vi "Results_file_Plotter.vi"() -> ()   [LabVIEW 2012]
uses:
  Anemometry/Anemometry Sub Vis/Data_plotting_vis/Plot_Slice.ctl
  Anemometry/Anemometry Sub Vis/Data_plotting_vis/Plotter_Mode.ctl
  Anemometry/Anemometry Sub Vis/Data_plotting_vis/Data_File_Type.ctl
  Anemometry/Anemometry Sub Vis/File/Setup_Filetype.ctl
  Anemometry/Anemometry Sub Vis/Controls/Global_mode.ctl
  Anemometry/Anemometry Sub Vis/Data_plotting_vis/Results_plotter_Global.vi
  Anemometry/Anemometry Sub Vis/Globals/Trav_pos_global.vi
  Instance           1 28Saved   Results_file_Plotter .vi
  Anemometry/Anemometry Sub Vis/Globals/Constants_global.vi
panel:
  out "Edit Raw DF?":bool
  in  "Tab Control":T1(tab)=enum."Save "
  in  "Template":path
  in  "Empty":bool
  in  "Result files to read":path[](array[path])
  in  "Add results file":bool
  in  "File Types to Read":T2
  in  "Vector Plot?":bool
  in  "Ordinate Name":string
  out "2nd Add label":string
  out "First Add label":string
  in  "Additional X Values":dbl[](array[numeric]) format="%.2f"
  in  "Additional Y Values":dbl[](array[numeric]) format="%.2f"
  in  "Show Results Space Analysis":bool
  in  "Show Plot Space Analysis":bool
  in  "Multi Ordinate":i32[](listbox)
  in  "Multi Ordinate?":bool
  in  "Ordinate":u16(ring) items=["Case", "File", "Source_Position X (mm)", "Receptor X (mm)", "Receptor Y (mm)", "Receptor Z (mm)", "C (ppm)", "c^2", "Q l/min", "CU/Q (m^{-2})", "Uref (m/s)", "Multi Run Start Time", "Bkgnd FF (C)", "Bkgnd Variance FF (C)", "Seconds since 1st Jan", "CU/Q Max Lat", "CU/Q Sig Y", "CU/Q Yo", "FF (C) Standard Error in Mean", "CU/Q Err", "Q Trace", "Drift%", "t (min)", "EnFlo Lab labstrat1 Delta T", "GMU Carrier 2 Gas", "Gas", "Source ID (mm)", "Emission Velocity m/s", "Emission Ratio", "FF (C) Standard Error in Variance", "GMU Source Type", "Aero_Tunnel Speed Meas Velocity", "Raw Data Filename", "Multi Run Row Number", "LDA X (mm)", "LDA Y (mm)", "LDA Z (mm)", "U", "u^2", "LDA (U) Standard Error in Mean", "W", "w^2", "LDA (W) Standard Error in Mean", "uw", "Av LDA Sampling Rate", "LDA (U) Standard Error in Variance", "u^2/U_{ref}^2", "w^2/U_{ref}^2", "-uw/U_{ref}^2", "U/Uref", "W/Uref", "LDA (U) & FF (C) Correlation uc", "LDA (W) & FF (C) Correlation wc", "Multi Run Row Type", "CU/Q (m^{-2}) Max Lat", "CU/Q (m^{-2}) Sig Y", "CU/Q (m^{-2}) Yo"]
  in  "Intensity Plot?":bool
  in  "Absisca":u16(ring) items=["Case", "File", "Source_Position X (mm)", "Receptor X (mm)", "Receptor Y (mm)", "Receptor Z (mm)", "C (ppm)", "c^2", "Q l/min", "CU/Q (m^{-2})", "Uref (m/s)", "Multi Run Start Time", "Bkgnd FF (C)", "Bkgnd Variance FF (C)", "Seconds since 1st Jan", "CU/Q Max Lat", "CU/Q Sig Y", "CU/Q Yo", "FF (C) Standard Error in Mean", "CU/Q Err", "Q Trace", "Drift%", "t (min)", "EnFlo Lab labstrat1 Delta T", "GMU Carrier 2 Gas", "Gas", "Source ID (mm)", "Emission Velocity m/s", "Emission Ratio", "FF (C) Standard Error in Variance", "GMU Source Type", "Aero_Tunnel Speed Meas Velocity", "Raw Data Filename", "Multi Run Row Number", "LDA X (mm)", "LDA Y (mm)", "LDA Z (mm)", "U", "u^2", "LDA (U) Standard Error in Mean", "W", "w^2", "LDA (W) Standard Error in Mean", "uw", "Av LDA Sampling Rate", "LDA (U) Standard Error in Variance", "u^2/U_{ref}^2", "w^2/U_{ref}^2", "-uw/U_{ref}^2", "U/Uref", "W/Uref", "LDA (U) & FF (C) Correlation uc", "LDA (W) & FF (C) Correlation wc", "Multi Run Row Type", "CU/Q (m^{-2}) Max Lat", "CU/Q (m^{-2}) Sig Y", "CU/Q (m^{-2}) Yo"]
  in  "Job Directory":path
  in  "Save Averaged rows":bool
  in  "Save Surface Fit":bool
  in  "Output Filename":path
  in  "Save Data in Rows":bool
  in  "Save Plot data":bool
  in  "Header":string
  in  "Process Point":bool
  in  "Kill Point":bool
  out "Table":string[][](table)
  in  "Post Process Plotted Data":bool
  in  "...using routine":string
  in  "Calculate new metadata":bool
  in  "Add /Edit metadata":bool
  in  "Delete Plotted data from file":bool
  in  "Save Setup":bool
  in  "Load Setup":bool
  in  "stop":bool
  out "Current":string="Graph Scales"
  in  "Single Series":i32[](listbox)=[0]
  in  "Edit Template File":bool
  in  "color and symbol":bool
  out "nRows":i32
  in  "Filter Bins 2":i32[](listbox)=[0]
  in  "Filter 6":u16(ring)
  in  "Filter 5":u16(ring)
  in  "Filter 4":u16(ring) items=["Show All (25)", "Lateral Profile (11)", "Vertical Profile (14)", "NOT Lateral Profile (14)", "NOT Vertical Profile (11)"]
  in  "Filter 3":u16(ring) items=["Show All (11)", "1 (11)", "NOT 1 (0)"]
  in  "Filter Array":u16[](array[ring])=[0, 0, 0, 0, 0, 0] items=["Don't Filter", "Case", "File", "Source_Position X (mm)", "Receptor X (mm)", "Receptor Y (mm)", "Receptor Z (mm)", "C (ppm)", "c^2", "Q l/min", "CU/Q (m^{-2})", "Uref (m/s)", "Multi Run Start Time", "Bkgnd FF (C)", "Bkgnd Variance FF (C)", "Seconds since 1st Jan", "CU/Q Max Lat", "CU/Q Sig Y", "CU/Q Yo", "FF (C) Standard Error in Mean", "CU/Q Err", "Q Trace", "Drift%", "t (min)", "EnFlo Lab labstrat1 Delta T", "GMU Carrier 2 Gas", "Gas", "Source ID (mm)", "Emission Velocity m/s", "Emission Ratio", "FF (C) Standard Error in Variance", "GMU Source Type", "Aero_Tunnel Speed Meas Velocity", "Raw Data Filename", "Multi Run Row Number", "LDA X (mm)", "LDA Y (mm)", "LDA Z (mm)", "U", "u^2", "LDA (U) Standard Error in Mean", "W", "w^2", "LDA (W) Standard Error in Mean", "uw", "Av LDA Sampling Rate", "LDA (U) Standard Error in Variance", "u^2/U_{ref}^2", "w^2/U_{ref}^2", "-uw/U_{ref}^2", "U/Uref", "W/Uref", "LDA (U) & FF (C) Correlation uc", "LDA (W) & FF (C) Correlation wc", "Multi Run Row Type", "CU/Q (m^{-2}) Max Lat", "CU/Q (m^{-2}) Sig Y", "CU/Q (m^{-2}) Yo"]
  in  "Filter Bins 1":i32[](listbox)=[0]
  in  "Create picture Vi Name":string caption="Picture VI:"
  in  "Save Plot as jpg":bool
  in  "Reload Files":bool
  out "Warning!":string
  out "XY Plot":cluster{dbl[], dbl[]}[](graph)
  out "Edit Raw Data Header Info":bool
  out "Raw DF in Orig Pos?":bool
  out "Intensity Graph":dbl[][](graph)
  in  "Bkgnd Value":dbl
  in  "Update":bool
  in  "Plot Resolution":bool
  in  "Point Size":i32(slide)=1 scale=0.0..10.0
  in  "No of Contours":i32=20
  in  "Slice mode":T3
  in  "Z Ch Name":u16(ring) items=["Case", "File", "Source_Position X (mm)", "Receptor X (mm)", "Receptor Y (mm)", "Receptor Z (mm)", "C (ppm)", "c^2", "Q l/min", "CU/Q (m^{-2})", "Uref (m/s)", "Multi Run Start Time", "Bkgnd FF (C)", "Bkgnd Variance FF (C)", "Seconds since 1st Jan", "CU/Q Max Lat", "CU/Q Sig Y", "CU/Q Yo", "FF (C) Standard Error in Mean", "CU/Q Err", "Q Trace", "Drift%", "t (min)", "EnFlo Lab labstrat1 Delta T", "GMU Carrier 2 Gas", "Gas", "Source ID (mm)", "Emission Velocity m/s", "Emission Ratio", "FF (C) Standard Error in Variance", "GMU Source Type", "Aero_Tunnel Speed Meas Velocity", "Raw Data Filename", "Multi Run Row Number", "LDA X (mm)", "LDA Y (mm)", "LDA Z (mm)", "U", "u^2", "LDA (U) Standard Error in Mean", "W", "w^2", "LDA (W) Standard Error in Mean", "uw", "Av LDA Sampling Rate", "LDA (U) Standard Error in Variance", "u^2/U_{ref}^2", "w^2/U_{ref}^2", "-uw/U_{ref}^2", "U/Uref", "W/Uref", "LDA (U) & FF (C) Correlation uc", "LDA (W) & FF (C) Correlation wc", "Multi Run Row Type", "CU/Q (m^{-2}) Max Lat", "CU/Q (m^{-2}) Sig Y", "CU/Q (m^{-2}) Yo"]
  in  "Y Ch Name":u16(ring) items=["Case", "File", "Source_Position X (mm)", "Receptor X (mm)", "Receptor Y (mm)", "Receptor Z (mm)", "C (ppm)", "c^2", "Q l/min", "CU/Q (m^{-2})", "Uref (m/s)", "Multi Run Start Time", "Bkgnd FF (C)", "Bkgnd Variance FF (C)", "Seconds since 1st Jan", "CU/Q Max Lat", "CU/Q Sig Y", "CU/Q Yo", "FF (C) Standard Error in Mean", "CU/Q Err", "Q Trace", "Drift%", "t (min)", "EnFlo Lab labstrat1 Delta T", "GMU Carrier 2 Gas", "Gas", "Source ID (mm)", "Emission Velocity m/s", "Emission Ratio", "FF (C) Standard Error in Variance", "GMU Source Type", "Aero_Tunnel Speed Meas Velocity", "Raw Data Filename", "Multi Run Row Number", "LDA X (mm)", "LDA Y (mm)", "LDA Z (mm)", "U", "u^2", "LDA (U) Standard Error in Mean", "W", "w^2", "LDA (W) Standard Error in Mean", "uw", "Av LDA Sampling Rate", "LDA (U) Standard Error in Variance", "u^2/U_{ref}^2", "w^2/U_{ref}^2", "-uw/U_{ref}^2", "U/Uref", "W/Uref", "LDA (U) & FF (C) Correlation uc", "LDA (W) & FF (C) Correlation wc", "Multi Run Row Type", "CU/Q (m^{-2}) Max Lat", "CU/Q (m^{-2}) Sig Y", "CU/Q (m^{-2}) Yo"]
  in  "X Ch Name":u16(ring) items=["Case", "File", "Source_Position X (mm)", "Receptor X (mm)", "Receptor Y (mm)", "Receptor Z (mm)", "C (ppm)", "c^2", "Q l/min", "CU/Q (m^{-2})", "Uref (m/s)", "Multi Run Start Time", "Bkgnd FF (C)", "Bkgnd Variance FF (C)", "Seconds since 1st Jan", "CU/Q Max Lat", "CU/Q Sig Y", "CU/Q Yo", "FF (C) Standard Error in Mean", "CU/Q Err", "Q Trace", "Drift%", "t (min)", "EnFlo Lab labstrat1 Delta T", "GMU Carrier 2 Gas", "Gas", "Source ID (mm)", "Emission Velocity m/s", "Emission Ratio", "FF (C) Standard Error in Variance", "GMU Source Type", "Aero_Tunnel Speed Meas Velocity", "Raw Data Filename", "Multi Run Row Number", "LDA X (mm)", "LDA Y (mm)", "LDA Z (mm)", "U", "u^2", "LDA (U) Standard Error in Mean", "W", "w^2", "LDA (W) Standard Error in Mean", "uw", "Av LDA Sampling Rate", "LDA (U) Standard Error in Variance", "u^2/U_{ref}^2", "w^2/U_{ref}^2", "-uw/U_{ref}^2", "U/Uref", "W/Uref", "LDA (U) & FF (C) Correlation uc", "LDA (W) & FF (C) Correlation wc", "Multi Run Row Type", "CU/Q (m^{-2}) Max Lat", "CU/Q (m^{-2}) Sig Y", "CU/Q (m^{-2}) Yo"]
  in  "Resolution":dbl=1.0 min=0.0 format="%.4f"
  out "Surface Area":dbl format="%^_6g"
  out "Surface Integral":dbl format="%^_6g"
  out "Surface Average":dbl format="%^#.6g"
  out "Uadvec":dbl
  in  "Full_Res_Results_Folder":path
  out "Last used Template":path
  out "Cursor index":i32
  out "Choosen Path":path
  in  "VI Refnum Calculation":refnum<vi>
  out "Filetype":string[](array[string])
  out "Mode":T4
  out "Plotted rows only?":bool
  in  "type specifier VI Refnum (for type only) 2":refnum<vi>
  in  "type specifier VI Refnum (for type only)":refnum<vi>
  out "Accept Array":bool[][](array[boolean])
  out "Previous slice mode":T3
  out "Slice mode Change?":bool
  out "Non-Blank Rows":bool[](array[boolean])
  out "File Index":i32
  out "Tolerances":dbl[](array[numeric]) format="%.2f"
  in  "Results files choosen":path[](array[path])
  in  "Transpose":bool
  out "Plotted Series":bool[][](array[boolean])
  in  "Results file":path
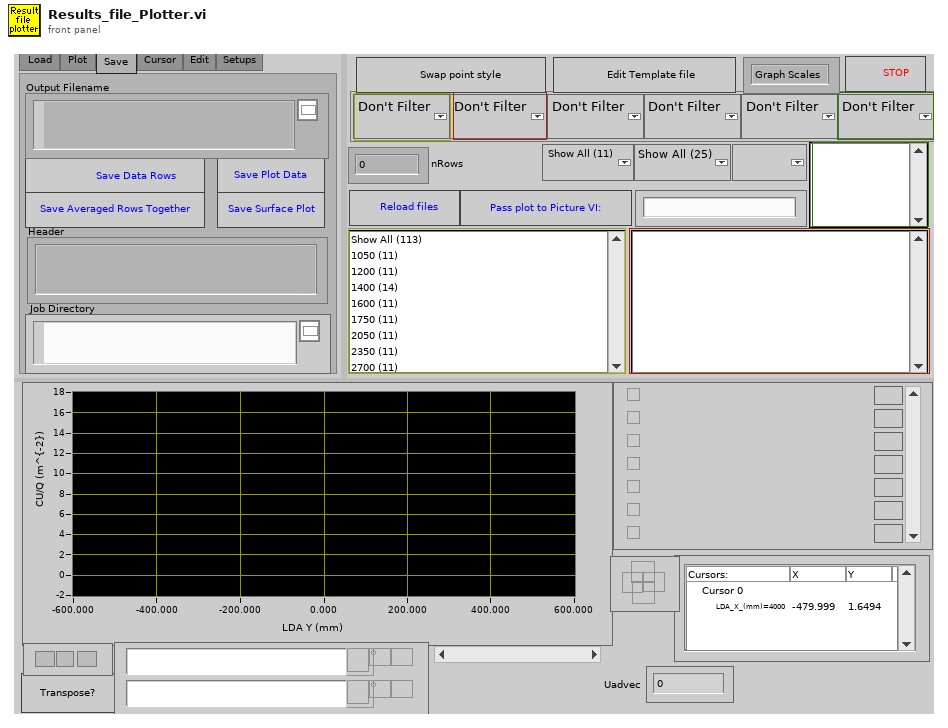
[diagram p1: front panel]
types:
  T1 = enum32{"Load ", "Plot ", "Save ", "Cursor", "Edit", "Setups"}
  T2 = typedef "Data_File_Type.ctl" = enum16{"Read All File Types", "Results Files Only", "Raw Data Files Only", "Calibration Files Only", "Gas Desk Files Only", "Old Results Files Only", "Tabulated Data Files Only"}
  T3 = typedef "Plot_Slice.ctl" = enum16{"XY Slice (Plan)", "YX Slice (Plan)", "YZ Slice (Cross)", "ZY Slice (Cross)", "XZ Slice (Side)", "ZX Slice (Side)"}
  T4 = typedef "Plotter_Mode.ctl" = enum16{"Save file", "Delete unwanted rows", "Edit Values with constants", "Edit values per row", "Edit Raw Data file header", "Post Process Plotted Rows"}
  T5 = typedef "Setup_Filetype.ctl" = enum16{"Measurement Setups", "Calibration Setups", "General", "Results File Plotter Setups", "Speed Calib Tweaks"}
  T6 = enum16{"Zero or one", "One", "Zero or more", "One or more"}
  T7 = typedef "Global_mode.ctl" = enum16{"Read Global", "Load Global From File", "Write Global to File"}
  T8 = enum16{"Edit Existing Template File", "Create New Template File"}
  T9 = enum16{"Show only data summary", "Show data summary", "No data summary"}
  T10 = typedef "All_Setup.ctl" = cluster{"Result files to read":path[], "Template":path, "Transpose":bool, "Additional X Values":dbl[], "Additional Y Values":dbl[], "Ordinate":u16, "Absisca":u16, "Filter Array":u16[], "color and symbol":bool, "Output Filename":path, "Jpg Vi Name":string, "Intensity Plot?":bool, "Multi Ordinate?":bool, "Filter Bins 1":i32[], "Filter Bins 2":i32[], "Multi Ordinate":i32[]}
  T11 = enum16{"Left Button", "Center Button", "Right Button", "Window Close"}
  T12 = enum32{"existing file", "new file", "new or existing file", "existing dir", "new dir", "new or existing dir", "existing file (use LLBs)", "new file (use LLBs)", "new or existing file (use LLBs)", "new or existing file or directory (use LLBs)"}
  T13 = cluster{"Plot Color":u32, "Plot Interpolation":u8, "Point Style":u8, "Line Style":u8, "Fill/Pt. Color":u32, "Line Width":u8, "Bar Plot Style":u8, "Fill To":i16}[]
  T14 = typedef "Group_Binning.ctl" = cluster{"Index":i32, "Tolerance":dbl, "Precision":string}
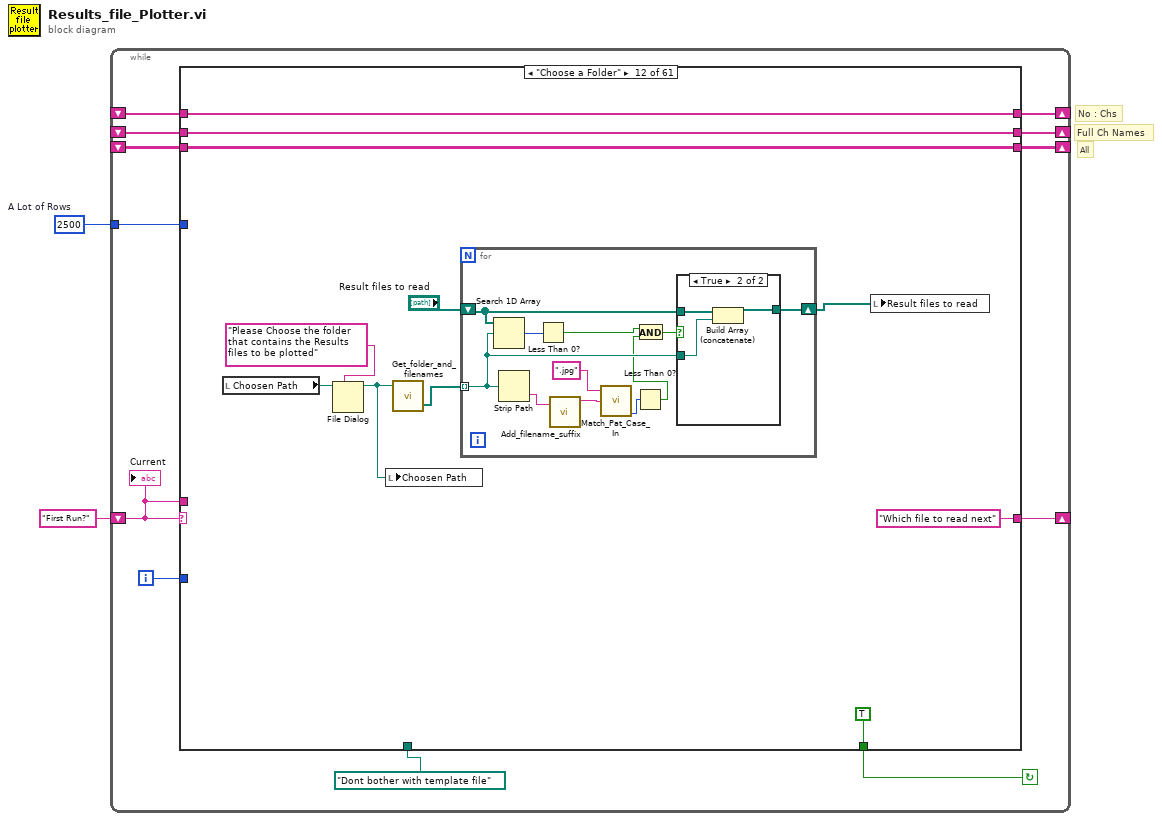
[diagram p0: block diagram]
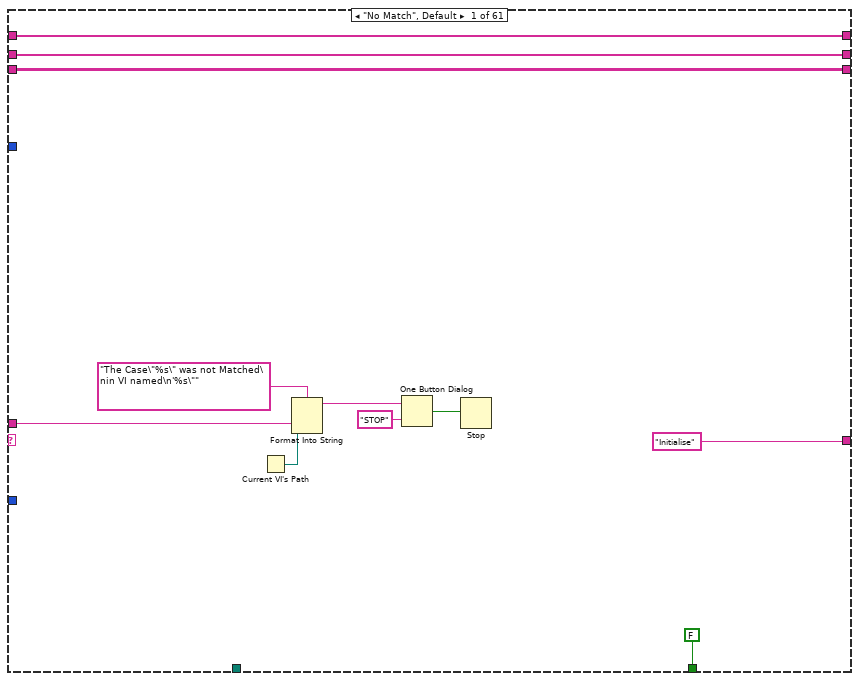
[diagram p2: hidden frame]
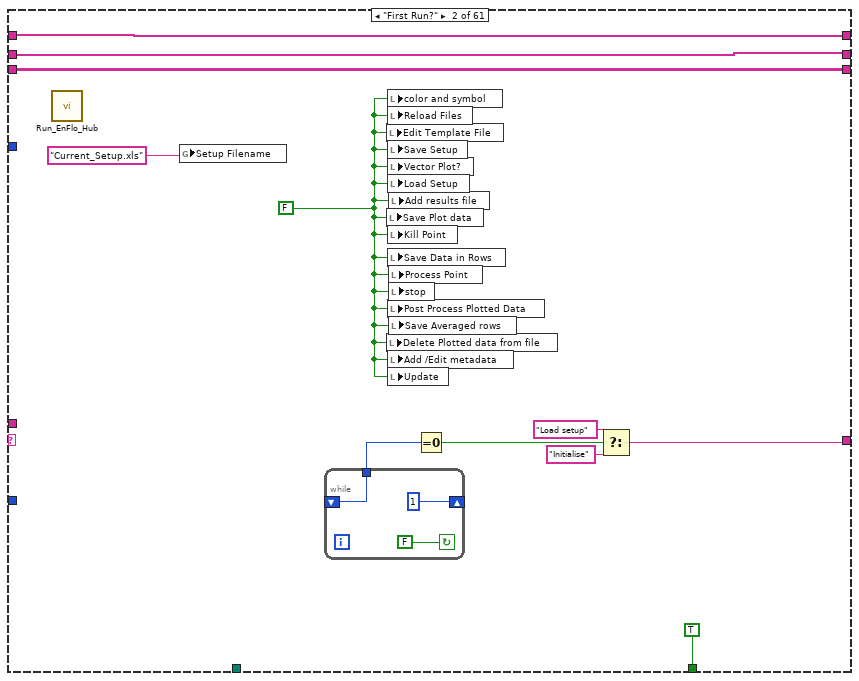
[diagram p3: hidden frame]
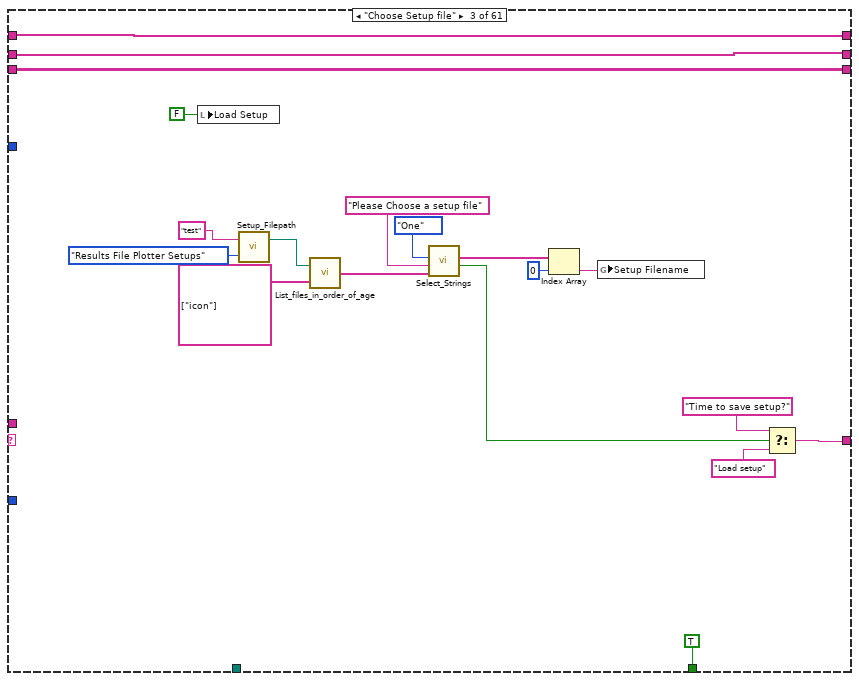
[diagram p4: hidden frame]
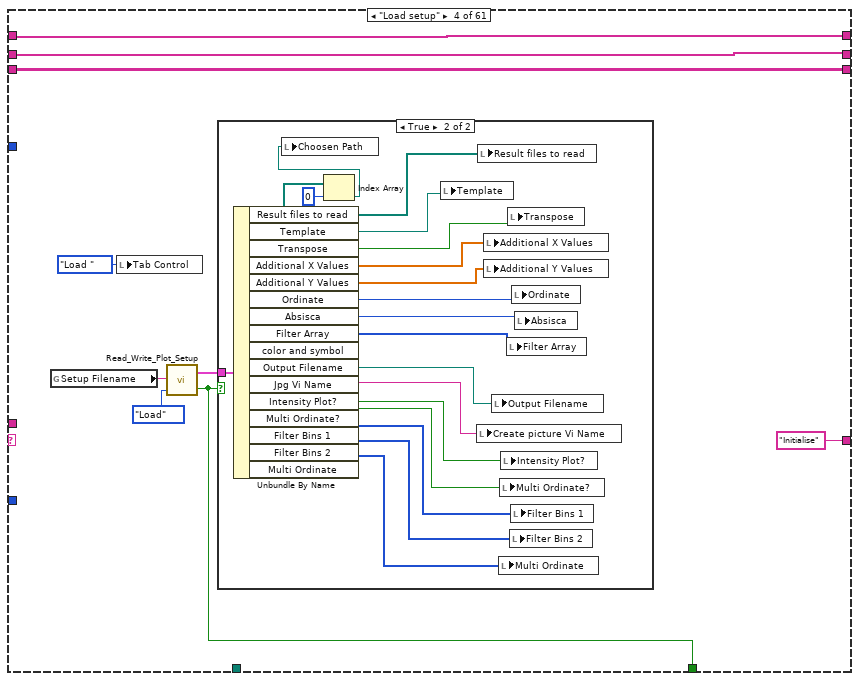
[diagram p5: hidden frame]
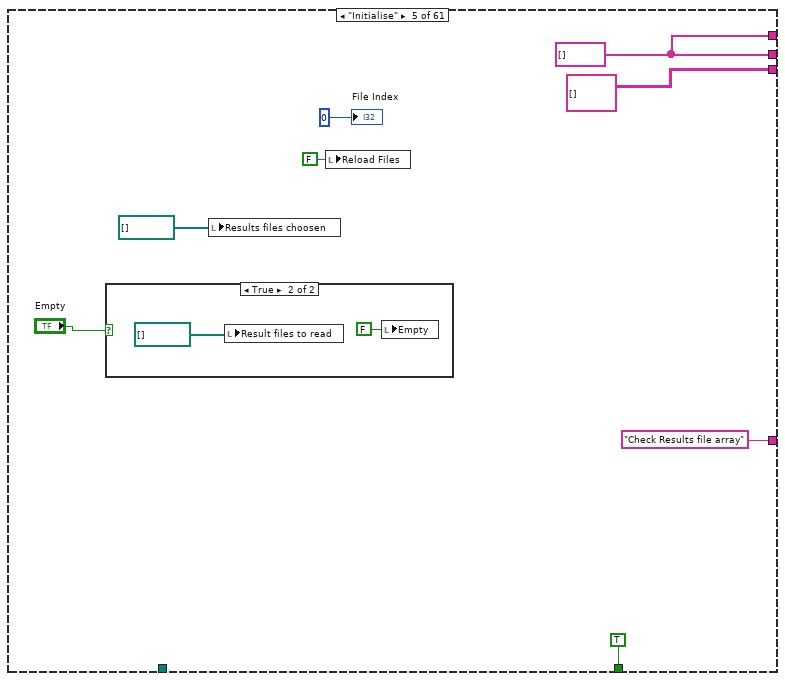
[diagram p7: hidden frame]
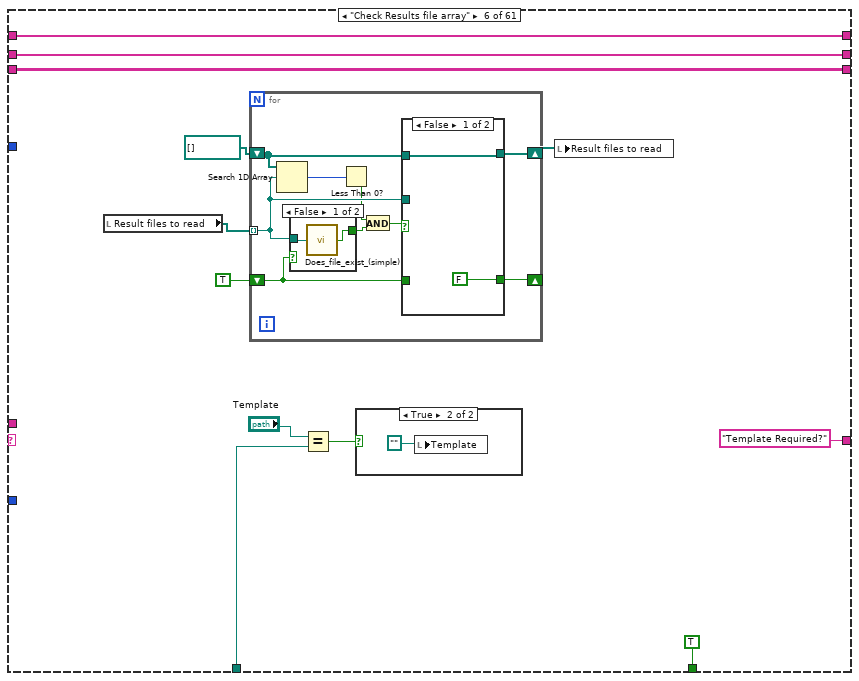
[diagram p9: hidden frame]
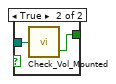
[diagram p11: hidden frame]
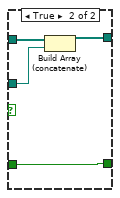
[diagram p12: hidden frame]
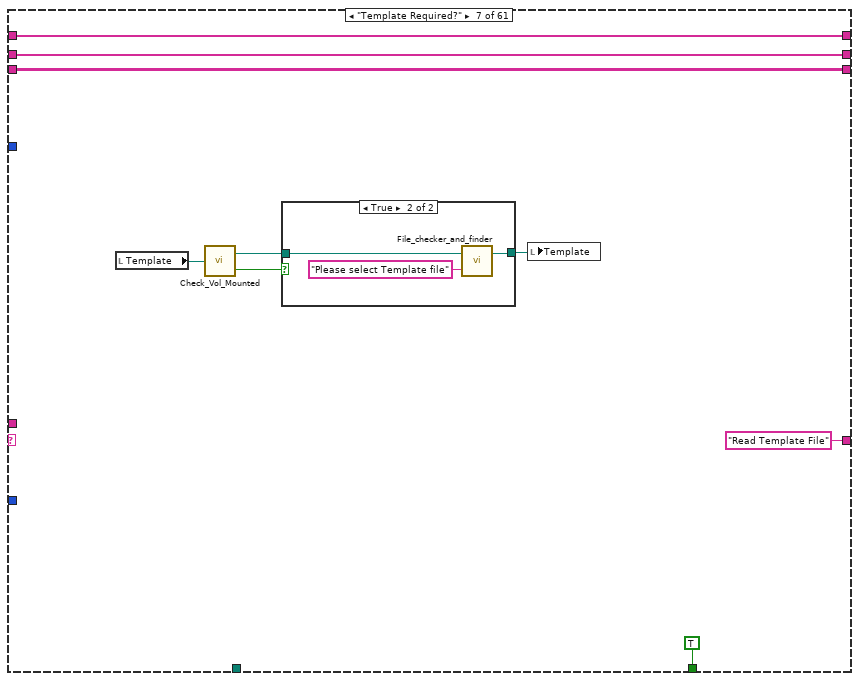
[diagram p13: hidden frame]
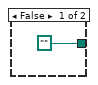
[diagram p14: hidden frame]
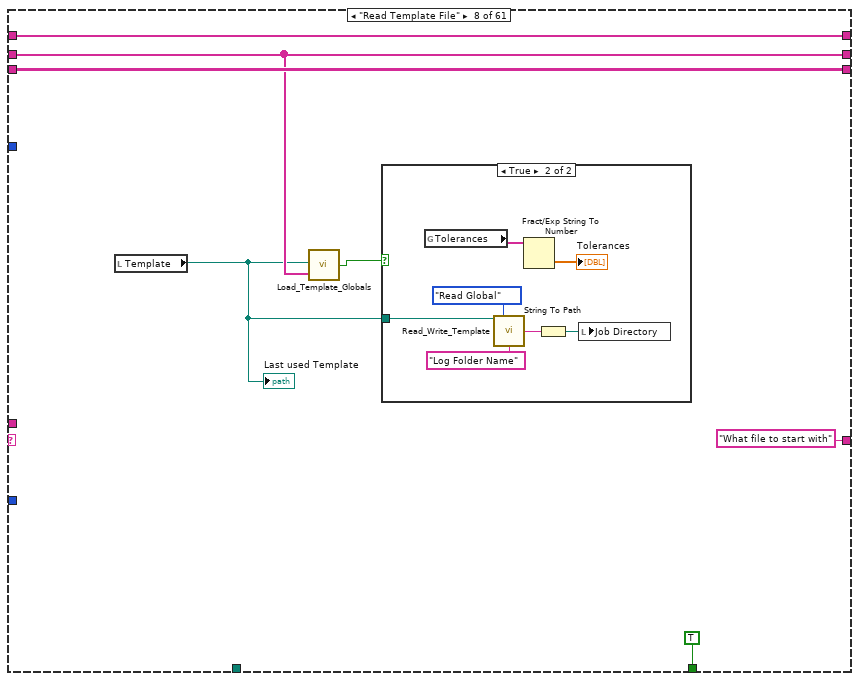
[diagram p15: hidden frame]
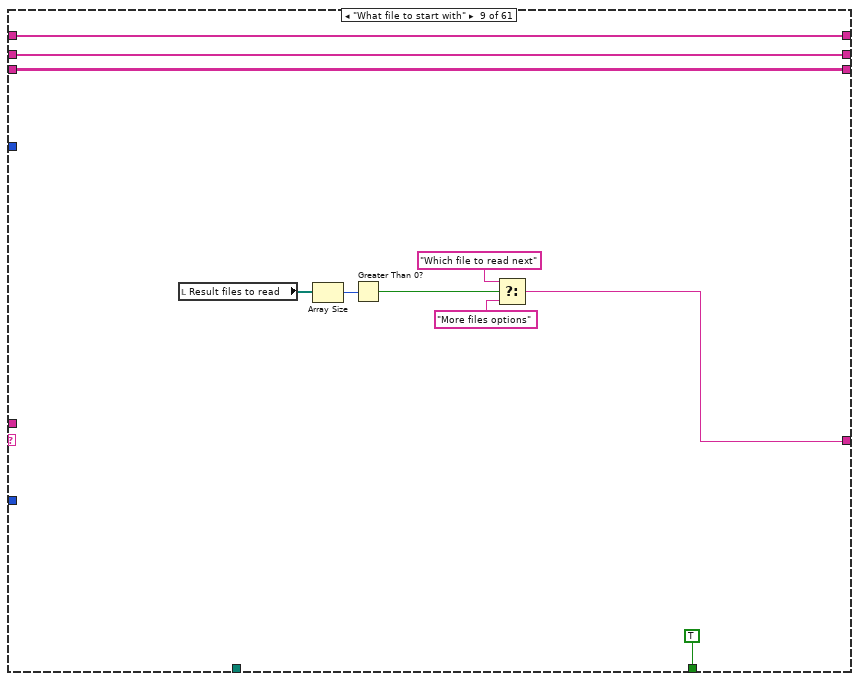
[diagram p17: hidden frame]
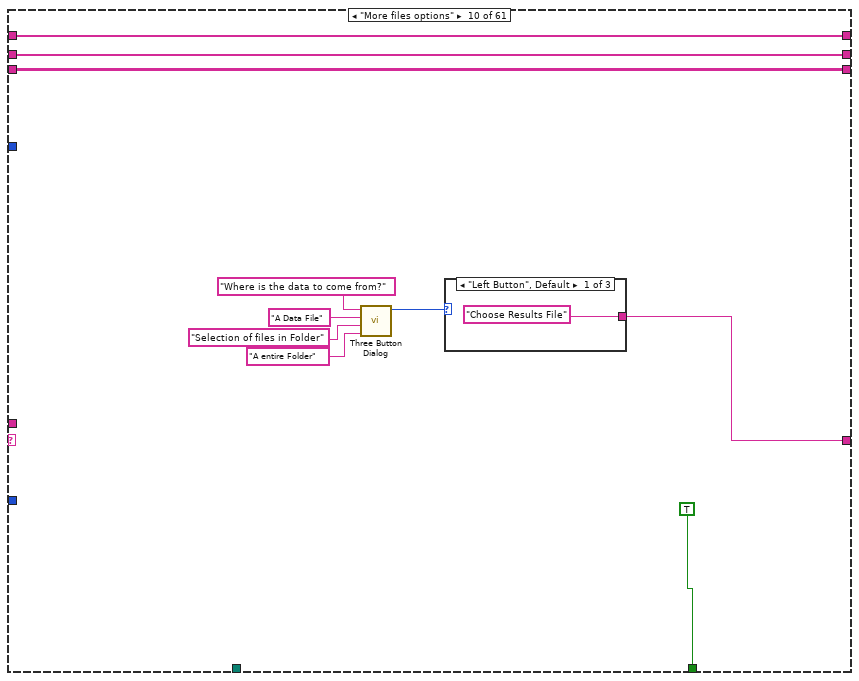
[diagram p18: hidden frame]
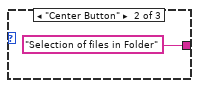
[diagram p19: hidden frame]
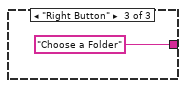
[diagram p20: hidden frame]
diagram:
  w1 = 2500  # A Lot of Rows
  # "No : Chs"
  # "Full Ch Names"
  # "All"
  n1 = while {
    shift-left: _ -> [w7]
    shift-right: [w8] -> _
    shift-left: "First Run?" -> [w11]
    shift-right: [w4] -> _
    shift-left: _ -> [w9]
    shift-right: [w14] -> _
    shift-left: _ -> [w12]
    shift-right: [w5] -> _
    tunnel: w1 -> [w3]
    i -> [w6]
    stop <- w13 continue-if-true
    n2 = case shown="\"Choose a Folder\"" w11 {
      tunnel: w9 -> [w25 w35 w57 w65 _ w106 w134 w143 w164 w174 w186 w200 w231 w258 w281 w403 w425 w451 w476 w502 w556 w570 w607 w909 w978 w1033 w1058 w1077 w1163 w1214 w1244 w1533 w1549 w1570 w1599 w1663 w1696 w1771 w1794 w1809 w1873 w1925 w1951 w2160 w2172 w2198 w2324 w2468 w2502 w2517 w2542 w2569 w2612 w2630 w2673 w2776 w2809 w3164 w3179 w3215 w3223]
      tunnel: [w25 w35 w57 w65 w91 w106 w134 w143 w164 w174 w186 w200 w231 w258 w279 w403 w425 w451 w476 w502 w556 w570 w607 w909 w978 w1033 w1058 w1077 w1163 w1214 w1242 w1533 w1549 w1570 w1599 w1663 w1696 w1771 w1794 w1809 w1873 w1925 w1949 w2160 w2172 w2196 w2317 w2468 w2502 w2517 w2542 w2569 w2612 w2630 w2673 w2776 w2809 w3164 w3179 w3215 w3223] -> w14
      tunnel: ["Initialise" w28 w52 "Initialise" ("t") "Check Results file array" ("t") "Template Required?" "Read Template File" "What file to start with" w155 w170 "Which file to read next" "Which file to read next" "Which file to read next" w254 w276 w394 "What is present?" "Ordinate Selector Type" w473 "Which rows are Non-Blank?" w549 "Create Selectors" w596 "Re Plot Data?" w973 "Prepare Filter2 strings" "Plot Data" w1074 "Add Axis names" "Analyse Plot Space" w1245 "What to do next?" "What to do next?" ("t") w1556 w1592 w1641 w1694 w1765 w1790 w1808 w1872 "Initialise" w1952 w2151 "Create Selectors" w2199 w2325 w2466 w2500 w2507 w2526 "Save XY plot as jpg" "Create Selectors" w2627 w2676 w2760 w2815 "Save Setup" ("t") "Initialise" ("t") w3184 "Time to save setup?"] -> w4
      tunnel: [FALSE TRUE TRUE w61 TRUE TRUE TRUE TRUE TRUE TRUE TRUE TRUE TRUE w249 w283 TRUE TRUE TRUE TRUE TRUE TRUE TRUE TRUE TRUE TRUE TRUE TRUE w1075 TRUE TRUE w1246 TRUE TRUE ("OK?") TRUE TRUE ("OK?") TRUE ("OK?") w1692 TRUE TRUE w1807 w1871 TRUE w1953 TRUE ("OK?") TRUE ("OK?") w2200 w2326 TRUE TRUE TRUE TRUE TRUE TRUE TRUE TRUE TRUE TRUE TRUE TRUE w3193 TRUE ("OK?")] -> w13
      tunnel: w12 -> [w24 w34 w56 w64 _ w105 w133 w145 w163 w173 w185 w199 w230 w257 w282 w399 w424 w452 w477 w503 w555 w568 w602 w911 w967 w1035 w1060 w1076 w1165 w1216 w1243 w1532 w1548 w1569 w1610 w1662 w1695 w1770 w1793 w1806 w1870 w1924 w1950 w2159 w2169 w2197 w2323 w2469 w2501 w2516 w2546 w2572 w2611 w2629 w2672 w2775 w2808 w3163 w3178 w3214 w3222]
      tunnel: w11 -> [w16 _ _ _ _ _ _ _ _ _ _ _ _ _ _ _ _ _ _ _ _ _ _ _ _ _ _ _ _ _ _ _ _ _ _ _ _ _ _ _ _ _ _ _ _ _ _ _ _ _ _ _ _ _ _ _ _ _ _ _ _]
      tunnel: path "Dont bother with template file" ("Template File") -> [_ _ _ _ _ w99 _ _ _ _ _ _ _ _ _ _ _ _ _ _ _ _ _ _ _ _ _ _ _ _ _ _ _ _ _ _ _ _ _ _ _ _ _ _ _ _ _ _ _ _ _ _ _ _ _ _ _ w3161 w3173 _ _]
      tunnel: [w15 w33 w55 w66 w91 w104 w132 w144 w161 w171 w183 w197 w228 w256 w278 w387 w423 w453 w475 w501 w547 w569 w600 w908 w969 w1026 w1053 w1073 w1157 w1209 w1238 w1529 w1550 w1568 w1600 w1664 w1697 w1769 w1792 w1805 w1869 w1923 w1943 w2161 w2177 w2187 w2320 w2478 w2503 w2518 w2543 w2570 w2613 w2631 w2677 w2777 w2816 w3165 w3180 w3216 w3224] -> w8
      tunnel: w7 -> [w15 w33 w55 w66 _ w104 w132 w144 w161 w171 w183 w197 w228 w256 w277 w387 w423 w453 w475 w501 w547 w569 w600 w908 w969 w1026 w1053 w1073 w1157 w1209 w1237 w1529 w1550 w1568 w1600 w1664 w1697 w1769 w1792 w1805 w1869 w1923 w1942 w2161 w2177 w2191 w2319 w2478 w2503 w2518 w2543 w2570 w2613 w2631 w2677 w2777 w2816 w3165 w3180 w3216 w3224]
      tunnel: w6 -> [_ _ _ _ _ _ _ _ _ _ _ _ _ _ _ _ _ _ _ _ _ _ _ _ _ _ _ _ _ _ _ _ _ _ _ _ w1693 _ _ _ _ _ _ _ _ _ _ _ _ _ _ _ _ _ _ _ _ _ _ _ _]
      tunnel: [w24 w34 w56 w64 string[][] [] w105 w133 w145 w163 w173 w185 w199 w230 w257 w280 w399 w424 w452 w477 w503 w555 w568 w602 w911 w967 w1035 w1060 w1076 w1165 w1216 w1241 w1532 w1548 w1569 w1610 w1662 w1695 w1770 w1793 w1806 w1870 w1924 w1948 w2159 w2169 w2195 w2316 w2469 w2501 w2516 w2546 w2572 w2611 w2629 w2672 w2775 w2808 w3163 w3178 w3214 w3222] -> w5
      tunnel: w3 -> [_ _ _ _ _ _ _ _ _ _ _ _ _ _ _ _ _ _ _ _ _ _ _ _ _ _ _ _ _ _ _ _ _ _ _ _ _ _ w1788 _ w1868 _ _ _ _ _ _ _ _ _ _ _ _ w2626 w2670 _ w2806 _ _ _ _]
      frame "No Match", Default {
        n3 = Current VI's Path() -> (path=w17:path)
        n4 = Format Into String(format string="The Case\"%s\" was not Matched\nin VI named\n'%s\"" ("Format String"), w16, w17) -> (resulting string=w20:string)  [unwired: 2 in, 1 out]
        n5 = One Button Dialog(message=w20, button name ("OK")="STOP") -> (true=w18:bool)
        n6 = Stop(stop? (T)=w18) -> ()
      }
      frame "First Run?" {
        w26 = FALSE ("Save Plot data")
        n7 = call "Run_EnFlo_Hub.vi"() -> ()  [unwired: 8 out]
        n8 = global write "Results_plotter_Global.vi" "Setup Filename"("Current_Setup.xls" ("Setup filename")) -> ()
        n9 = while {
          shift-right: [1] -> _
          shift-left: _ -> [w38]
          tunnel: [w38] -> w30
          stop <- FALSE continue-if-true
        }
        n10 = local write "Edit Template File"(w26) -> ()
        n11 = local write "Save Plot data"(w26) -> ()
        n12 = local write "Delete Plotted data from file"(w26) -> ()
        n13 = local write "color and symbol"(w26) -> ()
        n14 = local write "Reload Files"(w26) -> ()
        n15 = local write "Save Setup"(w26) -> ()
        n16 = local write "Vector Plot?"(w26) -> ()
        n17 = local write "Load Setup"(w26) -> ()
        n18 = local write "Kill Point"(w26) -> ()
        n19 = local write "Save Data in Rows"(w26) -> ()
        n20 = local write "Post Process Plotted Data"(w26) -> ()
        n21 = local write "Add /Edit metadata"(w26) -> ()
        n22 = local write "Update"(w26) -> ()
        n23 = local write "Add results file"(w26) -> ()
        n24 = local write "Process Point"(w26) -> ()
        n25 = local write "stop"(w26) -> ()
        n26 = local write "Save Averaged rows"(w26) -> ()
        n27 = Equal To 0?(x=w30) -> (x = 0?=w29:bool)
        n28 = Select(t="Load setup", s=w29, f="Initialise") -> (s? t:f=w28:string)
      }
      frame "Choose Setup file" {
        n29 = local write "Load Setup"(FALSE ("Save Setup")) -> ()
        n30 = call "Setup_Filepath.vi"("Setup File Type"=Setup_Filetype."Results File Plotter Setups", "Filename in"="test") -> ("Directory"=w40:path)  [unwired: 1 out]
        n31 = call "List_files_in_order_of_age.vi"("Files to Hide"=string[] ["icon"], "Folder"=w40) -> ("file names"=w51:string[])
        n32 = call "Select_Strings.vi"("Available Ch names"=w51, "Message"="Please Choose a setup file", "Selector mode"=T6."One") -> ("Cancel"=w45:bool, "Selected Channel Names"=w48:string[])  [unwired: 1 in, 3 out]
        n33 = Index Array(array=w48, index=0) -> (element=w46:string)
        n34 = global write "Results_plotter_Global.vi" "Setup Filename"(w46) -> ()
        n35 = Select(t="Time to save setup?", s=w45, f="Load setup") -> (s? t:f=w52:string)
      }
      frame "Load setup" {
        n36 = global read "Results_plotter_Global.vi" "Setup Filename"() -> (w60:string)
        n37 = local write "Tab Control"(T1."Load " ("Tab Control")) -> ()
        n38 = call "Read_Write_Plot_Setup.vi"("Mode"=enum16{"Load", "Save"}."Load", "Setup filename"=w60) -> ("OK?"=w61:bool, "Cluster 2"=w62:T10)  [unwired: 1 in]
        n39 = case shown="True" w61 {
          tunnel: w62 -> [_ w85]
          frame False {
          }
          frame True {
            n40 = Unbundle By Name(w85) -> ("Result files to read"=w70:path[], "Template"=w68:path, "Transpose"=w75:bool, "Additional X Values"=w76:dbl[], "Additional Y Values"=w77:dbl[], "Ordinate"=w78:u16, "Absisca"=w79:u16, "Filter Array"=w80:u16[], "Output Filename"=w81:path, "Jpg Vi Name"=w82:string, "Intensity Plot?"=w83:bool, "Multi Ordinate?"=w84:bool, "Filter Bins 1"=w74:i32[], "Filter Bins 2"=w73:i32[], "Multi Ordinate"=w72:i32[])  [unwired: 1 out]
            n41 = Index Array(array=w70, index=0) -> (element=w69:path)
            n42 = local write "Choosen Path"(w69) -> ()
            n43 = local write "Template"(w68) -> ()
            n44 = local write "Create picture Vi Name"(w82) -> ()
            n45 = local write "Result files to read"(w70) -> ()
            n46 = local write "Additional X Values"(w76) -> ()
            n47 = local write "Additional Y Values"(w77) -> ()
            n48 = local write "Output Filename"(w81) -> ()
            n49 = local write "Multi Ordinate"(w72) -> ()
            n50 = local write "Multi Ordinate?"(w84) -> ()
            n51 = local write "Intensity Plot?"(w83) -> ()
            n52 = local write "Filter Array"(w80) -> ()
            n53 = local write "Transpose"(w75) -> ()
            n54 = local write "Filter Bins 2"(w73) -> ()
            n55 = local write "Filter Bins 1"(w74) -> ()
            n56 = local write "Ordinate"(w78) -> ()
            n57 = local write "Absisca"(w79) -> ()
          }
        }
      }
      frame "Initialise" {
        w91 = string[] [] ("Channel names")
        n58 = case shown="True" "Empty" {
          frame False {
          }
          frame True {
            n59 = local write "Result files to read"(path[] [] ("Result files to read")) -> ()
            n60 = local write "Empty"(FALSE ("Empty")) -> ()
          }
        }
        n61 = local write "Results files choosen"(path[] [] ("Results file choosen")) -> ()
        n62 = local write "Reload Files"(FALSE ("Reload Files")) -> ()
        "File Index" <- 0
      }
      frame "Check Results file array" {
        n63 = local read "Result files to read"() -> (w103:path[])
        n64 = for {
          shift-right: [w117] -> w101
          shift-left: path[] [] -> [w116]
          tunnel: w103 -> [w115] mode=indexing
          shift-right: [w110] -> _
          shift-left: TRUE -> [w109]
          n65 = Search 1D Array(1D array=w116, element=w115) -> (index of element=w114:i32)  [unwired: 1 out]
          n66 = case shown="False" w109 {
            tunnel: w115 -> [w119 w121]
            tunnel: [w118 w120] -> w112
            frame False {
              n67 = call "Does_file_exist_(simple).vi"("Pathname"=w119) -> ("exists?"=w118:bool)
            }
            frame True {
              n68 = call "Check_Vol_Mounted.vi"("Filename"=w121) -> ("exists?"=w120:bool)  [unwired: 1 out]
            }
          }
          n69 = Less Than 0?(x=w114) -> (x < 0?=w111:bool)
          n70 = And(x=w111, y=w112) -> (x .and. y?=w113:bool)
          n71 = case shown="False" w113 {
            tunnel: w116 -> [w123 w127]
            tunnel: w115 -> [_ w126]
            tunnel: [w123 w125] -> w117
            tunnel: [FALSE w124] -> w110
            tunnel: w109 -> [_ w124]
            frame False {
            }
            frame True {
              n72 = Build Array (concatenate)(w127, w126) -> (w125:path[])
            }
          }
        }
        n73 = Equal?(x="Template", y=w99) -> (x = y?=w98:bool)
        n74 = case shown="True" w98 {
          frame False {
          }
          frame True {
            n75 = local write "Template"(path "") -> ()
          }
        }
        n76 = local write "Result files to read"(w101) -> ()
      }
      frame "Template Required?" {
        n77 = local read "Template"() -> (w131:path)
        n78 = call "Check_Vol_Mounted.vi"("Filename"=w131) -> ("Filename Out"=w130:path, "exists?"=w129:bool)
        n79 = case shown="True" w129 {
          tunnel: w130 -> [_ w139]
          tunnel: [path "" w138] -> w128
          frame False {
          }
          frame True {
            n80 = call "File_checker_and_finder.vi"("Promp if not found"="Please select Template file", "Filename In"=w139) -> ("Filename Out"=w138:path)  [unwired: 1 out]
          }
        }
        n81 = local write "Template"(w128) -> ()
      }
      frame "Read Template File" {
        n82 = local read "Template"() -> (w141:path)
        "Last used Template" <- w141
        n83 = call "Load_Template_Globals.vi"("Channel Names"=w143, "Template-read"=w141) -> ("Valid Template File?"=w142:bool)
        n84 = case shown="True" w142 {
          tunnel: w141 -> [_ w149]
          frame False {
          }
          frame True {
            n85 = global read "Results_plotter_Global.vi" "Tolerances"() -> (w153:string[])
            n86 = call "Read_Write_Template.vi"("Template File"=w149, "Mode"=Global_mode."Read Global", "Data type"="Log Folder Name" ("Variable name")) -> ("Single Value Out"=w151:string)  [unwired: 5 in, 7 out]
            n87 = Fract/Exp String To Number(string=w153) -> (number=→"Tolerances":dbl[])  [unwired: 4 out]
            n88 = String To Path(string=w151) -> (path=w148:path)
            n89 = local write "Job Directory"(w148) -> ()
          }
        }
      }
      frame "What file to start with" {
        n90 = local read "Result files to read"() -> (w160:path[])
        n91 = Array Size(array=w160) -> (size(s)=w159:i32)
        n92 = Greater Than 0?(x=w159) -> (x > 0?=w156:bool)
        n93 = Select(t="Which file to read next", s=w156, f="More files options") -> (s? t:f=w155:string)
      }
      frame "More files options" {
        n94 = call <vilib>:"Three Button Dialog.vi"("Right Button Text (\"Cancel\")"="A entire Folder" ("F button name (\"Cancel\")"), "Center Button Text (\"No\")"="Selection of files in Folder" ("T button name (\"OK\")"), "Left Button Text (\"Yes\")"="A Data File" ("T button name (\"OK\")"), "message"="Where is the data to come from?") -> ("Which Button?"=w169:T11)  [unwired: 1 in, 6 out]
        n95 = case shown="\"Left Button\", Default" w169 {
          tunnel: ["Choose Results File" "Selection of files in Folder" "Choose a Folder"] -> w170
          frame "Left Button", Default {
          }
          frame "Center Button" {
          }
          frame "Right Button" {
          }
        }
      }
      frame "Choose Results File" {
        (unwired) T12."existing file" ("select mode (2)")
        n96 = local read "Choosen Path"() -> (w178:path)
        n97 = File Dialog(7:"Please Choose a Results File" ("Promp if not found"), 11:w178) -> (1:w180:bool, 3:w179:path)  [unwired: 1 in, 6 out]
        "Choosen Path" <- w179
        n98 = case shown="False" w180 {
          tunnel: w179 -> [w187 _]
          frame False {
            n99 = local read "Result files to read"() -> (w188:path[])
            n100 = Build Array (concatenate)(w188, w187) -> (w189:path[])
            n101 = local write "Result files to read"(w189) -> ()
          }
          frame True {
          }
        }
      }
      frame "Choose a Folder" {
        n102 = local read "Choosen Path"() -> (w191:path)
        n103 = File Dialog(7:"Please Choose the folder that contains the Results files to be plotted" ("prompt"), 11:w191) -> (3:w190:path)  [unwired: 1 in, 7 out]
        n104 = local write "Choosen Path"(w190) -> ()
        n105 = call "Get_folder_and_filenames.vi"("file path (dialog if empty)"=w190) -> ("Files"=w192:path[])  [unwired: 1 out]
        n106 = for {
          shift-right: [w211] -> w193
          shift-left: "Result files to read" -> [w210]
          tunnel: w192 -> [w208] mode=indexing
          n107 = Search 1D Array(1D array=w210, element=w208) -> (index of element=w209:i32)  [unwired: 1 out]
          n108 = Strip Path(path=w208) -> (name=w207:string)  [unwired: 1 out]
          n109 = Less Than 0?(x=w209) -> (x < 0?=w206:bool)
          n110 = call "Add_filename_suffix.vi"("Filename"=w207) -> ("Original Suffix"=w204:string)  [unwired: 1 in, 3 out]
          n111 = call "Match_Pat_Case_In.vi"("String to match"=".jpg" ("x"), "String"=w204) -> ("offset past match"=w202:i32)  [unwired: 1 in, 3 out]
          n112 = Less Than 0?(x=w202) -> (x < 0?=w201:bool)
          n113 = And(x=w206, y=w201) -> (x .and. y?=w205:bool)
          n114 = case shown="True" w205 {
            tunnel: w210 -> [w212 w215]
            tunnel: w208 -> [_ w214]
            tunnel: [w212 w213] -> w211
            frame False {
            }
            frame True {
              n115 = Build Array (concatenate)(w215, w214) -> (w213:path[])
            }
          }
        }
        n116 = local write "Result files to read"(w193) -> ()
      }
      frame "Selection of files in Folder" {
        n117 = local read "Choosen Path"() -> (w217:path)
        n118 = local read "Result files to read"() -> (w220:path[])
        n119 = File Dialog(7:"Please Choose the folder that contains the Results files to be plotted" ("prompt"), 11:w217) -> (3:w216:path)  [unwired: 1 in, 7 out]
        n120 = call "Get_folder_and_filenames.vi"("file path (dialog if empty)"=w216) -> ("Files"=w222:path[])  [unwired: 1 out]
        n121 = local write "Choosen Path"(w216) -> ()
        n122 = for {
          tunnel: w222 -> [w245] mode=indexing
          tunnel: [w244] -> w225 mode=indexing
          n123 = Strip Path(path=w245) -> (name=w244:string)  [unwired: 1 out]
        }
        n124 = call "Select_Strings.vi"("Available Ch names"=w225, "Message"="Please select the desired data files", "Selector mode"=T6."Zero or more") -> ("Ch Indicies Choosen"=w223:i32[])  [unwired: 1 in, 4 out]
        n125 = for {
          tunnel: w223 -> [w243] mode=indexing
          tunnel: w222 -> [w242]
          tunnel: [w241] -> w218 mode=indexing
          n126 = Index Array(array=w242, index=w243) -> (element=w241:path)
        }
        n127 = for {
          shift-right: [w236] -> w219
          shift-left: w220 -> [w235]
          tunnel: w218 -> [w234] mode=indexing
          n128 = Search 1D Array(1D array=w235, element=w234) -> (index of element=w233:i32)  [unwired: 1 out]
          n129 = Less Than 0?(x=w233) -> (x < 0?=w232:bool)
          n130 = case shown="True" w232 {
            tunnel: w235 -> [w237 w240]
            tunnel: w234 -> [_ w239]
            tunnel: [w237 w238] -> w236
            frame False {
            }
            frame True {
              n131 = Build Array (concatenate)(w240, w239) -> (w238:path[])
            }
          }
        }
        n132 = local write "Result files to read"(w219) -> ()
      }
      frame "Which file to read next" {
        n133 = local read "Result files to read"() -> (w255:path[])
        n134 = local read "File Index"() -> (w252:i32)
        n135 = Array Size(array=w255) -> (size(s)=w253:i32)
        n136 = Equal?(x=w253, y=w252) -> (x = y?=w251:bool)
        n137 = case shown="False" w251 {
          tunnel: w255 -> [w261 _]
          tunnel: [w262 "Load Selectors"] -> w254
          tunnel: w252 -> [w260 w274]
          tunnel: [w259 w274] -> w247
          frame False {
            n138 = Index Array(array=w261, index=w260) -> (element=w263:path)
            n139 = Search 1D Array(1D array="Results files choosen", element=w263) -> (index of element=w265:i32)  [unwired: 1 out]
            n140 = call "Add_filename_suffix.vi"() -> ()  [unwired: 2 in, 4 out]
            n141 = case shown="-1" w265 {
              tunnel: "Results files choosen" -> [_ w273]
              tunnel: w263 -> [w269 w272]
              tunnel: ["Which file to read next" "Load Data"] -> w262
              frame 0, Default {
                n142 = Format Into String(format string="The filename\n \"%s\"\n has already been chosen" ("Format String"), w269) -> (resulting string=w267:string)  [unwired: 2 in, 1 out]
                n143 = One Button Dialog(message=w267) -> ()  [unwired: 2 out]
              }
              frame -1 {
                n144 = Build Array (concatenate)(w273, w272) -> (w271:path[])
                n145 = local write "Results files choosen"(w271) -> ()
              }
            }
            n146 = local write "Results file"(w263) -> ()
            n147 = Increment(x=w260) -> (x+1=w259:i32)
          }
          frame True {
          }
        }
        n148 = local read "stop"() -> (w250:bool)
        n149 = Decrement(x=w247) -> (x-1=w246:i32)
        n150 = Build Array(w246) -> (w248:i32[])
        n151 = Not(x=w250) -> (.not. x?=w249:bool)
        n152 = local write "File Index"(w247) -> ()
        n153 = property on="Result files to read" class="Arr (strict)"("Index Values"=w248) -> ()  [unwired: 2 in, 2 out]
      }
      frame "Load Data" {
        n154 = stacked-sequence {
          seq-local: [w288 _] -> [_ w348]
          seq-local: [w287 _] -> [_ w353]
          seq-local: [w286 _] -> [_ w352]
          seq-local: [w284 _] -> [_ w351]
          tunnel: [TRUE _] -> w283
          tunnel: w282 -> [w302 w354]
          tunnel: w281 -> [w301 _]
          tunnel: [w300 _] -> w280
          tunnel: [w299 _] -> w279
          tunnel: [w298 _] -> w278
          tunnel: w277 -> [w297 _]
          tunnel: ["Which file to read next" _] -> w276
          frame #0 {
            w291 = TRUE  # Add Extra Channels?
            n155 = local read "Template"() -> (w295:path)
            n156 = call "Read_Data_file.vi"("Results file"="Results file", "Add Extra Channels?"=w291, "Template File"=w295, "Desired File Types"="File Types to Read") -> ("Row numbers"=w286:i32[], "Template File Out"=w292:path, "Filetype"=w287:string, "Results file Out"=w288:path, "Ch names Out"=w293:string[], "Channel Values Out"=w289:string[][])  [unwired: 1 in, 9 out]
            n157 = local write "Template"(w292) -> ()
            n158 = Array Size(array=w293) -> (size(s)=w294:i32)
            n159 = Greater Than 0?(x=w294) -> (x > 0?=w284:bool)
            n160 = case shown="True" w284 {
              tunnel: w302 -> [w304 w318]
              tunnel: w301 -> [w306 w312]
              tunnel: w289 -> [_ w310]
              tunnel: [w304 w308] -> w300
              tunnel: [w306 w316] -> w299
              tunnel: [w305 w307] -> w298
              tunnel: w297 -> [w305 _]
              tunnel: w293 -> [_ w311]
              frame False {
              }
              frame True {
                n161 = for {
                  tunnel: w310 -> [w320] mode=indexing
                  tunnel: [w319] -> w309 mode=indexing
                  n162 = for {
                    tunnel: w320 -> [w322] mode=indexing
                    tunnel: [w321] -> w319 mode=indexing
                    n163 = call "Fast_string_Replace.vi"("Replace match with:"="[", "Input String"=w322, "regular expression"="(") -> ("Output String"=w323:string)  [unwired: 2 out]
                    n164 = call "Fast_string_Replace.vi"("Replace match with:"="]", "Input String"=w323, "regular expression"=")") -> ("Output String"=w321:string)  [unwired: 2 out]
                  }
                }
                n165 = call "Merge_channel_names.vi"("Preferred Channel array"=w312, "Channel array"=w311) -> ("Merged Channels"=w316:string[], "Preferred Channels Changed?"=w314:bool, "Channel Array Changed?"=w315:bool)
                n166 = for {
                  tunnel: w316 -> [w345] mode=indexing
                  tunnel: [w342] -> w307 mode=indexing
                  n167 = call "Fast_string_Replace.vi"("Replace match with:"=" ", "Input String"=w345, "regular expression"=":") -> ("Output String"=w341:string)  [unwired: 2 out]
                  n168 = call "Fast_string_Replace.vi"("Replace match with:"=" ", "Input String"=w341, "regular expression"="  ") -> ("Output String"=w340:string)  [unwired: 2 out]
                  n169 = call <vilib>:"Trim Whitespace.vi"("string"=w340) -> ("trimmed string"=w342:string)  [unwired: 1 in]
                }
                n170 = case shown="True" w314 {
                  tunnel: w318 -> [w333 w335]
                  tunnel: w312 -> [_ w337]
                  tunnel: [w333 w334] -> w313
                  tunnel: w316 -> [_ w336]
                  frame False {
                  }
                  frame True {
                    n171 = call "Merge_2D_values.vi"("Values In"=w335, "Present Channels"=w337, "Desired Channels"=w336) -> ("Values Out"=w334:string[][])
                  }
                }
                n172 = case shown="True" w315 {
                  tunnel: [w328 w332] -> w317
                  tunnel: w311 -> [_ w331]
                  tunnel: w309 -> [w328 w330]
                  tunnel: w316 -> [_ w329]
                  frame False {
                  }
                  frame True {
                    n173 = call "Merge_2D_values.vi"("Values In"=w330, "Present Channels"=w331, "Desired Channels"=w329) -> ("Values Out"=w332:string[][])
                  }
                }
                n174 = global write "Results_plotter_Global.vi" "Channel names"(w307) -> ()
                n175 = Build Array (concatenate)(w313, w317) -> (w308:string[][])
                n176 = global write "Results_plotter_Global.vi" "All Data"(w308) -> ()
              }
            }
          }
          frame #1 {
            n177 = local read "File Index"() -> (w350:i32)
            n178 = Decrement(x=w350) -> (x-1=w349:i32)
            n179 = local read "Result files to read"() -> (w347:path[])
            n180 = case shown="True" w351 {
              tunnel: w354 -> [_ w367]
              tunnel: w353 -> [_ w365]
              tunnel: w352 -> [_ w363]
              tunnel: w349 -> [w355 w361]
              tunnel: w348 -> [_ w360]
              tunnel: w347 -> [w357 w362]
              tunnel: [w356 w359] -> w346
              frame False {
                n181 = Delete From Array(array=w357, length=1, index=w355) -> (array with subset deleted=w356:path[])  [unwired: 1 out]
                n182 = local write "File Index"(w355) -> ()
              }
              frame True {
                n183 = Array Size(array=w367) -> (size(s)=w369:i32[])
                n184 = Index Array(array=w369, index=0 ("Index")) -> (element=w366:i32)
                n185 = for {
                  tunnel: w361 -> [w386]
                  tunnel: [w385] -> w371 mode=indexing
                  tunnel: w366 -> [w382]
                  tunnel: w363 -> [w381] mode=indexing
                  i -> [w383]
                  n186 = Add(x=w383, y=w382) -> (x+y=w384:i32)
                  n187 = Build Array(w386, w381, w384) -> (w385:i32[])
                }
                n188 = case shown="1, Default" w361 {
                  tunnel: w371 -> [w374 w379]
                  tunnel: [w374 w378] -> w370
                  tunnel: w365 -> [w373 w377]
                  tunnel: [w372 w375] -> w364
                  frame 0 {
                    n189 = Build Array(w373) -> (w372:string[])
                  }
                  frame 1, Default {
                    n190 = global read "Results_plotter_Global.vi" "Row Reference"() -> (w380:i32[][])
                    n191 = local read "Filetype"() -> (w376:string[])
                    n192 = Build Array (concatenate)(w376, w377) -> (w375:string[])
                    n193 = Build Array (concatenate)(w380, w379) -> (w378:i32[][])
                  }
                }
                "Filetype" <- w364
                n194 = Replace Array Subset(array=w362, new element=w360, index=w361) -> (w359:path[])
                n195 = global write "Results_plotter_Global.vi" "Row Reference"(w370) -> ()
              }
            }
            n196 = local write "Result files to read"(w346) -> ()
          }
        }
      }
      frame "Load Selectors" {
        n197 = while {
          shift-right: [w407] -> w392
          shift-left: _ -> [w409]
          tunnel: [w409] -> w391
          tunnel: w387 -> [w407]
          stop <- FALSE continue-if-true
        }
        n198 = Array Size(array=w399) -> (size(s)=w398:i32[])
        n199 = local read "Tolerances"() -> (w395:dbl[])
        n200 = Index Array(array=w398, index=0 ("Index")) -> (element=→"nRows":i32)
        n201 = Equal?(x=w392, y=w391) -> (x = y?=w390:bool)
        n202 = Build Array (concatenate)("Don't Filter" ("Input Element"), w387) -> (w404:string[])
        n203 = Array Size(array=w387) -> (size(s)=w401:i32)
        n204 = Array Size(array=w395) -> (size(s)=w400:i32)
        n205 = property on="Multi Ordinate" class="LstBox (strict)"("Item Names"=w387) -> ()  [unwired: 2 in, 2 out]
        n206 = property on="Z Ch Name" class="Ring (strict)"("Strings []"=w387) -> ()  [unwired: 2 in, 2 out]
        n207 = property on="Y Ch Name" class="Ring (strict)"("Strings []"=w387) -> ()  [unwired: 2 in, 2 out]
        n208 = property on="X Ch Name" class="Ring (strict)"("Strings []"=w387) -> ()  [unwired: 2 in, 2 out]
        n209 = property on="X Axis" class="Ring (strict)"("Strings []"=w387) -> ()  [unwired: 2 in, 2 out]
        n210 = property on="Ordinate" class="Ring (strict)"("Strings []"=w387) -> ()  [unwired: 2 in, 2 out]
        n211 = property on="Filter on column 1:" class="Ring (strict)"("Strings []"=w404) -> ()  [unwired: 2 in, 2 out]
        n212 = Not Equal?(x=w401, y=w400) -> (x != y?=w402:bool)
        n213 = case shown="True" w402 {
          tunnel: w401 -> [_ w416]
          tunnel: w400 -> [_ w415]
          tunnel: w395 -> [_ w412]
          frame False {
          }
          frame True {
            n214 = Subtract(x=w416, y=w415) -> (x-y=w414:i32)
            n215 = Initialize Array(1.0 ("Element Data"), w414) -> (w411:dbl[])
            n216 = Build Array (concatenate)(w412, w411) -> (w410:dbl[])
            n217 = local write "Tolerances"(w410) -> ()
          }
        }
        n218 = global write "Results_plotter_Global.vi" "First Loop"(TRUE) -> ()
        n219 = Select(t="What is present?", s=w390, f="Set Axis Channels") -> (s? t:f=w394:string)
      }
      frame "Set Axis Channels" {
        n220 = Array Size(array=w423) -> (size(s)=w422:i32)
        n221 = Build Array("X" ("regular expression"), "Y" ("regular expression"), "Z" ("regular expression")) -> (w417:string[])
        n222 = Decrement(x=w422) -> (x-1=w421:i32)
        n223 = for {
          tunnel: w423 -> [w435]
          tunnel: w421 -> [w434]
          tunnel: w417 -> [w433] mode=indexing
          i -> [w429]
          n224 = while {
            tunnel: w435 -> [w449] mode=indexing
            tunnel: w434 -> [w448]
            tunnel: w433 -> [w446]
            tunnel: [w439] -> w432
            tunnel: [w444] -> w431
            i -> [w444]
            stop <- w447 continue-if-true
            n225 = call "Match_Pat_Case_In.vi"("String to match"=w446, "String"=w449) -> ("offset past match"=w443:i32)  [unwired: 1 in, 3 out]
            n226 = In Range and Coerce(upper limit=4, x=w443, lower limit=0) -> (In Range?=w440:bool)  [unwired: 1 out]
            n227 = Less?(x=w444, y=w448) -> (x < y?=w445:bool)
            n228 = Not(x=w440) -> (.not. x?=w439:bool)
            n229 = And(x=w439, y=w445) -> (x .and. y?=w447:bool)
          }
          n230 = Select(t=0, s=w432, f=w431) -> (s? t:f=w428:i32)
          n231 = case shown="1" w429 {
            tunnel: w428 -> [w436 w437 w438]
            frame 0, Default {
              n232 = local write "X Ch Name"(w436) -> ()
            }
            frame 1 {
              n233 = local write "Y Ch Name"(w437) -> ()
            }
            frame 2 {
              n234 = local write "Z Ch Name"(w438) -> ()
            }
          }
        }
      }
      frame "What is present?" {
        n235 = case shown="True" "Show Results Space Analysis" {
          tunnel: w453 -> [_ w457]
          tunnel: w452 -> [_ w456]
          frame False {
          }
          frame True {
            n236 = stacked-sequence {
              tunnel: w457 -> [w461]
              tunnel: w456 -> [w460]
              frame #0 {
                w458 = FALSE  # Summarise All
                n237 = call "Summarise.vi"("Channel Names"=w461, "Data"=w460, "Summarise All"=w458) -> ("Summary"=w459:string[][])  [unwired: 2 in]
                n238 = call "Results_Space_Analysis.vi"("Table"=w459) -> ()
              }
            }
          }
        }
      }
      frame "Ordinate Selector Type" {
        n239 = while {
          tunnel: [w480] -> w471
          shift-left: _ -> [w480]
          shift-right: ["Slice mode"] -> w472
          stop <- FALSE continue-if-true
          "Previous slice mode" <- w480
        }
        n240 = Not(x="Multi Ordinate?") -> (.not. x?=w466:bool)
        n241 = property on="Multi Ordinate" class="LstBox (strict)"("Visible"="Multi Ordinate?") -> ()  [unwired: 2 in, 2 out]
        n242 = property on="Ordinate Name" class="Str"("Visible"="Multi Ordinate?") -> ()  [unwired: 2 in, 2 out]
        n243 = property on="Ordinate" class="Ring (strict)"("Visible"=w466) -> ()  [unwired: 2 in, 2 out]
        n244 = property on="First Add label" class="Str"("Visible"=w466) -> ()  [unwired: 2 in, 2 out]
        n245 = property on="2nd Add label" class="Str"("Visible"=w466) -> ()  [unwired: 2 in, 2 out]
        n246 = property on="Additional Y Values" class="Arr (strict)"("Visible"=w466) -> ()  [unwired: 2 in, 2 out]
        n247 = property on="Additional X Values" class="Arr (strict)"("Visible"=w466) -> ()  [unwired: 2 in, 2 out]
        n248 = Not Equal?(x=w472, y=w471) -> (x != y?=w463:bool)
        n249 = local read "Intensity Plot?"() -> (w470:bool)
        n250 = Or(x=w463, y="Update") -> (x .or. y?=w464:bool)
        n251 = global read "Results_plotter_Global.vi" "First Loop"() -> (w467:bool)
        n252 = case shown="False" "Multi Ordinate?" {
          frame False {
            n253 = Build Array("Ordinate") -> (w482:u16[])
            n254 = local write "Multi Ordinate"(w482) -> ()
          }
          frame True {
          }
        }
        n255 = Compound Arithmetic op=AND(invert w467, w464, w470) -> (w469:bool)
        "Slice mode Change?" <- w469
        n256 = Select(t="Change Slice mode", s=w469, f="Which rows are Non-Blank?") -> (s? t:f=w473:string)
      }
      frame "Change Slice mode" {
        n257 = local read "Previous slice mode"() -> (w486:T3)
        n258 = local read "Slice mode"() -> (w500:T3)
        n259 = case shown="\"YX Slice (Plan)\"" w500 {
          tunnel: [w512 w517 w524 w529 w536 w542] -> w499
          tunnel: "Y Ch Name" -> [w510 w517 w524 w530 w535 w540]
          tunnel: "X Ch Name" -> [w512 w516 w523 w528 w536 w541]
          tunnel: [w511 w518 w523 w528 w535 w540] -> w490
          tunnel: "Z Ch Name" -> [w511 w518 w522 w529 w534 w542]
          tunnel: [w510 w516 w522 w530 w534 w541] -> w488
          tunnel: w486 -> [w509 w514 w520 w526 w533 w538]
          tunnel: [w507 w513 w519 w525 w532 w537] -> w485
          frame "XY Slice (Plan)" {
            n260 = Equal?(x=Plot_Slice."YX Slice (Plan)" ("Previous slice mode"), y=w509) -> (x = y?=w507:bool)
          }
          frame "YX Slice (Plan)" {
            n261 = Equal?(x=Plot_Slice."XY Slice (Plan)" ("Previous slice mode"), y=w514) -> (x = y?=w513:bool)
          }
          frame "YZ Slice (Cross)" {
            n262 = Equal?(x=Plot_Slice."ZY Slice (Cross)" ("Previous slice mode"), y=w520) -> (x = y?=w519:bool)
          }
          frame "ZY Slice (Cross)" {
            n263 = Equal?(x=Plot_Slice."YZ Slice (Cross)" ("Previous slice mode"), y=w526) -> (x = y?=w525:bool)
          }
          frame "XZ Slice (Side)" {
            n264 = Equal?(x=Plot_Slice."ZX Slice (Side)" ("Previous slice mode"), y=w533) -> (x = y?=w532:bool)
          }
          frame "ZX Slice (Side)" {
            n265 = Equal?(x=Plot_Slice."XZ Slice (Side)" ("Previous slice mode"), y=w538) -> (x = y?=w537:bool)
          }
        }
        n266 = case shown="True" w485 {
          frame False {
          }
          frame True {
            n267 = local read "Transpose"() -> (w506:bool)
            n268 = Not(x=w506) -> (.not. x?=w505:bool)
            n269 = local write "Transpose"(w505) -> ()
          }
        }
        n270 = local write "Update"(FALSE ("Update")) -> ()
        n271 = Increment(x=w490) -> (x+1=w493:u16)
        n272 = Increment(x=w488) -> (x+1=w492:u16)
        n273 = local read "Filter Array"() -> (w497:u16[])
        n274 = Array Subset(array=w497, index=2 ("Array Index")) -> (w495:u16[])  [unwired: 1 in]
        n275 = Build Array (concatenate)(w493, w492, w495) -> (w494:u16[])
        n276 = local write "Filter Array"(w494) -> ()
        n277 = local write "Absisca"(w499) -> ()
      }
      frame "Which rows are Non-Blank?" {
        n278 = while {
          tunnel: [w559] -> w553
          tunnel: [w560] -> w554
          shift-left: _ -> [w561]
          shift-right: [w562] -> w546
          shift-left: _ -> [w564]
          shift-right: [w563] -> _
          stop <- FALSE continue-if-true
          n279 = local read "Multi Ordinate"() -> (w562:i32[])
          n280 = local read "Absisca"() -> (w563:u16)
          n281 = Equal?(x=w563, y=w564) -> (x = y?=w560:bool)
          n282 = Equal?(x=w562, y=w561) -> (x = y?=w559:bool)
        }
        n283 = global read "Results_plotter_Global.vi" "First Loop"() -> (w548:bool)
        n284 = Compound Arithmetic op=AND(invert w548, w554, w553) -> (w552:bool)
        n285 = Array Size(array=w546) -> (size(s)=w545:i32)
        n286 = Greater?(x=w545, y=1) -> (0:w543:bool)
        n287 = global write "Results_plotter_Global.vi" "Multi Ordinate?"(w543) -> ()
        n288 = Select(t="Create Selectors", s=w552, f="Evaluate Blank Rows") -> (s? t:f=w549:string)
      }
      frame "Evaluate Blank Rows" {
        n289 = local read "Multi Ordinate"() -> (w566:i32[])
        n290 = local read "Absisca"() -> (w567:u16)
        n291 = for {
          tunnel: w568 -> [w574] mode=indexing
          tunnel: w567 -> [w577]
          tunnel: w566 -> [w576]
          tunnel: [w573] -> w565 mode=indexing
          n292 = Index Array(array=w574, index=w577) -> (element=w578:string)
          n293 = call "Convert_to_number.vi"("string"=w578) -> ("Number"=w579:dbl)  [unwired: 1 out]
          n294 = Not A Number/Path/Refnum?(number/path/refnum=w579) -> (NaN/Path/Refnum?=w575:bool)
          n295 = case shown="False" w575 {
            tunnel: w576 -> [w583 _]
            tunnel: w574 -> [w582 _]
            tunnel: [w580 FALSE] -> w573
            frame False {
              n296 = for {
                tunnel: w583 -> [w589] mode=indexing
                tunnel: w582 -> [w587]
                tunnel: [w584] -> w581 mode=indexing
                n297 = Index Array(array=w587, index=w589) -> (element=w588:string)
                n298 = call "Convert_to_number.vi"("string"=w588) -> ("Number"=w586:dbl)  [unwired: 1 out]
                n299 = Not A Number/Path/Refnum?(number/path/refnum=w586) -> (NaN/Path/Refnum?=w585:bool)
                n300 = Not(x=w585) -> (.not. x?=w584:bool)
              }
              n301 = Or Array Elements(Boolean array=w581) -> (logical OR=w580:bool)
            }
            frame True {
            }
          }
        }
        "Non-Blank Rows" <- w565
      }
      frame "Create Selectors" {
        n302 = local read "Non-Blank Rows"() -> (w594:bool[])
        n303 = local read "Tolerances"() -> (w592:dbl[])
        n304 = global read "Results_plotter_Global.vi" "Precision"() -> (w591:string[])
        n305 = Array Size(array=w602) -> (size(s)=w601:i32[])
        n306 = Index Array(array=w601, index=0 ("Index")) -> (element=w604:i32)
        n307 = for {
          tunnel: w602 -> [w620]
          tunnel: "Filter Array" -> [w612] mode=indexing
          shift-right: [w619] -> w593
          shift-left: _ -> [w617]
          tunnel: w604 -> [w618]
          tunnel: [w615] -> w599 mode=indexing
          tunnel: w594 -> [w614]
          tunnel: w592 -> [w613]
          tunnel: w591 -> [w610]
          i -> [w616]
          n308 = Decrement(x=w612) -> (x-1=w609:u16)
          n309 = Index Array(array=w610, index=w609) -> (element=w608:string)
          n310 = Index Array(array=w613, index=w609) -> (element=w611:dbl)
          n311 = case shown="1" w616 {
            tunnel: w620 -> [w633 w669 w710 w751 w792 w835 w876]
            tunnel: w612 -> [w632 w668 w709 w750 w791 w834 w875]
            tunnel: w611 -> [w631 w667 w708 w749 w790 w833 w874]
            tunnel: [w630 w666 w707 w748 w789 w832 w873] -> w619
            tunnel: w618 -> [w628 w665 w706 w747 w788 w831 w872]
            tunnel: w617 -> [_ w664 w705 w746 w787 w830 w871]
            tunnel: w616 -> [w627 w663 w702 w743 w784 w829 w868]
            tunnel: [w623 w658 w701 w742 w783 w824 w867] -> w615
            tunnel: w614 -> [w622 w657 w700 w741 w782 w823 w866]
            tunnel: w608 -> [w621 w656 w699 w740 w781 w822 w865]
            frame 0, Default {
              n312 = case shown="1, Default" w632 {
                tunnel: w633 -> [w639 w649]
                tunnel: w632 -> [w640 w648]
                tunnel: w631 -> [_ w655]
                tunnel: [w635 w652] -> w630
                tunnel: "Filter Bins 1" -> [_ w653]
                tunnel: [string[] [] ("Write Attribute") w654] -> w629
                tunnel: w628 -> [w637 _]
                tunnel: w627 -> [w643 w651]
                tunnel: [i32[] [0] ("Filter Bins Out") w650] -> w625
                tunnel: [TRUE ("Unchanged?") w647] -> w623
                tunnel: w622 -> [_ w646]
                tunnel: w621 -> [_ w645]
                frame 0 {
                  n313 = call "Create_filter_points.vi"("Channel to Filter On"=w640, "Index"=w643, "Ch Values In"=w639) -> ()  [unwired: 4 in, 4 out]
                  n314 = Initialize Array(TRUE, w637) -> (w636:bool[])
                  n315 = Build Array(w636) -> (w635:bool[][])
                }
                frame 1, Default {
                  n316 = call "Create_filter_points.vi"("Non-Blank Rows"=w646, "Precision"=w645, "Channel to Filter On"=w648, "Tolerance"=w655, "Index"=w651, "Filter Bins 1"=w653, "Ch Values In"=w649) -> ("Unchanged?"=w647:bool, "Accept array"=w652:bool[][], "Filter Bins Out"=w650:i32[], "Bin Names"=w654:string[])
                }
              }
              n317 = Equal?(x="Filter Bins 1", y=w625) -> (x = y?=w624:bool)
              n318 = case shown="False" w624 {
                tunnel: w625 -> [w634 _]
                frame False {
                  n319 = local write "Filter Bins 1"(w634) -> ()
                }
                frame True {
                }
              }
              n320 = property on="Filter bins 1" class="LstBox (strict)"("Item Names"=w629) -> ()  [unwired: 2 in, 2 out]
            }
            frame 1 {
              n321 = case shown="1, Default" w668 {
                tunnel: w669 -> [_ w681]
                tunnel: w668 -> [w672 w680]
                tunnel: w667 -> [_ w688]
                tunnel: [w676 w684] -> w666
                tunnel: "Filter Bins 2" -> [_ w686]
                tunnel: [string[] [] ("Write Attribute") w690] -> w662
                tunnel: w665 -> [_ _]
                tunnel: w664 -> [w676 w689]
                tunnel: w663 -> [w675 w687]
                tunnel: [i32[] [0] ("Filter Bins Out") w682] -> w661
                tunnel: [TRUE ("Unchanged?") w679] -> w658
                tunnel: w657 -> [_ w678]
                tunnel: w656 -> [_ w677]
                frame 0 {
                  n322 = call "Create_filter_points.vi"("Channel to Filter On"=w672, "Index"=w675) -> ()  [unwired: 5 in, 4 out]
                }
                frame 1, Default {
                  n323 = call "Create_filter_points.vi"("Non-Blank Rows"=w678, "Precision"=w677, "Channel to Filter On"=w680, "Tolerance"=w688, "Index"=w687, "Filter Bins 1"=w686, "Ch Values In"=w681) -> ("Unchanged?"=w679:bool, "Accept array"=w685:bool[][], "Filter Bins Out"=w682:i32[], "Bin Names"=w690:string[])
                  n324 = for {
                    tunnel: w689 -> [w695]
                    tunnel: w685 -> [w694] mode=indexing
                    shift-right: [w691] -> w684
                    shift-left: bool[][] [] -> [w693]
                    n325 = for {
                      tunnel: w694 -> [w698]
                      tunnel: w695 -> [w697] mode=indexing
                      tunnel: [w696] -> _ mode=indexing
                      tunnel: [w696] -> w692 mode=indexing
                      n326 = And(x=w698, y=w697) -> (x .and. y?=w696:bool[])
                    }
                    n327 = Build Array (concatenate)(w693, w692) -> (w691:bool[][])
                  }
                }
              }
              n328 = Equal?(x="Filter Bins 2", y=w661) -> (x = y?=w659:bool)
              n329 = case shown="False" w659 {
                tunnel: w661 -> [w670 _]
                frame False {
                  n330 = local write "Filter Bins 2"(w670) -> ()
                }
                frame True {
                }
              }
              n331 = property on="Filter Bins 2" class="LstBox (strict)"("Item Names"=w662) -> ()  [unwired: 2 in, 2 out]
            }
            frame 2 {
              n332 = case shown="0" w709 {
                tunnel: w710 -> [_ w720]
                tunnel: w709 -> [w713 w721]
                tunnel: w708 -> [_ w732]
                tunnel: [w716 w733] -> w707
                tunnel: "Filter 3" -> [_ w724]
                tunnel: [string[] [] ("Write Attribute") w735] -> w703
                tunnel: w706 -> [_ _]
                tunnel: w705 -> [w716 w734]
                tunnel: w702 -> [w715 w727]
                tunnel: [TRUE ("Unchanged?") w719] -> w701
                tunnel: w700 -> [_ w718]
                tunnel: w699 -> [_ w717]
                frame 0 {
                  n333 = call "Create_filter_points.vi"("Channel to Filter On"=w713, "Index"=w715) -> ()  [unwired: 5 in, 4 out]
                  n334 = local write "Filter 3"(0) -> ()
                }
                frame 1, Default {
                  n335 = Build Array(w724) -> (w731:u16[])
                  n336 = call "Create_filter_points.vi"("Non-Blank Rows"=w718, "Precision"=w717, "Channel to Filter On"=w721, "Tolerance"=w732, "Index"=w727, "Filter Bins 1"=w731, "Ch Values In"=w720) -> ("Unchanged?"=w719:bool, "Accept array"=w729:bool[][], "Filter Bins Out"=w725:i32[], "Bin Names"=w735:string[])
                  n337 = Index Array(array=w725, index=0 ("Index")) -> (element=w722:i32)
                  n338 = Index Array(array=w729, index (row)=0 ("Index")) -> (element=w728:bool[])  [unwired: 1 in]
                  n339 = Equal?(x=w724, y=w722) -> (x = y?=w723:bool)
                  n340 = case shown="True" w723 {
                    tunnel: w722 -> [w736 _]
                    frame False {
                      n341 = local write "Filter 3"(w736) -> ()
                    }
                    frame True {
                    }
                  }
                  n342 = for {
                    tunnel: w728 -> [w739]
                    tunnel: w734 -> [w738] mode=indexing
                    tunnel: [w737] -> w733 mode=indexing
                    n343 = And(x=w739, y=w738) -> (x .and. y?=w737:bool[])
                  }
                }
              }
              n344 = property on="Filter 3" class="Ring (strict)"("Strings []"=w703) -> ()  [unwired: 2 in, 2 out]
            }
            frame 3 {
              n345 = case shown="1, Default" w750 {
                tunnel: w751 -> [_ w762]
                tunnel: w750 -> [w754 w761]
                tunnel: w749 -> [_ w773]
                tunnel: [w757 w774] -> w748
                tunnel: "Filter 4" -> [_ w765]
                tunnel: [string[] [] ("Write Attribute") w776] -> w744
                tunnel: w747 -> [_ _]
                tunnel: w746 -> [w757 w775]
                tunnel: w743 -> [w756 w768]
                tunnel: [TRUE ("Unchanged?") w760] -> w742
                tunnel: w741 -> [_ w759]
                tunnel: w740 -> [_ w758]
                frame 0 {
                  n346 = call "Create_filter_points.vi"("Channel to Filter On"=w754, "Index"=w756) -> ()  [unwired: 5 in, 4 out]
                  n347 = local write "Filter 4"(0) -> ()
                }
                frame 1, Default {
                  n348 = Build Array(w765) -> (w772:u16[])
                  n349 = call "Create_filter_points.vi"("Non-Blank Rows"=w759, "Precision"=w758, "Channel to Filter On"=w761, "Tolerance"=w773, "Index"=w768, "Filter Bins 1"=w772, "Ch Values In"=w762) -> ("Unchanged?"=w760:bool, "Accept array"=w770:bool[][], "Filter Bins Out"=w766:i32[], "Bin Names"=w776:string[])
                  n350 = Index Array(array=w766, index=0 ("Index")) -> (element=w764:i32)
                  n351 = Equal?(x=w765, y=w764) -> (x = y?=w763:bool)
                  n352 = Index Array(array=w770, index (row)=0 ("Index")) -> (element=w769:bool[])  [unwired: 1 in]
                  n353 = case shown="False" w763 {
                    tunnel: w764 -> [w777 _]
                    frame False {
                      n354 = local write "Filter 4"(w777) -> ()
                    }
                    frame True {
                    }
                  }
                  n355 = for {
                    tunnel: w769 -> [w780]
                    tunnel: w775 -> [w779] mode=indexing
                    tunnel: [w778] -> w774 mode=indexing
                    n356 = And(x=w780, y=w779) -> (x .and. y?=w778:bool[])
                  }
                }
              }
              n357 = property on="Filter 4" class="Ring (strict)"("Strings []"=w744) -> ()  [unwired: 2 in, 2 out]
            }
            frame 4 {
              n358 = case shown="1, Default" w791 {
                tunnel: w792 -> [_ w803]
                tunnel: w791 -> [w795 w802]
                tunnel: w790 -> [_ w814]
                tunnel: [w798 w815] -> w789
                tunnel: "Filter 5" -> [_ w805]
                tunnel: [string[] [] ("Write Attribute") w817] -> w785
                tunnel: w788 -> [_ _]
                tunnel: w787 -> [w798 w816]
                tunnel: w784 -> [w797 w809]
                tunnel: [TRUE ("Unchanged?") w801] -> w783
                tunnel: w782 -> [_ w800]
                tunnel: w781 -> [_ w799]
                frame 0 {
                  n359 = call "Create_filter_points.vi"("Channel to Filter On"=w795, "Index"=w797) -> ()  [unwired: 5 in, 4 out]
                  n360 = local write "Filter 5"(0) -> ()
                }
                frame 1, Default {
                  n361 = Build Array(w805) -> (w813:u16[])
                  n362 = call "Create_filter_points.vi"("Non-Blank Rows"=w800, "Precision"=w799, "Channel to Filter On"=w802, "Tolerance"=w814, "Index"=w809, "Filter Bins 1"=w813, "Ch Values In"=w803) -> ("Unchanged?"=w801:bool, "Accept array"=w811:bool[][], "Filter Bins Out"=w807:i32[], "Bin Names"=w817:string[])
                  n363 = Index Array(array=w807, index=0 ("Index")) -> (element=w806:i32)
                  n364 = Equal?(x=w805, y=w806) -> (x = y?=w804:bool)
                  n365 = Index Array(array=w811, index (row)=0 ("Index")) -> (element=w810:bool[])  [unwired: 1 in]
                  n366 = case shown="False" w804 {
                    tunnel: w806 -> [w818 _]
                    frame False {
                      n367 = local write "Filter 5"(w818) -> ()
                    }
                    frame True {
                    }
                  }
                  n368 = for {
                    tunnel: w810 -> [w821]
                    tunnel: w816 -> [w820] mode=indexing
                    tunnel: [w819] -> w815 mode=indexing
                    n369 = And(x=w821, y=w820) -> (x .and. y?=w819:bool[])
                  }
                }
              }
              n370 = property on="Filter 5" class="Ring (strict)"("Strings []"=w785) -> ()  [unwired: 2 in, 2 out]
            }
            frame 5 {
              n371 = case shown="1, Default" w834 {
                tunnel: w835 -> [_ w852]
                tunnel: w834 -> [w838 w851]
                tunnel: w833 -> [_ w856]
                tunnel: [w842 w843] -> w832
                tunnel: "Single Series" -> [_ w854]
                tunnel: [string[] [] ("Write Attribute") w858] -> w828
                tunnel: w831 -> [_ _]
                tunnel: w830 -> [w842 w857]
                tunnel: w829 -> [w841 w855]
                tunnel: [i32[] [0] ("Filter Bins Out") w853] -> w827
                tunnel: [TRUE ("Unchanged?") w850] -> w824
                tunnel: w823 -> [_ w849]
                tunnel: w822 -> [_ w848]
                frame 0 {
                  n372 = call "Create_filter_points.vi"("Channel to Filter On"=w838, "Index"=w841) -> ()  [unwired: 5 in, 4 out]
                }
                frame 1, Default {
                  n373 = call "Create_filter_points.vi"("Non-Blank Rows"=w849, "Precision"=w848, "Channel to Filter On"=w851, "Tolerance"=w856, "Index"=w855, "Filter Bins 1"=w854, "Ch Values In"=w852) -> ("Unchanged?"=w850:bool, "Accept array"=w845:bool[][], "Filter Bins Out"=w853:i32[], "Bin Names"=w858:string[])
                  n374 = Index Array(array=w845, index (row)=0 ("Index")) -> (element=w846:bool[])  [unwired: 1 in]
                  n375 = for {
                    shift-right: [w859] -> w844
                    shift-left: w846 -> [w861]
                    tunnel: w845 -> [w860] mode=indexing
                    n376 = Or(x=w860, y=w861) -> (x .or. y?=w859:bool[])
                  }
                  n377 = for {
                    tunnel: w844 -> [w864]
                    tunnel: w857 -> [w863] mode=indexing
                    tunnel: [w862] -> w843 mode=indexing
                    n378 = And(x=w864, y=w863) -> (x .and. y?=w862:bool[])
                  }
                }
              }
              n379 = Equal?(x="Single Series", y=w827) -> (x = y?=w825:bool)
              n380 = case shown="False" w825 {
                tunnel: w827 -> [w836 _]
                frame False {
                  n381 = local write "Single Series"(w836) -> ()
                }
                frame True {
                }
              }
              n382 = property on="Single Series" class="LstBox (strict)"("Item Names"=w828) -> ()  [unwired: 2 in, 2 out]
            }
            frame 6 {
              n383 = case shown="1, Default" w875 {
                tunnel: w876 -> [_ w887]
                tunnel: w875 -> [w879 w886]
                tunnel: w874 -> [_ w894]
                tunnel: [w882 w899] -> w873
                tunnel: "Filter 6" -> [_ w889]
                tunnel: [string[] [] ("Write Attribute") w901] -> w869
                tunnel: w872 -> [_ _]
                tunnel: w871 -> [w882 w900]
                tunnel: w868 -> [w881 w893]
                tunnel: [TRUE ("Unchanged?") w885] -> w867
                tunnel: w866 -> [_ w884]
                tunnel: w865 -> [_ w883]
                frame 0 {
                  n384 = call "Create_filter_points.vi"("Channel to Filter On"=w879, "Index"=w881) -> ()  [unwired: 5 in, 4 out]
                  n385 = local write "Filter 6"(0) -> ()
                }
                frame 1, Default {
                  n386 = Build Array(w889) -> (w895:u16[])
                  n387 = call "Create_filter_points.vi"("Non-Blank Rows"=w884, "Precision"=w883, "Channel to Filter On"=w886, "Tolerance"=w894, "Index"=w893, "Filter Bins 1"=w895, "Ch Values In"=w887) -> ("Unchanged?"=w885:bool, "Accept array"=w897:bool[][], "Filter Bins Out"=w891:i32[], "Bin Names"=w901:string[])
                  n388 = Index Array(array=w891, index=0 ("Index")) -> (element=w890:i32)
                  n389 = Equal?(x=w889, y=w890) -> (x = y?=w888:bool)
                  n390 = Index Array(array=w897, index (row)=0 ("Index")) -> (element=w896:bool[])  [unwired: 1 in]
                  n391 = case shown="False" w888 {
                    tunnel: w890 -> [w902 _]
                    frame False {
                      n392 = local write "Filter 6"(w902) -> ()
                    }
                    frame True {
                    }
                  }
                  n393 = for {
                    tunnel: w896 -> [w905]
                    tunnel: w900 -> [w904] mode=indexing
                    tunnel: [w903] -> w899 mode=indexing
                    n394 = And(x=w905, y=w904) -> (x .and. y?=w903:bool[])
                  }
                }
              }
              n395 = property on="Filter 6" class="Ring (strict)"("Strings []"=w869) -> ()  [unwired: 2 in, 2 out]
            }
          }
        }
        "Accept Array" <- w593
        n396 = And Array Elements(Boolean array=w599) -> (logical AND=w598:bool)
        n397 = Select(t="Select all for Filter 2", s=w598, f="Create Selectors") -> (s? t:f=w596:string)
      }
      frame "Select all for Filter 2" {
        n398 = local read "Slice mode Change?"() -> (w907:bool)
        n399 = case shown="True" w907 {
          frame False {
          }
          frame True {
            n400 = property on="Filter Bins 2" class="LstBox (strict)"() -> ("Item Names"=w921:string[])  [unwired: 2 in, 2 out]
            n401 = Array Size(array=w921) -> (size(s)=w920:i32)
            n402 = Build Array("Blanks", "Numeric", "Non Numeric", "Non Blanks", "Show All" ("Input Element")) -> (w914:string[])
            n403 = local read "Filter Bins 1"() -> (w923:i32[])
            n404 = while {
              tunnel: w921 -> [w936] mode=indexing
              tunnel: w920 -> [w939]
              shift-right: [w930] -> w912
              shift-left: i32[] [] -> [w931]
              tunnel: w914 -> [w933]
              i -> [w932]
              stop <- w937 stop-if-true
              n405 = String Subset(string=w936, length (rest)=4 ("length (rest)")) -> (substring=w941:string)  [unwired: 1 out]
              n406 = Match Pattern(string=w936, regular expression=" (") -> (before substring=w934:string)  [unwired: 4 out]
              n407 = Search 1D Array(1D array=w933, element=w934) -> (index of element=w929:i32)  [unwired: 1 out]
              n408 = Equal?(x="NOT ", y=w941) -> (x = y?=w928:bool)
              n409 = Equal?(x=w939, y=w932) -> (x = y?=w938:bool)
              n410 = Less Than 0?(x=w929) -> (x < 0?=w927:bool)
              n411 = Or(x=w928, y=w938) -> (x .or. y?=w937:bool)
              n412 = Compound Arithmetic op=AND(w927, invert w928) -> (w926:bool)
              n413 = case shown="False" w926 {
                tunnel: w932 -> [_ w946]
                tunnel: w931 -> [w943 w945]
                tunnel: [w943 w944] -> w930
                frame False {
                }
                frame True {
                  n414 = Build Array (concatenate)(w945, w946) -> (w944:i32[])
                }
              }
            }
            n415 = Array Size(array=w923) -> (size(s)=w925:i32)
            n416 = case shown="1" w925 {
              tunnel: [w947 w950] -> w924
              tunnel: w923 -> [_ w949]
              tunnel: i32[] [1] ("Filter Bins 1") -> [w947 w948]
              frame 0, Default {
              }
              frame 1 {
                n417 = Index Array(array=w949, index=0 ("Index")) -> (element=w952:i32)
                n418 = Greater Than 0?(x=w952) -> (x > 0?=w951:bool)
                n419 = Select(t=w949, s=w951, f=w948) -> (s? t:f=w950:i32[])
              }
            }
            n420 = local write "Filter Bins 1"(w924) -> ()
            n421 = local write "Filter Bins 2"(w912) -> ()
          }
        }
      }
      frame "Re Plot Data?" {
        n422 = while {
          tunnel: [w1000] -> w962
          shift-left: _ -> [w1002]
          shift-right: [w1001] -> _
          tunnel: [w1005] -> w968
          shift-left: _ -> [w1003]
          shift-right: [w1004] -> _
          tunnel: [w1009] -> w970
          shift-left: _ -> [w1008]
          shift-right: [w1007] -> w954
          tunnel: [w1010] -> w971
          shift-left: _ -> [w1012]
          shift-right: [w1011] -> _
          tunnel: [w1014] -> w972
          shift-left: _ -> [w1013]
          shift-right: [w1006] -> _
          tunnel: [w1015] -> w975
          tunnel: [w1016] -> w976
          shift-left: _ -> [w1017]
          shift-right: [w1018] -> _
          shift-left: _ -> [w1020]
          shift-right: [w1019] -> _
          tunnel: [w1021] -> w955
          shift-left: _ -> [w1022]
          shift-right: [w1023] -> _
          tunnel: [w998] -> w965
          shift-right: [w995] -> _
          shift-left: _ -> [w994]
          tunnel: [w997] -> w964
          shift-right: [w993] -> _
          shift-left: _ -> [w996]
          tunnel: [w990] -> w963
          shift-right: [w991] -> _
          shift-left: _ -> [w992]
          shift-right: [w988] -> _
          shift-left: _ -> [w989]
          tunnel: [w987] -> w957
          stop <- FALSE continue-if-true
          n423 = local read "Ordinate Name"() -> (w988:string)
          n424 = local read "Additional X Values"() -> (w995:dbl[])
          n425 = local read "Additional Y Values"() -> (w993:dbl[])
          n426 = local read "Intensity Plot?"() -> (w1007:bool)
          n427 = local read "color and symbol"() -> (w991:bool)
          n428 = local read "Accept Array"() -> (w1023:bool[][])
          n429 = local read "No of Contours"() -> (w1004:i32)
          n430 = local read "Point Size"() -> (w1001:i32)
          n431 = local read "Multi Ordinate"() -> (w1018:i32[])
          n432 = local read "Resolution"() -> (w1011:dbl)
          n433 = local read "Transpose"() -> (w1006:bool)
          n434 = local read "Absisca"() -> (w1019:u16)
          n435 = Equal?(x=w988, y=w989) -> (x = y?=w987:bool)
          n436 = Equal?(x=w1006, y=w1013) -> (x = y?=w1014:bool)
          n437 = Equal?(x=w991, y=w992) -> (x = y?=w990:bool)
          n438 = Equal?(x=w1004, y=w1003) -> (x = y?=w1005:bool)
          n439 = Equal?(x=w1001, y=w1002) -> (x = y?=w1000:bool)
          n440 = Equal?(x=w1011, y=w1012) -> (x = y?=w1010:bool)
          n441 = Equal?(x=w995, y=w994) -> (x = y?=w998:bool)
          n442 = Equal?(x=w993, y=w996) -> (x = y?=w997:bool)
          n443 = Equal?(x=w1019, y=w1020) -> (x = y?=w1016:bool)
          n444 = Equal?(x=w1023, y=w1022) -> (x = y?=w1021:bool)
          n445 = Equal?(x=w1007, y=w1008) -> (x = y?=w1009:bool)
          n446 = Equal?(x=w1018, y=w1017) -> (x = y?=w1015:bool)
        }
        n447 = global read "Results_plotter_Global.vi" "First Loop"() -> (w966:bool)
        n448 = while {
          shift-right: [w986] -> _
          shift-left: _ -> [w985]
          shift-right: [w983] -> _
          shift-left: _ -> [w984]
          tunnel: [w982] -> w961
          tunnel: [w981] -> w960
          stop <- FALSE continue-if-true
          n449 = local read "Filter Bins 1"() -> (w983:i32[])
          n450 = local read "Filter Bins 2"() -> (w986:i32[])
          n451 = Equal?(x=w983, y=w984) -> (x = y?=w981:bool)
          n452 = Equal?(x=w986, y=w985) -> (x = y?=w982:bool)
        }
        n453 = Not(x=w954) -> (.not. x?=w958:bool)
        n454 = property on="Resolution" class="DigNum (strict)"("Visible"=w954) -> ()  [unwired: 2 in, 2 out]
        n455 = property on="Bkgnd Value" class="DigNum (strict)"("Visible"=w954) -> ()  [unwired: 2 in, 2 out]
        n456 = property on="Intensity Graph" class="IntGraph (strict)"("Visible"=w954) -> ()  [unwired: 2 in, 2 out]
        n457 = property on="XY Plot" class="XYGraph (strict)"("Visible"=w958) -> ()  [unwired: 2 in, 2 out]
        n458 = Compound Arithmetic op=AND(w961, w960) -> (w959:bool)
        n459 = Compound Arithmetic op=AND(w957, w959, w962, w963, w968, w971, w972, w976, w975, w955, w970, w965, w964, invert w966) -> (w974:bool)
        n460 = Select(t="What to do next?", s=w974, f="Prepare for Plotting") -> (s? t:f=w973:string)
      }
      frame "Prepare for Plotting" {
        n461 = local read "Filter Array"() -> (w1032:u16[])
        n462 = local read "Multi Ordinate"() -> (w1027:i32[])
        n463 = Index Array(array=w1032, index=0 ("Index")) -> (element=w1029:u16)
        n464 = Equal To 0?(x=w1029) -> (x = 0?=w1030:bool)
        n465 = for {
          tunnel: w1027 -> [w1038] mode=indexing
          tunnel: [w1037] -> w1025 mode=indexing
          tunnel: w1026 -> [w1036]
          n466 = Index Array(array=w1036, index=w1038) -> (element=w1037:string)
        }
        n467 = case shown="False" w1030 {
          tunnel: w1029 -> [w1044 _]
          tunnel: w1026 -> [w1042 _]
          tunnel: [w1039 string[] []] -> w1024
          frame False {
            n468 = Decrement(x=w1044) -> (x-1=w1043:u16)
            n469 = local read "Filter Bins 1"() -> (w1046:i32[])
            n470 = property on="Filter bins 1" class="LstBox (strict)"() -> ("Item Names"=w1045:string[])  [unwired: 2 in, 2 out]
            n471 = Index Array(array=w1042, index=w1043) -> (element=w1040:string)
            n472 = for {
              tunnel: w1046 -> [w1049] mode=indexing
              tunnel: w1045 -> [w1048]
              tunnel: [w1047] -> w1041 mode=indexing
              n473 = Index Array(array=w1048, index=w1049) -> (element=w1047:string)
            }
            n474 = Build Array (concatenate)(w1040, w1041) -> (w1039:string[])
          }
          frame True {
          }
        }
        n475 = global write "Results_plotter_Global.vi" "Ordinate Strings"(w1025) -> ()
        n476 = global write "Results_plotter_Global.vi" "Filter 1 Strings"(w1024) -> ()
      }
      frame "Prepare Filter2 strings" {
        n477 = local read "Filter Array"() -> (w1057:u16[])
        n478 = Index Array(array=w1057, index=1 ("Index")) -> (element=w1054:u16)
        n479 = Equal To 0?(x=w1054) -> (x = 0?=w1055:bool)
        n480 = case shown="False" w1055 {
          tunnel: w1054 -> [w1066 _]
          tunnel: w1053 -> [w1064 _]
          tunnel: [w1061 string[] []] -> w1051
          frame False {
            n481 = Decrement(x=w1066) -> (x-1=w1065:u16)
            n482 = local read "Filter Bins 2"() -> (w1068:i32[])
            n483 = property on="Filter Bins 2" class="LstBox (strict)"() -> ("Item Names"=w1067:string[])  [unwired: 2 in, 2 out]
            n484 = Index Array(array=w1064, index=w1065) -> (element=w1062:string)
            n485 = for {
              tunnel: w1068 -> [w1071] mode=indexing
              tunnel: w1067 -> [w1070]
              tunnel: [w1069] -> w1063 mode=indexing
              n486 = Index Array(array=w1070, index=w1071) -> (element=w1069:string)
            }
            n487 = Build Array (concatenate)(w1062, w1063) -> (w1061:string[])
          }
          frame True {
          }
        }
        n488 = global write "Results_plotter_Global.vi" "Filter 2 Strings"(w1051) -> ()
      }
      frame "Plot Data" {
        n489 = stacked-sequence {
          seq-local: [w1078 _ _] -> [_ w1114 _]
          seq-local: [w1079 _ _] -> [_ w1113 _]
          tunnel: w1076 -> [_ w1123 _]
          tunnel: [_ TRUE _] -> w1075
          tunnel: [_ _ w1141] -> w1074
          tunnel: w1073 -> [w1080 _ _]
          frame #0 {
            n490 = global read "Results_plotter_Global.vi" "Ordinate Strings"() -> (w1078:string[])
            n491 = for {
              tunnel: w1078 -> [w1082] mode=indexing
              tunnel: w1080 -> [w1085]
              tunnel: [w1083] -> w1079 mode=indexing
              n492 = String Length(string=w1082) -> (length=w1081:i32)
              n493 = for {
                tunnel: w1082 -> [w1089]
                tunnel: w1085 -> [w1086] mode=indexing
                shift-right: [w1093] -> w1083
                shift-left: -1 -> [w1091]
                tunnel: w1081 -> [w1087]
                i -> [w1092]
                n494 = String Subset(string=w1086, length (rest)=w1087) -> (substring=w1088:string)  [unwired: 1 out]
                n495 = Equal?(x=w1088, y=w1089) -> (x = y?=w1090:bool)
                n496 = case shown="True" w1090 {
                  tunnel: [w1105 w1108] -> w1093
                  tunnel: w1092 -> [w1104 _]
                  tunnel: w1091 -> [w1103 w1108]
                  tunnel: w1087 -> [w1102 _]
                  tunnel: w1086 -> [w1101 _]
                  frame True {
                    n497 = String Subset(string=w1101, offset (0)=w1102) -> (substring=w1095:string)  [unwired: 1 out]
                    n498 = call <vilib>:"Trim Whitespace.vi"("string"=w1095) -> ("trimmed string"=w1094:string)  [unwired: 1 in]
                    n499 = Equal?(x=w1094, y="Err") -> (x = y?=w1097:bool)
                    n500 = Equal?(x=w1094, y="err") -> (x = y?=w1098:bool)
                    n501 = Or(x=w1097, y=w1098) -> (x .or. y?=w1096:bool)
                    n502 = case shown="True" w1096 {
                      tunnel: [w1106 w1107] -> w1105
                      tunnel: w1104 -> [w1106 _]
                      tunnel: w1103 -> [_ w1107]
                      frame True {
                      }
                      frame False {
                      }
                    }
                  }
                  frame False {
                  }
                }
              }
            }
          }
          frame #1 {
            n503 = global read "Results_plotter_Global.vi" "Filter 1 Strings"() -> (w1109:string[])
            n504 = global read "Results_plotter_Global.vi" "Filter 2 Strings"() -> (w1110:string[])
            n505 = local read "Accept Array"() -> (w1125:bool[][])
            n506 = local read "Multi Ordinate?"() -> (w1119:bool)
            n507 = Select(t=5, s=w1119, f=2 ("y")) -> (s? t:f=w1117:i32)
            n508 = global write "Results_plotter_Global.vi" "Ordinate"("Multi Ordinate") -> ()
            n509 = global write "Results_plotter_Global.vi" "Absisca"("Absisca") -> ()
            n510 = global write "Results_plotter_Global.vi" "Transpose"("Transpose") -> ()
            n511 = while {
              shift-right: [w1128] -> w1122
              shift-left: _ -> [w1129]
              tunnel: "color and symbol" -> [w1130]
              tunnel: w1117 -> [w1126]
              stop <- FALSE continue-if-true
              n512 = case shown="True" w1130 {
                tunnel: w1129 -> [w1137 w1139]
                tunnel: [w1136 w1139] -> w1128
                tunnel: w1126 -> [w1131 _]
                frame True {
                  n513 = Add(x=w1137, y=1) -> (x+y=w1134:i32)
                  n514 = local write "color and symbol"(FALSE ("color and symbol")) -> ()
                  n515 = Greater?(x=w1134, y=w1131) -> (0:w1135:bool)
                  n516 = Select(t=0, s=w1135, f=w1134) -> (s? t:f=w1136:i32)
                }
                frame False {
                }
              }
            }
            n517 = call "Plot_XY_data.vi"("Channel Values"=w1123, "Ordinate Strings"=w1114, "Swap color and symbol"=w1122, "Error Bar Chs"=w1113, "Accept Array"=w1125, "Filter 1 Strings"=w1109, "Filter 2 Strings"=w1110, "Ordinate"="Multi Ordinate", "Absisca"="Absisca", "Transpose"="Transpose") -> ("Accept Array Out"=→"Plotted Series":bool[][])  [unwired: 5 out]
          }
          frame #2 {
            n518 = Select(t="Intensity plot", s="Intensity Plot?", f="Add Legend and scales") -> (s? t:f=w1141:string)
            n519 = property on="Surface Area" class="DigNum (strict)"("Visible"="Intensity Plot?") -> ()  [unwired: 2 in, 2 out]
            n520 = property on="Surface Integral" class="DigNum (strict)"("Visible"="Intensity Plot?") -> ()  [unwired: 2 in, 2 out]
            n521 = property on="Surface Average" class="DigNum (strict)"("Visible"="Intensity Plot?") -> ()  [unwired: 2 in, 2 out]
            n522 = property on="X Ch Name" class="Ring (strict)"("Visible"="Intensity Plot?") -> ()  [unwired: 2 in, 2 out]
            n523 = property on="Y Ch Name" class="Ring (strict)"("Visible"="Intensity Plot?") -> ()  [unwired: 2 in, 2 out]
            n524 = property on="Z Ch Name" class="Ring (strict)"("Visible"="Intensity Plot?") -> ()  [unwired: 2 in, 2 out]
            n525 = property on="Point Size" class="Slide (strict)"("Visible"="Intensity Plot?") -> ()  [unwired: 2 in, 2 out]
            n526 = property on="No of Contours" class="DigNum (strict)"("Visible"="Intensity Plot?") -> ()  [unwired: 2 in, 2 out]
            n527 = property on="Slice mode" class="Enum (strict)"("Visible"="Intensity Plot?") -> ()  [unwired: 2 in, 2 out]
            n528 = property on="Plot Resolution" class="Bool (strict)"("Visible"="Intensity Plot?") -> ()  [unwired: 2 in, 2 out]
            n529 = property on="Update" class="Bool (strict)"("Visible"="Intensity Plot?") -> ()  [unwired: 2 in, 2 out]
          }
        }
      }
      frame "Add Legend and scales" {
        n530 = local read "Transpose"() -> (w1147:bool)
        n531 = global read "Results_plotter_Global.vi" "Plot Index values"() -> (w1150:dbl[][])
        n532 = global read "Results_plotter_Global.vi" "XY Graph Cluster"() -> (→"XY Plot":cluster{dbl[], dbl[]}[])
        n533 = Select(t=1 ("index (row)"), s=w1147, f=0 ("index (row)")) -> (s? t:f=w1144:i32)
        n534 = Index Array(array=w1150, index (row)=w1144) -> (element=w1149:dbl[])  [unwired: 1 in]
        n535 = Array Max & Min(array=w1149) -> (max value=w1148:dbl)  [unwired: 3 out]
        n536 = global read "Results_plotter_Global.vi" "Point info"() -> (w1155:T13)
        n537 = global read "Results_plotter_Global.vi" "Legend"() -> (w1156:string[])
        n538 = Greater?(x=w1148, y=2680560000.0) -> (0:w1152:bool)
        n539 = case shown="False" w1152 {
          tunnel: [w1167 u8 7 ("X Scale.Format & Precision:Precision")] -> w1151
          tunnel: w1148 -> [w1173 _]
          frame False {
            n540 = Absolute Value(x=w1173) -> (abs(x)=w1166:dbl)
            n541 = In Range and Coerce(upper limit=100000.0 ("y"), x=w1166, lower limit=0.0001) -> (In Range?=w1170:bool)  [unwired: 1 out]
            n542 = Select(t=u8 0 ("f"), s=w1170, f=u8 1) -> (s? t:f=w1167:u8)
          }
          frame True {
          }
        }
        n543 = local write "Warning!"("") -> ()
        n544 = for {
          tunnel: w1156 -> [w1193] mode=indexing
          tunnel: w1155 -> [w1190] mode=indexing
          tunnel: [w1191] -> w1160
          i -> [w1191]
          n545 = call "Abbreviate_string.vi"("Input String"=w1193, "Max String Length"=50) -> ("Output String"=w1184:string)
          n546 = String Length(string=w1184) -> (length=w1187:i32)
          n547 = Subtract(x=w1187, y=2) -> (x-y=w1185:i32)
          n548 = String Subset(string=w1184, length (rest)=w1185) -> (substring=w1183:string)  [unwired: 1 out]
          n549 = Unbundle By Name(w1190) -> ("Point Style"=w1189:u8, "Fill/Pt. Color"=w1188:u32)
          n550 = call "Fast_string_Replace.vi"("Replace match with:"="_", "Input String"=w1183, "regular expression"=" ") -> ("Output String"=w1182:string)  [unwired: 1 in, 1 out]
          n551 = property on="XY Plot" class="XYGraph (strict)"("Active Plot"=w1191, "Plot.Plot Name"=w1182, "Plot.Point Style"=w1189, "Plot.Fill/Point Color"=w1188, "Plot.Plot Color"=w1188) -> ()  [unwired: 2 in, 2 out]
        }
        n552 = Increment(x=w1160) -> (x+1=w1159:i32)
        n553 = property on="XY Plot" class="XYGraph (strict)"("X Scale.Format & Precision:Format"=w1151) -> ()  [unwired: 2 in, 2 out]
        n554 = for {
          N: 10 -> [_]
          tunnel: w1159 -> [w1178]
          i -> [w1179]
          w1175 = u32 0
          n555 = Add(x=w1178, y=w1179) -> (x+y=w1177:i32)
          n556 = property on="XY Plot" class="XYGraph (strict)"("Active Plot"=w1177, "Plot.Plot Name"="" ("Write Attribute"), "Plot.Plot Color"=w1175, "Plot.Fill/Point Color"=w1175) -> ()  [unwired: 2 in, 2 out]
        }
      }
      frame "Add Axis names" {
        n557 = local read "Multi Ordinate"() -> (w1208:i32[])
        n558 = for {
          tunnel: w1208 -> [w1225] mode=indexing
          shift-right: [w1222] -> w1201
          shift-left: "" -> [w1221]
          tunnel: w1209 -> [w1224]
          tunnel: [w1217] -> w1200
          i -> [w1217]
          n559 = Index Array(array=w1224, index=w1225) -> (element=w1223:string)
          n560 = String Length(string=w1221) -> (length=w1220:i32)
          n561 = Less?(x=w1220, y=40) -> (x < y?=w1218:bool)
          n562 = case shown="True" w1218 {
            tunnel: w1223 -> [_ w1230]
            tunnel: [w1226 w1229] -> w1222
            tunnel: w1221 -> [w1226 w1227]
            frame False {
            }
            frame True {
              n563 = Concatenate Strings(w1227, w1230, "   ") -> (w1229:string)
            }
          }
        }
        n564 = Greater Than 0?(x=w1200) -> (x > 0?=w1198:bool)
        n565 = local read "Transpose"() -> (w1211:bool)
        n566 = local read "Absisca"() -> (w1212:u16)
        n567 = Index Array(array=w1209, index=w1212) -> (element=w1210:string)
        n568 = String Length(string=w1201) -> (length=w1204:i32)
        n569 = Empty String/Path?(string/path="Ordinate Name") -> (empty?=w1199:bool)
        n570 = Subtract(x=w1204, y=3) -> (x-y=w1202:i32)
        n571 = Compound Arithmetic op=AND(invert w1199, w1198) -> (w1197:bool)
        n572 = String Subset(string=w1201, length (rest)=w1202) -> (substring=w1196:string)  [unwired: 1 out]
        n573 = Select(t="Ordinate Name", s=w1197, f=w1196) -> (s? t:f=w1194:string)
        n574 = case shown="False" w1211 {
          tunnel: [w1231 w1234] -> w1207
          tunnel: w1194 -> [w1232 w1234]
          tunnel: [w1232 w1233] -> w1206
          tunnel: w1210 -> [w1231 w1233]
          frame False {
          }
          frame True {
          }
        }
        n575 = global write "Results_plotter_Global.vi" "X Axis Name"(w1207) -> ()
        n576 = global write "Results_plotter_Global.vi" "Y Axis Name"(w1206) -> ()
        n577 = global write "Results_plotter_Global.vi" "Value plotted Name"(w1194) -> ()
        n578 = property on="XY Plot" class="XYGraph (strict)"("X Scale.Name Label.Text"=w1207, "Y Scale.Name Label.Text"=w1206) -> ()  [unwired: 2 in, 2 out]
      }
      frame "Intensity plot" {
        # "Max"
        # "Min"
        n579 = global read "Results_plotter_Global.vi" "XY Graph Cluster"() -> (w1235:cluster{dbl[], dbl[]}[])
        n580 = local read "Tolerances"() -> (w1240:dbl[])
        n581 = local read "Absisca"() -> (w1239:u16)
        n582 = local read "Transpose"() -> (w1236:bool)
        n583 = stacked-sequence {
          seq-local: [w1253 _ _ _ _ _ _ _ _ _ _ _ _] -> [_ _ _ w1318 w1325 _ w1350 _ _ _ _ _ _]
          seq-local: [_ w1269 _ _ _ _ _ _ _ _ _ _ _] -> [_ _ _ _ w1324 _ w1349 _ _ _ _ _ _]
          seq-local: [_ _ w1301 _ _ _ _ _ _ _ _ _ _] -> [_ _ _ _ _ _ w1358 _ _ _ _ _ _]
          seq-local: [_ _ _ _ _ _ w1360 _ _ _ _ _ _] -> [_ _ _ _ _ _ _ _ w1384 _ _ _ _]
          seq-local: [_ _ _ _ _ _ w1359 _ _ _ _ _ _] -> [_ _ _ _ _ _ _ _ w1385 _ _ _ _]
          seq-local: [_ w1265 _ _ _ _ _ _ _ _ _ _ _] -> [_ _ _ _ _ _ _ _ _ w1449 _ _ _]
          seq-local: [_ _ _ w1316 _ _ _ _ _ _ _ _ _] -> [_ _ _ _ w1323 _ w1354 _ _ _ _ _ _]
          seq-local: [_ _ _ _ _ _ _ _ _ _ _ w1475 _] -> [_ _ _ _ _ _ _ _ _ _ _ _ w1525]
          seq-local: [_ _ _ _ _ _ _ _ _ _ _ w1474 _] -> [_ _ _ _ _ _ _ _ _ _ _ _ w1526]
          seq-local: [_ _ _ w1315 _ _ _ _ _ _ _ _ _] -> [_ _ _ _ _ w1338 _ _ _ _ _ _ _]
          seq-local: [_ _ _ _ _ _ _ _ _ _ _ w1472 _] -> [_ _ _ _ _ _ _ _ _ _ _ _ w1518]
          tunnel: [_ _ _ TRUE _ _ _ _ _ _ _ _ _] -> w1246
          tunnel: [_ _ _ _ _ _ _ _ _ _ _ _ "Analyse Plot Space"] -> w1245
          tunnel: w1243 -> [w1250 _ _ _ _ _ _ _ _ _ _ _ _]
          tunnel: w1244 -> [w1251 _ w1302 _ _ _ _ _ _ w1430 _ _ _]
          tunnel: [w1251 _ _ _ _ _ _ _ _ _ _ _ _] -> w1242
          tunnel: [w1250 _ _ _ _ _ _ _ _ _ _ _ _] -> w1241
          tunnel: w1240 -> [w1255 _ _ _ _ _ _ _ _ _ _ _ _]
          tunnel: w1235 -> [w1254 _ _ w1320 _ _ _ _ _ _ _ _ _]
          tunnel: w1239 -> [w1252 _ _ _ _ _ _ _ _ w1446 _ _ _]
          tunnel: w1236 -> [w1249 _ _ w1317 _ _ w1362 _ _ w1444 _ _ _]
          tunnel: [_ w1270 _ _ _ _ _ _ _ _ _ _ _] -> w1238
          tunnel: w1237 -> [_ w1270 _ _ _ _ _ _ _ w1431 _ _ _]
          frame #0 {
            n584 = Not(x=w1249) -> (.not. x?=w1248:bool)
            n585 = for {
              tunnel: w1254 -> [w1264] mode=indexing
              tunnel: w1248 -> [w1261]
              shift-right: [w1259] -> w1256
              shift-left: dbl[] [] -> [w1260]
              n586 = Unbundle(w1264) -> (w1263:dbl[], w1262:dbl[])
              n587 = Select(t=w1263, s=w1261, f=w1262) -> (s? t:f=w1258:dbl[])
              n588 = Build Array (concatenate)(w1260, w1258) -> (w1259:dbl[])
            }
            n589 = Index Array(array=w1255, index=w1252) -> (element=w1247:dbl)
            n590 = call "Numeric_bins.vi"("Values"=w1256, "Tolerance"=w1247) -> ("Bin Centres"=w1253:dbl[])  [unwired: 2 out]
          }
          frame #1 {
            n591 = local read "Filter Bins 2"() -> (w1271:i32[])
            n592 = local read "Filter Bins 1"() -> (w1273:i32[])
            n593 = Array Size(array=w1271) -> (size(s)=w1275:i32)
            n594 = Array Size(array=w1273) -> (size(s)=w1276:i32)
            n595 = Greater?(x=w1276, y=w1275) -> (0:w1274:bool)
            n596 = case shown="True" w1274 {
              tunnel: w1273 -> [_ w1298]
              tunnel: [w1294 w1298] -> w1272
              tunnel: [w1295 w1297] -> w1267
              tunnel: w1271 -> [w1294 _]
              tunnel: [1 0] -> w1265
              frame False {
                n597 = property on="Filter Bins 2" class="LstBox (strict)"() -> ("Item Names"=w1295:string[])  [unwired: 2 in, 2 out]
              }
              frame True {
                n598 = property on="Filter Bins 1" class="LstBox (strict)"() -> ("Item Names"=w1297:string[])  [unwired: 2 in, 2 out]
              }
            }
            n599 = Array Size(array=w1267) -> (size(s)=w1266:i32)
            n600 = for {
              tunnel: w1272 -> [w1281] mode=indexing
              tunnel: w1267 -> [w1287]
              shift-right: [w1284] -> w1269
              shift-left: dbl[] [] -> [w1285]
              tunnel: w1266 -> [w1280]
              n601 = Index Array(array=w1287, index=w1281) -> (element=w1283:string)
              n602 = Less?(x=w1281, y=w1280) -> (x < y?=w1279:bool)
              n603 = Match Pattern(string=w1283, regular expression=" (0)") -> (offset past match=w1282:i32)  [unwired: 4 out]
              n604 = Less Than 0?(x=w1282) -> (x < 0?=w1278:bool)
              n605 = And(x=w1278, y=w1279) -> (x .and. y?=w1277:bool)
              n606 = case shown="True" w1277 {
                tunnel: w1285 -> [w1288 w1292]
                tunnel: [w1288 w1291] -> w1284
                tunnel: w1283 -> [_ w1290]
                frame False {
                }
                frame True {
                  n607 = Fract/Exp String To Number(string=w1290) -> (number=w1289:dbl)  [unwired: 4 out]
                  n608 = Build Array (concatenate)(w1292, w1289) -> (w1291:dbl[])
                }
              }
            }
          }
          frame #2 {
            n609 = local read "Template"() -> (w1300:path)
            n610 = call "Valid_Path.vi"("Filename"=w1300) -> ("Valid Path?"=w1299:bool)
            n611 = case shown="True" w1299 {
              tunnel: w1300 -> [_ w1312]
              tunnel: w1302 -> [_ w1311]
              tunnel: [nan w1308] -> w1301
              frame False {
              }
              frame True {
                n612 = local read "Multi Ordinate"() -> (w1307:i32[])
                n613 = call "Read_Write_Template.vi"("Template File"=w1312, "Mode"=Global_mode."Read Global", "Channel names In"=w1311, "Data type"="Minimum Value") -> ("1D Info Out"=w1310:string[])  [unwired: 4 in, 7 out]
                n614 = Index Array(array=w1307, index=0 ("Index")) -> (element=w1306:i32)
                n615 = Index Array(array=w1310, index=w1306) -> (element=w1309:string)
                n616 = Fract/Exp String To Number(string=w1309, default (0 dbl)=nan) -> (number=w1308:dbl)  [unwired: 3 out]
              }
            }
          }
          frame #3 {
            n617 = call "Grid_Data.vi"("Transpose"=w1317, "XY Graph"=w1320, "Bin Centres"=w1318) -> ("No of Duplicates"=w1315:i32, "Grided data"=w1316:dbl[][])
          }
          frame #4 {
            n618 = for {
              tunnel: w1325 -> [w1330]
              tunnel: w1324 -> [w1329] mode=indexing
              tunnel: w1323 -> [w1328] mode=indexing
              shift-right: [w1326] -> w1321
              shift-left: dbl[][] [] -> [w1327]
              n619 = for {
                tunnel: w1330 -> [w1336] mode=indexing
                tunnel: w1329 -> [w1331]
                tunnel: w1328 -> [w1335] mode=indexing
                shift-right: [w1332] -> w1326
                shift-left: w1327 -> [w1334]
                n620 = Build Array(w1336, w1331, w1335) -> (w1333:dbl[])
                n621 = Build Array (concatenate)(w1334, w1333) -> (w1332:dbl[][])
              }
            }
            n622 = global write "Results_plotter_Global.vi" "Intensity Plot data in rows"(w1321) -> ()
          }
          frame #5 {
            n623 = case shown="1, Default" w1338 {
              tunnel: w1338 -> [_ w1342]
              tunnel: ["" w1340] -> w1337
              frame 0 {
              }
              frame 1, Default {
                n624 = Format Into String(format string="The Intensity Plot has %d duplicate points which have been averaged together.", w1342) -> (resulting string=w1340:string)  [unwired: 2 in, 1 out]
              }
            }
            "Warning!" <- w1337
          }
          frame #6 {
            n625 = call "Insert_extra_rows_and_col.vi"("Row Values In"=w1349, "Additional Row Values"="Additional X Values", "Column Values In"=w1350, "Data In"=w1354, "Additional Column Values"="Additional Y Values") -> ("Row Values Out"=w1351:dbl[], "Column Values Out"=w1352:dbl[], "Data Out"=w1353:dbl[][])  [unwired: 2 out]
            n626 = Select(t="Resolution", s="Plot Resolution", f=0.0) -> (s? t:f=w1344:dbl)
            n627 = call "2D_interpolation.vi"("X Axis Current"=w1352, "Min Z Value In"=w1358, "Y axis Current"=w1351, "Bkgnd Value"="Bkgnd Value", "Plot In"=w1353, "Increment Value"=w1344, "Transpose"=w1362, "Point Size"="Point Size") -> ("min Z value"=w1360:dbl, "max Z value"=w1359:dbl, "Increment Value Out"=w1348:dbl, "Plot Out"=→"Intensity Graph":dbl[][])  [unwired: 4 out]
            n628 = local write "Resolution"(w1348) -> ()
          }
          frame #7 {
            n629 = global read "Results_plotter_Global.vi" "X Scale"() -> (w1370:cluster{"Xo":dbl, "delta X":dbl})
            n630 = global read "Results_plotter_Global.vi" "Y Scale"() -> (w1366:cluster{"Xo":dbl, "delta X":dbl})
            n631 = global read "Results_plotter_Global.vi" "Y Max"() -> (w1367:dbl)
            n632 = global read "Results_plotter_Global.vi" "X Max"() -> (w1368:dbl)
            n633 = Unbundle By Name(w1366) -> ("Xo"=w1365:dbl)
            n634 = Unbundle By Name(w1370) -> ("Xo"=w1369:dbl)
            n635 = Subtract(x=w1367, y=w1365) -> (x-y=w1371:dbl)
            n636 = Subtract(x=w1368, y=w1369) -> (x-y=w1380:dbl)
            n637 = Greater?(x=w1380, y=5.0) -> (0:w1378:bool)
            n638 = Greater?(x=w1371, y=5.0) -> (0:w1373:bool)
            n639 = Select(t=u8 0 ("Write Attribute"), s=w1378, f=u8 3) -> (s? t:f=w1364:u8)
            n640 = Select(t=u8 0 ("Write Attribute"), s=w1373, f=u8 3) -> (s? t:f=w1363:u8)
            n641 = property on="Intensity Graph" class="IntGraph (strict)"("X Scale.Offset and Multiplier"=w1370, "X Scale.Range:Maximum"=w1368, "Y Scale.Offset and Multiplier"=w1366, "Y Scale.Range:Maximum"=w1367, "X Scale.Format & Precision:Precision"=w1364, "Y Scale.Format & Precision:Precision"=w1363) -> ()  [unwired: 2 in, 2 out]
          }
          frame #8 {
            n642 = Greater Than 0?(x=w1385) -> (x > 0?=w1382:bool)
            n643 = Less Than 0?(x=w1384) -> (x < 0?=w1383:bool)
            n644 = And(x=w1382, y=w1383) -> (x .and. y?=w1381:bool)
            n645 = case shown="True" w1381 {
              tunnel: w1385 -> [w1414 w1428]
              tunnel: [w1422 w1426] -> w1387
              tunnel: w1384 -> [w1410 w1423]
              frame True {
                (unwired) u32 3743
                (unwired) u32 16721152
                n646 = Absolute Value(x=w1410) -> (abs(x)=w1409:dbl)
                n647 = Absolute Value(x=w1414) -> (abs(x)=w1416:dbl)
                n648 = Absolute Value(x=w1410) -> (abs(x)=w1417:dbl)
                n649 = Max & Min(x=w1416, y=w1417) -> (max(x,y)=w1412:dbl)  [unwired: 1 out]
                n650 = Divide(x=w1409, y=w1412) -> (x/y=w1403:dbl)
                n651 = Subtract(x=1.0, y=w1403) -> (x-y=w1402:dbl)
                n652 = Multiply(x=w1402, y=u32 255) -> (x*y=w1408:dbl)
                n653 = To Unsigned Long Integer(number=w1408) -> (unsigned 32bit integer=w1392:u32)
                n654 = Multiply(x=w1392, y=u32 256) -> (x*y=w1394:u32)
                n655 = Multiply(x=w1392, y=u32 65536) -> (x*y=w1391:u32)
                n656 = Compound Arithmetic op=ADD(w1391, w1394, u32 255) -> (w1390:u32)
                n657 = Bundle("min Z value"=w1410, w1390) -> (w1419:cluster{"min Z value":dbl, u32})  [unwired: 1 out]
                n658 = Divide(x=w1414, y=w1412) -> (x/y=w1407:dbl)
                n659 = Bundle("max Z value"=0.0, u32 16777215) -> (w1418:cluster{"max Z value":dbl, u32})  [unwired: 1 out]
                n660 = Subtract(x=1.0, y=w1407) -> (x-y=w1405:dbl)
                n661 = Multiply(x=w1405, y=u32 255) -> (x*y=w1401:dbl)
                n662 = To Unsigned Long Integer(number=w1401) -> (unsigned 32bit integer=w1388:u32)
                n663 = Multiply(x=w1388, y=u32 256) -> (x*y=w1398:u32)
                n664 = Compound Arithmetic op=ADD(w1388, w1398, u32 16711680) -> (w1389:u32)
                n665 = Bundle("max Z value"=w1414, w1389) -> (w1421:cluster{"max Z value":dbl, u32})  [unwired: 1 out]
                n666 = Build Array(w1421, w1419) -> (w1420:cluster{"min Z value":dbl, u32}[])
                n667 = Build Array (concatenate)(w1420, w1418) -> (w1422:cluster{"max Z value":dbl, u32}[])
              }
              frame False {
                n668 = Bundle("max Z value"=w1428, u32 16721152) -> (w1425:cluster{"max Z value":dbl, u32})  [unwired: 1 out]
                n669 = Bundle("min Z value"=w1423, u32 3743) -> (w1424:cluster{"min Z value":dbl, u32})  [unwired: 1 out]
                n670 = Build Array(w1425, w1424) -> (w1426:cluster{"min Z value":dbl, u32}[])
              }
            }
            n671 = property on="Intensity Graph" class="IntGraph (strict)"("Ignore Array"=FALSE ("Write Attribute"), "Z Scale.Marker Values[]"=w1387) -> ()  [unwired: 2 in, 2 out]
          }
          frame #9 {
            n672 = local read "Filter Array"() -> (w1448:u16[])
            n673 = Index Array(array=w1448, index=w1449) -> (element=w1447:u16)
            n674 = Decrement(x=w1447) -> (x-1=w1445:u16)
            n675 = local read "Multi Ordinate"() -> (w1435:i32[])
            n676 = Index Array(array=w1431, index=w1445) -> (element=w1439:string)
            n677 = Index Array(array=w1431, index=w1446) -> (element=w1438:string)
            n678 = case shown="False" w1444 {
              tunnel: [w1451 w1453] -> w1437
              tunnel: w1439 -> [w1451 w1452]
              tunnel: w1438 -> [w1450 w1453]
              tunnel: [w1450 w1452] -> w1436
              frame False {
              }
              frame True {
              }
            }
            n679 = Index Array(array=w1435, index=0) -> (element=w1433:i32)
            n680 = Index Array(array=w1430, index=w1433) -> (element=w1432:string)
            n681 = global write "Results_plotter_Global.vi" "Value plotted Name"(w1432) -> ()
            n682 = property on="Intensity Graph" class="IntGraph (strict)"("X Scale.Name Label.Text"=w1436, "Y Scale.Name Label.Text"=w1437) -> ()  [unwired: 2 in, 2 out]
            n683 = global write "Results_plotter_Global.vi" "Y Axis Name"(w1436) -> ()
            n684 = global write "Results_plotter_Global.vi" "X Axis Name"(w1437) -> ()
            n685 = Format Into String(format string="Add %s values", w1439) -> (resulting string=→"First Add label":string)  [unwired: 2 in, 1 out]
            n686 = Format Into String(format string="Add %s values", w1438) -> (resulting string=→"2nd Add label":string)  [unwired: 2 in, 1 out]
          }
          frame #10 {
            n687 = property on="Intensity Graph" class="IntGraph (strict)"() -> ("Color Table"=w1455:u32[])  [unwired: 2 in, 2 out]
            n688 = Increment(x="No of Contours") -> (x+1=w1456:i32)
            n689 = Divide(x=255, y=w1456) -> (x/y=w1460:dbl)
            n690 = To Long Integer(number=w1460) -> (32bit integer=w1459:i32)
            n691 = for {
              tunnel: w1459 -> [w1468]
              tunnel: [w1465] -> w1454 mode=indexing
              tunnel: w1455 -> [w1464] mode=indexing
              tunnel: u32 0 -> [w1463]
              i -> [w1469]
              n692 = Increment(x=w1469) -> (x+1=w1466:i32)
              n693 = Quotient & Remainder(x=w1466, y=w1468) -> (x-y*floor(x/y)=w1467:i32)  [unwired: 1 out]
              n694 = case shown="0" w1467 {
                tunnel: [w1470 w1471] -> w1465
                tunnel: w1464 -> [_ w1471]
                tunnel: w1463 -> [w1470 _]
                frame 0 {
                }
                frame 1, Default {
                }
              }
            }
            n695 = property on="Intensity Graph" class="IntGraph (strict)"("Ignore Array"=TRUE ("Write Attribute"), "Color Table"=w1454) -> ()  [unwired: 2 in, 2 out]
          }
          frame #11 {
            n696 = global read "Results_plotter_Global.vi" "Raw Interpolation"() -> (w1473:dbl[][])
            n697 = Add Array Elements(numeric array=w1473) -> (sum=w1472:dbl)
            n698 = Array Size(array=w1473) -> (size(s)=w1483:i32[])
            n699 = Decrement(x=w1483) -> (x-1=w1481:i32[])
            n700 = Index Array(array=w1481, index=0) -> (element=w1482:i32)
            n701 = Index Array(array=w1481, index=1) -> (element=w1478:i32)
            n702 = for {
              N: w1482 -> [_]
              tunnel: w1473 -> [w1491]
              tunnel: w1478 -> [w1490]
              shift-right: [w1486] -> w1475
              shift-left: 0.0 -> [w1487]
              shift-right: [w1485] -> w1474
              shift-left: 0 -> [w1484]
              i -> [w1489]
              n703 = Increment(x=w1489) -> (x+1=w1488:i32)
              n704 = for {
                N: w1490 -> [_]
                tunnel: w1491 -> [w1500]
                tunnel: w1489 -> [w1505]
                tunnel: w1488 -> [w1503]
                shift-right: [w1496] -> w1486
                shift-left: w1487 -> [w1495]
                shift-right: [w1492] -> w1485
                shift-left: w1484 -> [w1493]
                i -> [w1504]
                n705 = Increment(x=w1504) -> (x+1=w1502:i32)
                n706 = Index Array(array=w1500, index (row)=w1505, index (col)=w1502) -> (element=w1501:dbl)
                n707 = Index Array(array=w1500, index (row)=w1503, index (col)=w1502) -> (element=w1498:dbl)
                n708 = Index Array(array=w1500, index (row)=w1505, index (col)=w1504) -> (element=w1506:dbl)
                n709 = Index Array(array=w1500, index (row)=w1503, index (col)=w1504) -> (element=w1499:dbl)
                n710 = Compound Arithmetic op=ADD(w1506, w1501, w1499, w1498) -> (w1494:dbl)
                n711 = Not A Number/Path/Refnum?(number/path/refnum=w1494) -> (NaN/Path/Refnum?=w1497:bool)
                n712 = case shown="False" w1497 {
                  tunnel: [w1510 w1514] -> w1496
                  tunnel: w1495 -> [w1512 w1514]
                  tunnel: w1494 -> [w1511 _]
                  tunnel: [w1509 w1513] -> w1492
                  tunnel: w1493 -> [w1508 w1513]
                  frame False {
                    n713 = Add(x=w1511, y=w1512) -> (x+y=w1510:dbl)
                    n714 = Add(x=1, y=w1508) -> (x+y=w1509:i32)
                  }
                  frame True {
                  }
                }
              }
            }
          }
          frame #12 {
            n715 = local read "Resolution"() -> (w1527:dbl)
            n716 = Divide(x=w1525, y=4.0) -> (x/y=w1523:dbl)
            n717 = Multiply(x=w1527, y=w1527) -> (x*y=w1519:dbl)
            n718 = Multiply(x=w1519, y=w1518) -> ()  [unwired: 1 out]
            n719 = Multiply(x=w1519, y=w1526) -> (x*y=w1520:dbl)
            "Surface Area" <- w1520
            n720 = Multiply(x=w1519, y=w1523) -> (x*y=w1516:dbl)
            "Surface Integral" <- w1516
            n721 = global write "Results_plotter_Global.vi" "Surface Area"(w1520) -> ()
            n722 = global write "Results_plotter_Global.vi" "Surface Integral"(w1516) -> ()
            n723 = Divide(x=16666667, y=w1516) -> (x/y=→"Uadvec":dbl)
            n724 = Divide(x=w1516, y=w1520) -> (x/y=→"Surface Average":dbl)
          }
        }
      }
      frame "Analyse Plot Space" {
        n725 = case shown="True" "Show Plot Space Analysis" {
          tunnel: w1532 -> [_ w1542]
          tunnel: w1529 -> [_ w1541]
          frame False {
          }
          frame True {
            w1538 = TRUE  # Summarise All
            n726 = global read "Results_plotter_Global.vi" "Plot Index values"() -> (w1536:dbl[][])
            n727 = Index Array(array=w1536, index (row)=2) -> (element=w1535:dbl[])  [unwired: 1 in]
            n728 = To Long Integer(number=w1535) -> (32bit integer=w1534:i32[])
            n729 = for {
              tunnel: w1534 -> [w1545] mode=indexing
              tunnel: w1542 -> [w1544]
              tunnel: [w1543] -> w1539 mode=indexing
              n730 = Index Array(array=w1544, index (row)=w1545) -> (element=w1543:string[])  [unwired: 1 in]
            }
            n731 = call "Summarise.vi"("Channel Names"=w1541, "Data"=w1539, "Summarise All"=w1538) -> ("Summary"=w1540:string[][])  [unwired: 2 in]
            n732 = call "Plot_Space_Analysis.vi"("Table"=w1540) -> ()
          }
        }
      }
      frame "Vector Plot" {
        n733 = flat-sequence {
          tunnel: w1550 -> [w1552]
          tunnel: w1548 -> [w1551]
          frame #0 {
            n734 = local read "Template"() -> (w1553:path)
            n735 = call "Vector_Plotting.vi"("Template Filename"=w1553, "Data"=w1551, "Channel Names"=w1552) -> ()  [unwired: 1 out]
          }
          frame #1 {
            n736 = local write "Vector Plot?"(FALSE ("Vector Plot?")) -> ()
          }
        }
      }
      frame "What to do next?" {
        n737 = local read "Warning!"() -> (w1563:string)
        n738 = Empty String/Path?(string/path=w1563) -> (empty?=w1562:bool)
        n739 = Not(x=w1562) -> (.not. x?=w1561:bool)
        n740 = property on="Warning!" class="Str" props=["Visible", "Blinking", "Caption"]("Visible"=w1561, "Blinking"=w1561) -> ()  [unwired: 2 in, 3 out]
        n741 = case shown="False" "Add results file" {
          tunnel: [w1585 "More files options"] -> w1566
          tunnel: "Add results file" -> [_ _]
          tunnel: "Edit Template File" -> [w1576 _]
          frame False {
            n742 = Select(t="Edit template file", s=w1576, f="What to do next 2nd?") -> (s? t:f=w1574:string)
            n743 = Or(x="Save Plot data", y="Save Surface Fit") -> (x .or. y?=w1578:bool)
            n744 = Select(t="Save Plot Data", s=w1578, f=w1574) -> (s? t:f=w1581:string)
            n745 = Select(t="Create Plot summary", s="Save Plot as jpg", f=w1581) -> (s? t:f=w1572:string)
            n746 = Select(t="Save Data in Rows", s="Save Data in Rows", f=w1572) -> (s? t:f=w1585:string)
          }
          frame True {
            n747 = local write "Add results file"(FALSE) -> ()
          }
        }
        n748 = Select(t="End", s="stop", f=w1566) -> (s? t:f=w1557:string)
        n749 = Select(t="Vector Plot", s="Vector Plot?", f=w1557) -> (s? t:f=w1556:string)
      }
      frame "What to do next 2nd?" {
        n750 = local read "Empty"() -> (w1608:bool)
        n751 = local read "Last used Template"() -> (w1596:path)
        n752 = local read "Template"() -> (w1588:path)
        n753 = Select(t="Empty Results file array", s=w1608, f="What to do next 3rd?") -> (s? t:f=w1591:string)
        n754 = global write "Results_plotter_Global.vi" "Template"(w1588) -> ()
        n755 = Not Equal?(x=w1596, y=w1588) -> (x != y?=w1595:bool)
        n756 = Select(t="What type of row averaging?", s="Save Averaged rows", f=w1591) -> (s? t:f=w1603:string)
        n757 = case shown="True" "Delete Plotted data from file" {
          tunnel: [w1636 "Full Res file manipulator" ("t")] -> w1601
          tunnel: w1603 -> [w1636 _]
          frame False {
          }
          frame True {
            n758 = local write "Plotted rows only?"(TRUE ("Save Plotted rows only?")) -> ()
            n759 = local write "Mode"(Plotter_Mode."Delete unwanted rows" ("Mode")) -> ()
          }
        }
        n760 = case shown="False" "Add /Edit metadata" {
          tunnel: [w1613 w1628] -> w1593
          tunnel: w1601 -> [w1614 w1629]
          tunnel: w1599 -> [_ w1627]
          tunnel: "Reload Files" -> [w1615 _]
          tunnel: [string[] [] ("New Chs Out") w1621] -> w1590
          tunnel: [string[][] [] w1620] -> w1589
          frame False {
            n761 = Select(t="Initialise", s=w1615, f=w1614) -> (s? t:f=w1613:string)
          }
          frame True {
            n762 = local read "Result files to read"() -> (w1622:path[])
            n763 = call "Edit_Channel_Panel.vi"("All Channel names"=w1627, "Result files to read"=w1622) -> ("New Values Out"=w1635:string[], "New Chs Out"=w1621:string[], "Cancel Out"=w1624:bool, "Edit Raw Data Header Info Out"=w1618:bool, "Plotted rows only?"=w1634:bool, "Edit Raw data files?"=→"Edit Raw DF?":bool, "Raw data files in Orig Positions?"=→"Raw DF in Orig Pos?":bool, "Mode"=w1632:T4)  [unwired: 6 out]
            "Edit Raw Data Header Info" <- w1618
            n764 = Array Size(array=w1621) -> (size(s)=w1631:i32)
            n765 = Build Array(w1635) -> (w1620:string[][])
            n766 = local write "Add /Edit metadata"(FALSE ("Add /Edit metadata")) -> ()
            n767 = Greater Than 0?(x=w1631) -> (x > 0?=w1619:bool)
            n768 = local write "Plotted rows only?"(w1634) -> ()
            n769 = Or(x=w1618, y=w1619) -> (x .or. y?=w1617:bool)
            n770 = local write "Mode"(w1632) -> ()
            n771 = Compound Arithmetic op=AND(invert w1624, w1617) -> (w1623:bool)
            n772 = Select(t="Full Res file manipulator", s=w1623, f=w1629) -> (s? t:f=w1628:string)
          }
        }
        n773 = global write "Results_plotter_Global.vi" "New Chs In"(w1590) -> ()
        n774 = global write "Results_plotter_Global.vi" "New Values In"(w1589) -> ()
        n775 = Select(t="Initialise", s=w1595, f=w1593) -> (s? t:f=w1592:string)
      }
      frame "What to do next 3rd?" {
        n776 = local read "Show Results Space Analysis"() -> (w1651:bool)
        n777 = local read "Show Plot Space Analysis"() -> (w1650:bool)
        n778 = while {
          shift-right: [w1674] -> _
          shift-left: _ -> [w1673]
          shift-left: _ -> [w1672]
          shift-left: _ -> [w1671]
          tunnel: w1651 -> [w1674]
          shift-right: [w1679] -> _
          shift-left: _ -> [w1678]
          shift-left: _ -> [w1677]
          shift-left: _ -> [w1676]
          tunnel: w1650 -> [w1679]
          tunnel: [w1675] -> w1649
          tunnel: [w1670] -> w1648
          stop <- TRUE stop-if-true
          n779 = Compound Arithmetic op=AND(w1674, w1673, w1672, w1671) -> (w1670:bool)
          n780 = Compound Arithmetic op=AND(w1679, w1678, w1677, w1676) -> (w1675:bool)
        }
        n781 = Select(t="Run Calculation Routine", s="Calculate new metadata", f="Time to save setup?") -> (s? t:f=w1657:string)
        n782 = case shown="True" w1649 {
          frame False {
          }
          frame True {
            n783 = Open VI Reference(vi path="Plot_Space_Analysis.vi" ("VI path")) -> (vi reference=w1691:refnum<vi>, error out=w1690:errorcluster)  [unwired: 1 in, 4 out]
            n784 = property class="VI"(reference=w1691, error in=w1690) -> (reference out=w1689:refnum<vi>, error out=w1688:errorcluster, "Front Panel Window:Open"=w1686:bool)
            n785 = local write "Show Plot Space Analysis"(w1686) -> ()
            n786 = Close Reference(reference=w1689, error in (no error)=w1688) -> ()  [unwired: 1 out]
          }
        }
        n787 = case shown="True" w1648 {
          frame False {
          }
          frame True {
            n788 = Open VI Reference(vi path="Results_Space_Analysis.vi" ("VI path")) -> (vi reference=w1685:refnum<vi>, error out=w1684:errorcluster)  [unwired: 1 in, 4 out]
            n789 = property class="VI"(reference=w1685, error in=w1684) -> (reference out=w1683:refnum<vi>, error out=w1682:errorcluster, "Front Panel Window:Open"=w1680:bool)
            n790 = local write "Show Results Space Analysis"(w1680) -> ()
            n791 = Close Reference(reference=w1683, error in (no error)=w1682) -> ()  [unwired: 1 out]
          }
        }
        n792 = Select(t="Save Setup", s="Save Setup", f=w1657) -> (s? t:f=w1654:string)
        n793 = Select(t="Choose Setup file", s="Load Setup", f=w1654) -> (s? t:f=w1647:string)
        n794 = Or(x="Kill Point", y="Process Point") -> (x .or. y?=w1644:bool)
        n795 = Select(t="Process cursor point", s=w1644, f=w1647) -> (s? t:f=w1640:string)
        n796 = case shown="True" "Post Process Plotted Data" {
          tunnel: [w1665 "Full Res file manipulator" ("t")] -> w1641
          tunnel: w1640 -> [w1665 _]
          frame False {
          }
          frame True {
            n797 = local write "Plotted rows only?"(TRUE ("Plotted rows only?")) -> ()
            n798 = local write "Mode"(Plotter_Mode."Post Process Plotted Rows" ("Mode")) -> ()
          }
        }
      }
      frame "Time to save setup?" {
        n799 = stacked-sequence {
          seq-local: [w1701 _] -> [_ w1745]
          seq-local: [w1700 _] -> [_ w1744]
          tunnel: [w1709 _] -> w1694
          tunnel: w1693 -> [w1699 _]
          tunnel: [w1698 _] -> w1692
          frame #0 {
            n800 = while {
              shift-right: [w1731] -> _
              shift-left: _ -> [w1729]
              shift-right: [w1718] -> _
              shift-left: _ -> [w1726]
              tunnel: [w1718] -> w1708
              tunnel: [w1717] -> w1707
              shift-right: [w1719] -> _
              shift-left: _ -> [w1725]
              tunnel: [w1723] -> w1702
              tunnel: [w1720] -> w1703
              tunnel: [w1719] -> w1704
              tunnel: [w1716] -> w1700
              tunnel: w1699 -> [w1712]
              tunnel: [w1711] -> w1698
              stop <- FALSE continue-if-true
              n801 = Get Date/Time In Seconds() -> (seconds since 1Jan1904=w1727:timestamp)
              n802 = To Double Precision Float(number=w1727) -> (double precision float=w1730:dbl)
              n803 = local read "Show Plot Space Analysis"() -> (w1719:bool)
              n804 = Subtract(x=w1730, y=w1729) -> (x-y=w1733:dbl)
              n805 = local read "Show Results Space Analysis"() -> (w1718:bool)
              n806 = Greater?(x=w1733, y=600.0) -> (0:w1714:bool)
              n807 = Greater?(x=w1712, y=300) -> (0:w1710:bool)
              n808 = And(x=w1714, y=w1710) -> (x .and. y?=w1713:bool)
              n809 = case shown="False" w1713 {
                tunnel: [w1734 w1743] -> w1731
                tunnel: w1730 -> [w1735 w1743]
                tunnel: w1729 -> [w1736 _]
                tunnel: ["Check modification dates?" "Save Setup"] -> w1722
                tunnel: [TRUE w1740] -> w1711
                tunnel: w1710 -> [w1737 _]
                frame False {
                  n810 = Select(t=w1736, s=w1737, f=w1735) -> (s? t:f=w1734:dbl)
                }
                frame True {
                  n811 = global read "Trav_pos_global.vi" "Estimated Completion time"() -> (w1742:string)
                  n812 = Empty String/Path?(string/path=w1742) -> (empty?=w1740:bool)
                }
              }
              n813 = Not Equal?(x=w1719, y=w1725) -> (x != y?=w1720:bool)
              n814 = Not Equal?(x=w1718, y=w1726) -> (x != y?=w1717:bool)
              n815 = Compound Arithmetic op=AND(invert w1718, w1717) -> (w1716:bool)
              n816 = And(x=w1719, y=w1720) -> (x .and. y?=w1724:bool)
              n817 = Select(t="Analyse Plot Space", s=w1724, f=w1722) -> (s? t:f=w1723:string)
            }
            n818 = Compound Arithmetic op=AND(invert w1704, w1703) -> (w1701:bool)
            n819 = And(x=w1708, y=w1707) -> (x .and. y?=w1706:bool)
            n820 = Select(t="What is present?", s=w1706, f=w1702) -> (s? t:f=w1709:string)
          }
          frame #1 {
            n821 = case shown="True" w1744 {
              frame False {
              }
              frame True {
                n822 = Open VI Reference(vi path="Results_Space_Analysis.vi" ("VI path")) -> (vi reference=w1751:refnum<vi>, error out=w1750:errorcluster)  [unwired: 1 in, 4 out]
                n823 = property class="VI"(reference=w1751, error in=w1750, "Front Panel Window:Open"=FALSE) -> (reference out=w1749:refnum<vi>, error out=w1748:errorcluster)
                n824 = Close Reference(reference=w1749, error in (no error)=w1748) -> ()  [unwired: 1 out]
              }
            }
            n825 = case shown="True" w1745 {
              frame False {
              }
              frame True {
                n826 = Open VI Reference(vi path="Plot_Space_Analysis.vi" ("VI path")) -> (vi reference=w1757:refnum<vi>, error out=w1756:errorcluster)  [unwired: 1 in, 4 out]
                n827 = property class="VI"(reference=w1757, error in=w1756, "Front Panel Window:Open"=FALSE) -> (reference out=w1755:refnum<vi>, error out=w1754:errorcluster)
                n828 = Close Reference(reference=w1755, error in (no error)=w1754) -> ()  [unwired: 1 out]
              }
            }
          }
        }
      }
      frame "Check modification dates?" {
        n829 = while {
          shift-right: [w1777] -> _
          shift-left: _ -> [w1775]
          tunnel: [w1774] -> w1766
          stop <- FALSE continue-if-true
          n830 = Get Date/Time In Seconds() -> (seconds since 1Jan1904=w1772:timestamp)
          n831 = To Double Precision Float(number=w1772) -> (double precision float=w1776:dbl)
          n832 = Subtract(x=w1776, y=w1775) -> (x-y=w1780:dbl)
          n833 = Greater?(x=w1780, y=200.0) -> (0:w1778:bool)
          n834 = case shown="True" w1778 {
            tunnel: [w1782 w1785] -> w1777
            tunnel: w1776 -> [_ w1785]
            tunnel: w1775 -> [w1782 _]
            tunnel: [FALSE w1783] -> w1774
            frame False {
            }
            frame True {
              n835 = global read "Results_plotter_Global.vi" "First Loop"() -> (w1784:bool)
              n836 = Not(x=w1784) -> (.not. x?=w1783:bool)
            }
          }
        }
        n837 = Equal?(x="Tab Control", y=enum32{"Load ", "Plot ", "Save ", "Cursor"}."Cursor" ("Tab Control")) -> (x = y?=w1762:bool)
        n838 = global write "Results_plotter_Global.vi" "First Loop"(FALSE) -> ()
        n839 = Select(t="Read Cursor", s=w1762, f="Ordinate Selector Type") -> (s? t:f=w1760:string)
        n840 = Select(t="Files Modified?", s=w1766, f=w1760) -> (s? t:f=w1765:string)
      }
      frame "Files Modified?" {
        n841 = local read "nRows"() -> (w1789:i32)
        n842 = Less?(x=w1789, y=w1788) -> (x < y?=w1786:bool)
        n843 = case shown="True" w1786 {
          tunnel: [w1795 w1801] -> w1790
          tunnel: "Ordinate Selector Type" -> [w1795 w1796]
          frame False {
          }
          frame True {
            n844 = local read "Result files to read"() -> (w1800:path[])
            n845 = for {
              tunnel: w1800 -> [w1804] mode=indexing
              tunnel: [w1802] -> w1799 mode=indexing
              n846 = call "File_Modified_Since_Check.vi"("Pathname"=w1804, "Just Modified?"=TRUE) -> ("Modified?"=w1802:bool)
            }
            n847 = Or Array Elements(Boolean array=w1799) -> (logical OR=w1798:bool)
            n848 = Select(t="Initialise", s=w1798, f=w1796) -> (s? t:f=w1801:string)
          }
        }
      }
      frame "Read Cursor" {
        n849 = stacked-sequence {
          seq-local: [w1810 _] -> [_ w1845]
          tunnel: ["Ordinate Selector Type" _] -> w1808
          tunnel: [TRUE _] -> w1807
          tunnel: w1806 -> [_ w1844]
          tunnel: w1805 -> [_ w1843]
          frame #0 {
            n850 = property on="XY Plot" class="XYGraph (strict)"() -> ("Cursor.Cursor Position:Cursor X"=w1812:dbl, "Cursor.Cursor Position:Cursor Y"=w1811:dbl)  [unwired: 2 in, 2 out]
            n851 = local read "Transpose"() -> (w1825:bool)
            n852 = global read "Results_plotter_Global.vi" "Plot Index values"() -> (w1818:dbl[][])
            n853 = Index Array(array=w1818, index (row)=1) -> (element=w1816:dbl[])  [unwired: 1 in]
            n854 = Index Array(array=w1818, index (row)=2) -> (element=w1815:dbl[])  [unwired: 1 in]
            n855 = Index Array(array=w1818, index (row)=0) -> (element=w1817:dbl[])  [unwired: 1 in]
            n856 = case shown="True" w1825 {
              tunnel: [w1829 w1831] -> w1824
              tunnel: w1812 -> [w1829 w1830]
              tunnel: [w1828 w1830] -> w1823
              tunnel: w1811 -> [w1828 w1831]
              frame False {
              }
              frame True {
              }
            }
            n857 = for {
              tunnel: w1824 -> [w1840]
              tunnel: w1823 -> [w1839]
              tunnel: [w1834] -> w1822 mode=indexing
              tunnel: w1817 -> [w1833] mode=indexing
              tunnel: w1816 -> [w1832] mode=indexing
              n858 = Subtract(x=w1840, y=w1833) -> (x-y=w1838:dbl)
              n859 = Subtract(x=w1839, y=w1832) -> (x-y=w1837:dbl)
              n860 = Multiply(x=w1838, y=w1838) -> (x*y=w1835:dbl)
              n861 = Multiply(x=w1837, y=w1837) -> (x*y=w1836:dbl)
              n862 = Add(x=w1835, y=w1836) -> (x+y=w1834:dbl)
            }
            n863 = Array Max & Min(array=w1822) -> (min index (indices)=w1814:i32)  [unwired: 3 out]
            n864 = Index Array(array=w1815, index=w1814) -> (element=w1813:dbl)
            n865 = To Long Integer(number=w1813) -> (32bit integer=w1810:i32)
            "Cursor index" <- w1810
          }
          frame #1 {
            n866 = Index Array(array=w1844, index (row)=w1845) -> (element=w1842:string[])  [unwired: 1 in]
            n867 = for {
              tunnel: w1843 -> [w1853] mode=indexing
              tunnel: w1842 -> [w1846] mode=indexing
              tunnel: [w1852] -> w1841 mode=indexing
              n868 = while {
                shift-right: [w1865] -> _
                shift-left: w1846 -> [w1866]
                tunnel: [w1862] -> w1850
                tunnel: [w1861] -> w1848 mode=indexing
                i -> [w1862]
                stop <- w1863 continue-if-true
                n869 = Match Pattern(string=w1866, regular expression=":") -> (before substring=w1861:string, after substring=w1865:string, offset past match=w1864:i32)  [unwired: 2 out]
                n870 = Greater Than 0?(x=w1864) -> (x > 0?=w1863:bool)
              }
              n871 = Greater?(x=w1850, y=2) -> (0:w1849:bool)
              n872 = Reverse 1D Array(array=w1848) -> (reversed array=w1847:string[])
              n873 = case shown="True" w1849 {
                tunnel: w1853 -> [w1856 w1860]
                tunnel: [w1854 w1859] -> w1852
                tunnel: w1847 -> [_ w1858]
                tunnel: w1846 -> [w1855 w1857]
                frame False {
                  n874 = Build Array(w1856, w1855) -> (w1854:string[])
                }
                frame True {
                  n875 = Build Array (concatenate)(w1860, w1858, w1857) -> (w1859:string[])
                }
              }
            }
            "Table" <- w1841
          }
        }
      }
      frame "Process Cursor Point" {
        n876 = stacked-sequence {
          tunnel: [w1880] -> w1872
          tunnel: [TRUE] -> w1871
          tunnel: w1870 -> [_]
          tunnel: w1869 -> [_]
          tunnel: w1868 -> [w1881]
          frame #0 {
            n877 = local read "Kill Point"() -> (w1882:bool)
            n878 = global read "Results_plotter_Global.vi" "Row Reference"() -> (w1888:i32[][])
            n879 = local read "Cursor index"() -> (w1887:i32)
            n880 = Index Array(array=w1888, index (row)=w1887) -> (element=w1883:i32[])  [unwired: 1 in]
            n881 = local read "Result files to read"() -> (w1886:path[])
            n882 = Index Array(array=w1883, index #1=0 ("index"), index #2=1 ("index")) -> (element #1=w1885:i32, element #2=w1874:i32)
            n883 = Index Array(array=w1886, index=w1885) -> (element=w1879:path)
            n884 = call "GetRawDataFilePaths.vi"("Results file or Folder"=w1879) -> ("RawDataFilePaths"=w1878:string[])  [unwired: 9 in, 1 out]
            n885 = Index Array(array=w1878, index=w1874) -> (element=w1877:string)
            n886 = call "String_to_Pathname.vi"("Input String"=w1877) -> ("path"=w1876:path)
            n887 = case shown="False" w1882 {
              tunnel: w1879 -> [_ w1910]
              tunnel: w1874 -> [_ w1906]
              tunnel: w1881 -> [_ w1913]
              tunnel: ["What to do next?" ("t") w1912] -> w1880
              tunnel: w1876 -> [w1890 w1904]
              frame False {
                n888 = disable-structure shown="Enabled" {
                  disable-tunnel: w1890 -> [_ w1902]
                  frame Disabled {
                    n889 = local read "Table"() -> (w1901:string[][])
                    n890 = Index Array(array=w1901, index (col) #1=1 ("disabled index (col)"), index (col) #2=0 ("index (col)")) -> (element #1=w1894:string[], element #2=w1893:string[])  [unwired: 2 in]
                    n891 = Search 1D Array(1D array=w1893, element="Raw Data Filename") -> (index of element=w1897:i32)  [unwired: 1 in]
                    n892 = Index Array(array=w1894, index=w1897) -> (element=w1896:string)
                    n893 = call "String_to_Pathname.vi"("Input String"=w1896) -> ("path"=w1895:path)
                    n894 = call "Post_Process_Measurement.vi"("Raw data file"=w1895) -> ()  [unwired: 1 out]
                  }
                  frame Enabled {
                    n895 = call "Post_Process_Measurement.vi"("Raw data file"=w1902) -> ()  [unwired: 1 out]
                  }
                }
                n896 = local write "Process Point"(FALSE ("Kill Point")) -> ()
              }
              frame True {
                n897 = Strip Path(path=w1910) -> (name=w1905:string)  [unwired: 1 out]
                n898 = Strip Path(path=w1904) -> (name=w1903:string)  [unwired: 1 out]
                n899 = local read "nRows"() -> (w1915:i32)
                n900 = Format Into String(format string="Are you sure you want to remove the row in the results file \"%s\" generated from the raw data filename \"%s\"?", w1905, w1903) -> (resulting string=w1908:string)  [unwired: 2 in, 1 out]
                n901 = Less?(x=w1915, y=w1913) -> (x < y?=w1914:bool)
                n902 = Two Button Dialog(message=w1908) -> (T button?=w1907:bool)  [unwired: 2 out]
                n903 = case shown="True" w1914 {
                  tunnel: ["Create Selectors" "Initialise" ("t")] -> w1912
                  frame False {
                  }
                  frame True {
                  }
                }
                n904 = case shown="True" w1907 {
                  tunnel: w1910 -> [_ w1917]
                  tunnel: w1906 -> [_ w1916]
                  frame False {
                  }
                  frame True {
                    n905 = Build Array(w1916) -> (w1918:i32[])
                    n906 = call "Delete_unwanted_rows.vi"("Selected Rows"=w1918, "Filename"=w1917) -> ()  [unwired: 1 out]
                  }
                }
                n907 = local write "Kill Point"(FALSE ("Kill Point")) -> ()
              }
            }
          }
        }
      }
      frame "Edit template file" {
        n908 = stacked-sequence {
          frame #0 {
            n909 = local read "Template"() -> (w1927:path)
            n910 = call "Valid_Path.vi"("Filename"=w1927) -> ("Valid Path?"=w1926:bool)
            n911 = case shown="False" w1926 {
              tunnel: [T8."Edit Existing Template File" ("Mode") T8."Create New Template File" ("Mode")] -> w1930
              frame True {
              }
              frame False {
              }
            }
            n912 = local read "Results file"() -> (w1929:path)
            n913 = call "Edit_Template_File.vi"("Mode"=w1930, "Template Filename"=w1927, "Data Filename"=w1929) -> ("Template Filename Out"=w1928:path)  [unwired: 12 out]
            n914 = local write "Template"(w1928) -> ()
          }
          frame #1 {
            n915 = local read "Job Directory"() -> (w1933:path)
            n916 = Path To String(path=w1933) -> (string=w1936:string)
            n917 = call "Read_Write_Template.vi"("Mode"=Global_mode."Write Global to File", "Single Value In"=w1936, "Data type"="Log Folder Name" ("Variable name")) -> ()  [unwired: 5 in, 8 out]
            n918 = local write "Edit Template File"(FALSE ("Edit Template File")) -> ()
            n919 = Current VI's Path() -> (path=w1939:path)
            n920 = call "Open_Close_Front_Panel.ph.vi"("Front Panel Window:Open"=TRUE, "VI path"=w1939) -> ()  [unwired: 2 out]
          }
        }
      }
      frame "Save Plot Data" {
        n921 = global read "Results_plotter_Global.vi" "XY Graph Cluster"() -> (w1940:cluster{dbl[], dbl[]}[])
        n922 = local read "Tolerances"() -> (w1947:dbl[])
        n923 = local read "Absisca"() -> (w1946:u16)
        n924 = local read "Transpose"() -> (w1945:bool)
        n925 = local read "Multi Ordinate"() -> (w1944:i32[])
        n926 = global read "Results_plotter_Global.vi" "Precision"() -> (w1941:string[])
        n927 = stacked-sequence {
          seq-local: [w1958 _ _ _ _ _ _ _ _] -> [_ w1983 _ w2021 _ _ _ _ _]
          seq-local: [_ w1979 _ _ _ _ _ _ _] -> [_ _ _ _ _ _ _ w2143 _]
          seq-local: [_ _ _ _ _ w2073 _ _ _] -> [_ _ _ _ _ _ _ w2142 _]
          seq-local: [_ _ _ _ _ w2075 _ _ _] -> [_ _ _ _ _ _ w2111 _ _]
          seq-local: [_ _ _ w2019 _ _ _ _ _] -> [_ _ _ _ _ _ w2112 _ _]
          seq-local: [_ _ _ _ w2042 _ _ _ _] -> [_ _ _ _ _ w2068 _ _ _]
          seq-local: [w1955 _ _ _ _ _ _ _ _] -> [_ _ _ _ _ _ _ _ w2148]
          seq-local: [w1954 _ _ _ _ _ _ _ _] -> [_ w1971 _ _ _ _ _ _ _]
          seq-local: [_ _ w2000 _ _ _ _ _ _] -> [_ _ _ w2020 _ _ w2113 _ _]
          seq-local: [_ _ _ _ _ _ w2109 _ _] -> [_ _ _ _ _ _ _ w2140 _]
          tunnel: [_ _ _ _ _ _ _ _ TRUE] -> w1953
          tunnel: [_ _ _ _ _ _ _ _ w2146] -> w1952
          tunnel: w1950 -> [_ _ _ _ _ w2071 _ _ _]
          tunnel: w1951 -> [_ w1976 _ _ _ w2074 _ _ _]
          tunnel: [_ _ _ _ _ w2074 _ _ _] -> w1949
          tunnel: [_ _ _ _ _ w2071 _ _ _] -> w1948
          tunnel: w1947 -> [w1960 _ _ _ w2047 w2072 _ _ _]
          tunnel: w1940 -> [w1959 _ _ w2023 _ _ _ _ _]
          tunnel: w1946 -> [w1957 w1993 _ _ w2049 _ _ _ _]
          tunnel: w1945 -> [w1956 _ _ w2022 _ _ _ _ _]
          tunnel: w1944 -> [_ _ _ _ w2046 _ _ _ _]
          tunnel: [_ _ _ w2017 _ _ _ _ _] -> w1943
          tunnel: w1942 -> [_ _ w2003 w2017 _ _ _ _ _]
          tunnel: w1941 -> [_ _ _ w2016 _ w2067 _ _ _]
          frame #0 {
            n928 = local read "Save Surface Fit"() -> (w1955:bool)
            n929 = Not(x=w1956) -> (.not. x?=w1963:bool)
            n930 = for {
              tunnel: w1959 -> [w1970] mode=indexing
              tunnel: w1963 -> [w1967]
              shift-right: [w1965] -> w1961
              shift-left: dbl[] [] -> [w1966]
              n931 = Unbundle(w1970) -> (w1969:dbl[], w1968:dbl[])
              n932 = Select(t=w1969, s=w1967, f=w1968) -> (s? t:f=w1964:dbl[])
              n933 = Build Array (concatenate)(w1966, w1964) -> (w1965:dbl[])
            }
            n934 = Index Array(array=w1960, index=w1957) -> (element=w1954:dbl)
            n935 = call "Numeric_bins.vi"("Values"=w1961, "Tolerance"=w1954) -> ("Bin Centres"=w1958:dbl[])  [unwired: 2 out]
          }
          frame #1 {
            n936 = Index Array(array=w1976, index=w1993) -> (element=w1996:string)
            n937 = Match Pattern(string=w1996, regular expression=":") -> (before substring=w1995:string, after substring=w1994:string)  [unwired: 3 out]
            n938 = Concatenate Strings(w1995, " ", w1994, " =:" ("regular expression")) -> (w1978:string)
            n939 = Greater?(x=w1971, y=0.4) -> (0:w1991:bool)
            n940 = Greater?(x=w1971, y=0.09) -> (0:w1986:bool)
            n941 = call <vilib>:"Trim Whitespace.vi"("string"=w1978) -> ("trimmed string"=w1977:string)  [unwired: 1 in]
            n942 = Select(t=i16 0 ("precision (6)"), s=w1991, f=i16 2 ("precision (6)")) -> (s? t:f=w1987:i16)
            n943 = Select(t=w1987, s=w1986, f=i16 3) -> (s? t:f=w1984:i16)
            n944 = Number To Fractional String(number=w1983, precision (6)=w1984) -> (F-format string=w1982:string[])  [unwired: 2 out]
            n945 = for {
              tunnel: w1977 -> [w1999]
              tunnel: w1982 -> [w1997] mode=indexing
              tunnel: [w1998] -> w1981 mode=indexing
              n946 = Concatenate Strings(w1999, w1997) -> (w1998:string)
            }
            n947 = Build Array (concatenate)("Plot:Legend:" ("Input Element"), w1981, "End of:Plot Series:" ("Input Element")) -> (w1979:string[])
          }
          frame #2 {
            n948 = local read "Multi Ordinate?"() -> (w2002:bool)
            n949 = global read "Results_plotter_Global.vi" "Legend"() -> (w2001:string[])
            n950 = case shown="False" w2002 {
              tunnel: w2003 -> [w2007 _]
              tunnel: [w2004 w2015] -> w2000
              tunnel: w2001 -> [w2006 w2015]
              frame False {
                n951 = local read "Multi Ordinate"() -> (w2010:i32[])
                n952 = Index Array(array=w2010, index=0 ("Index")) -> (element=w2008:i32)
                n953 = Index Array(array=w2007, index=w2008) -> (element=w2005:string)
                n954 = for {
                  tunnel: w2006 -> [w2014] mode=indexing
                  tunnel: w2005 -> [w2013]
                  tunnel: [w2011] -> w2004 mode=indexing
                  n955 = Format Into String(format string="; %s", initial string=w2013, w2014) -> (resulting string=w2011:string)  [unwired: 1 in, 1 out]
                }
              }
              frame True {
              }
            }
          }
          frame #3 {
            n956 = call "Grid_Data.vi"("Transpose"=w2022, "XY Graph"=w2023, "Bin Centres"=w2021) -> ("Grided data"=w2018:dbl[][])  [unwired: 1 out]
            n957 = for {
              tunnel: w2020 -> [w2030] mode=indexing
              tunnel: [w2032] -> w2019 mode=indexing
              tunnel: w2018 -> [w2031] mode=indexing
              tunnel: w2017 -> [w2026]
              tunnel: w2016 -> [w2025]
              n958 = Match Pattern(string=w2030, regular expression=";") -> (before substring=w2027:string)  [unwired: 4 out]
              n959 = Search 1D Array(1D array=w2026, element=w2027) -> (index of element=w2028:i32)  [unwired: 1 out]
              n960 = Index Array(array=w2025, index=w2028) -> (element=w2024:string)
              n961 = for {
                tunnel: w2024 -> [w2037]
                tunnel: [w2036] -> w2033 mode=indexing
                tunnel: w2031 -> [w2034] mode=indexing
                n962 = Not A Number/Path/Refnum?(number/path/refnum=w2034) -> (NaN/Path/Refnum?=w2035:bool)
                n963 = case shown="True" w2035 {
                  tunnel: w2037 -> [w2040 _]
                  tunnel: [w2039 ""] -> w2036
                  tunnel: w2034 -> [w2038 _]
                  frame False {
                    n964 = call "Number_2_string.vi"("precision"=w2040, "number"=w2038) -> ("String"=w2039:string)
                  }
                  frame True {
                  }
                }
              }
              n965 = Build Array (concatenate)(w2030, w2033) -> (w2032:string[])
            }
          }
          frame #4 {
            n966 = Index Array(array=w2046, index=0 ("Index")) -> (element=w2044:i32)
            n967 = global read "Results_plotter_Global.vi" "Summarise"() -> (w2043:string[])
            n968 = for {
              shift-right: [w2056] -> w2042
              shift-left: i32[] [] -> [w2057]
              tunnel: w2049 -> [w2062]
              tunnel: w2044 -> [w2061]
              tunnel: w2047 -> [w2054] mode=indexing
              tunnel: w2043 -> [w2052] mode=indexing
              i -> [w2055]
              n969 = Equal?(x=w2061, y=w2055) -> (x = y?=w2060:bool)
              n970 = Not A Number/Path/Refnum?(number/path/refnum=w2054) -> (NaN/Path/Refnum?=w2053:bool)
              n971 = Equal?(x=w2062, y=w2055) -> (x = y?=w2059:bool)
              n972 = Equal?(x="FALSE", y=w2052) -> (x = y?=w2050:bool)
              n973 = Compound Arithmetic op=OR(w2059, w2060, w2053, w2050) -> (w2058:bool)
              n974 = case shown="False" w2058 {
                tunnel: w2057 -> [w2065 w2066]
                tunnel: [w2064 w2066] -> w2056
                tunnel: w2055 -> [w2063 _]
                frame False {
                  n975 = Build Array (concatenate)(w2065, w2063) -> (w2064:i32[])
                }
                frame True {
                }
              }
            }
          }
          frame #5 {
            n976 = local read "Plotted Series"() -> (w2070:bool[][])
            n977 = for {
              tunnel: w2072 -> [w2086]
              tunnel: [w2085] -> w2075 mode=indexing
              tunnel: w2068 -> [w2084]
              tunnel: w2071 -> [w2083]
              tunnel: w2070 -> [w2082] mode=indexing
              tunnel: i32[] [] -> [w2080]
              tunnel: w2067 -> [w2079]
              n978 = for {
                shift-right: [w2088] -> w2081
                shift-left: w2080 -> [w2089]
                tunnel: w2082 -> [w2087] mode=indexing
                i -> [w2090]
                n979 = case shown="True" w2087 {
                  tunnel: w2090 -> [_ w2094]
                  tunnel: w2089 -> [w2091 w2093]
                  tunnel: [w2091 w2092] -> w2088
                  frame False {
                  }
                  frame True {
                    n980 = Build Array (concatenate)(w2093, w2094) -> (w2092:i32[])
                  }
                }
              }
              n981 = for {
                tunnel: w2086 -> [w2102]
                tunnel: [w2103] -> w2085 mode=indexing
                tunnel: w2084 -> [w2097] mode=indexing
                tunnel: w2083 -> [w2100]
                tunnel: w2081 -> [w2099]
                tunnel: w2079 -> [w2096]
                n982 = for {
                  tunnel: w2099 -> [w2108] mode=indexing
                  tunnel: [w2107] -> w2104 mode=indexing
                  tunnel: w2097 -> [w2106]
                  tunnel: w2100 -> [w2105]
                  n983 = Index Array(array=w2105, index (row)=w2108, index (col)=w2106) -> (element=w2107:string)
                }
                n984 = Index Array(array=w2096, index=w2097) -> (element=w2098:string)
                n985 = Index Array(array=w2102, index=w2097) -> (element=w2101:dbl)
                n986 = call "Value_Occurence_Analysis.vi"("Average Numeric Values?"=FALSE, "Tolerance"=w2101, "Precision (3)"=w2098, "String Array"=w2104) -> ("Output String"=w2103:string)  [unwired: 2 out]
              }
            }
            n987 = for {
              tunnel: w2068 -> [w2078] mode=indexing
              tunnel: w2074 -> [w2077]
              tunnel: [w2076] -> w2073 mode=indexing
              n988 = Index Array(array=w2077, index=w2078) -> (element=w2076:string)
            }
          }
          frame #6 {
            n989 = for {
              shift-right: [w2126] -> w2109
              shift-left: string[][] [] -> [w2127]
              shift-right: [w2122] -> _
              shift-left: _ -> [w2123]
              tunnel: w2113 -> [w2124] mode=indexing
              tunnel: w2112 -> [w2116] mode=indexing
              tunnel: w2111 -> [w2115] mode=indexing
              i -> [w2121]
              n990 = Greater Than 0?(x=w2121) -> (x > 0?=w2120:bool)
              n991 = Match Pattern(string=w2124, regular expression="; ") -> (before substring=w2122:string)  [unwired: 4 out]
              n992 = Equal?(x=w2123, y=w2122) -> (x = y?=w2119:bool)
              n993 = Build Array (concatenate)(w2116, "", w2115) -> (w2114:string[])
              n994 = Compound Arithmetic op=AND(w2120, invert w2119) -> (w2118:bool)
              n995 = case shown="True" w2118 {
                tunnel: w2127 -> [w2131 w2134]
                tunnel: [w2130 w2133] -> w2126
                tunnel: w2114 -> [w2129 w2132]
                frame True {
                  n996 = Build Array (concatenate)(w2131, string[] [] ("array"), w2129) -> (w2130:string[][])
                }
                frame False {
                  n997 = Build Array (concatenate)(w2134, w2132) -> (w2133:string[][])
                }
              }
            }
          }
          frame #7 {
            w2139 = TRUE  # Simple Save?
            n998 = Build Array (concatenate)(w2143, w2142) -> (w2141:string[])
            n999 = local read "Header"() -> (w2136:string)
            n1000 = call "Write_output_file.vi"("Output filename"="Output Filename", "Header"=w2136, "Channel Names"=w2141, "Data"=w2140, "Simple Save?"=w2139, "Summarise mode"=T9."No data summary") -> ("Output filename Out"=w2137:path)  [unwired: 6 in, 3 out]
            n1001 = local write "Output Filename"(w2137) -> ()
          }
          frame #8 {
            n1002 = local write "Save Plot data"(FALSE ("Save Plot data")) -> ()
            n1003 = local write "Header"("") -> ()
            n1004 = Select(t="Save Surface Fit data", s=w2148, f="Create Selectors") -> (s? t:f=w2146:string)
          }
        }
      }
      frame "What type of row averaging?" {
        n1005 = Two Button Dialog(message="Do you want to Combine rows with identical positions together?", 1:"Just average series" ("F button name (\"Cancel\")"), 2:"Combine rows" ("T button name (\"OK\")")) -> (T button?=w2154:bool)
        n1006 = Select(t="Combine rows" ("T button name (\"OK\")"), s=w2154, f="Average Rows together") -> (s? t:f=w2151:string)
      }
      frame "Combine rows" {
        w2164 = TRUE  # Show panel ?
        n1007 = local read "Output Filename"() -> (w2163:path)
        n1008 = call "Combined_file_Panel.vi"("Show panel ?"=w2164, "Output filename"=w2163) -> ("Only Plotted data?"=w2165:bool, "Include Empty Rows? Out"=w2166:bool, "Give Audit Channels Out"=w2167:bool, "Output filename Out"=w2162:path)  [unwired: 5 out]
        n1009 = case shown="False" w2165 {
          tunnel: w2169 -> [w2178 w2181]
          tunnel: [w2178 w2179] -> w2168
          frame False {
          }
          frame True {
            n1010 = global read "Results_plotter_Global.vi" "Plot Index values"() -> (w2183:dbl[][])
            n1011 = Index Array(array=w2183, index (row)=2) -> (element=w2180:dbl[])  [unwired: 1 in]
            n1012 = for {
              tunnel: w2181 -> [w2186]
              tunnel: w2180 -> [w2185] mode=indexing
              tunnel: [w2184] -> w2179 mode=indexing
              n1013 = Index Array(array=w2186, index (row)=w2185) -> (element=w2184:string[])  [unwired: 1 in]
            }
          }
        }
        n1014 = local write "Save Averaged rows"(FALSE ("Save Plot data")) -> ()
        n1015 = local read "X Ch Name"() -> (w2173:u16)
        n1016 = local read "Y Ch Name"() -> (w2174:u16)
        n1017 = local read "Z Ch Name"() -> (w2175:u16)
        n1018 = call "Find_Rows_to_Combine.vi"("Include Empty Rows?"=w2166, "file path (dialog if empty)"=w2162, "Give Audit Channels"=w2167, "Full Channel Names"=w2172, "Data"=w2168, "Z Column Index"=w2175, "Y Column Index"=w2174, "X Column Index"=w2173) -> ()  [unwired: 4 out]
        n1019 = local write "Output Filename"(w2162) -> ()
      }
      frame "Average Rows together" {
        n1020 = global read "Results_plotter_Global.vi" "XY Graph Cluster"() -> (w2188:cluster{dbl[], dbl[]}[])
        n1021 = local read "Tolerances"() -> (w2194:dbl[])
        n1022 = local read "Absisca"() -> (w2193:u16)
        n1023 = local read "Transpose"() -> (w2192:bool)
        n1024 = global read "Results_plotter_Global.vi" "Precision"() -> (w2190:string[])
        n1025 = global read "Results_plotter_Global.vi" "Summarise"() -> (w2189:string[])
        n1026 = stacked-sequence {
          seq-local: [w2206 _ _ _ _] -> [_ w2223 _ _ _]
          seq-local: [_ w2226 _ _ _] -> [_ _ _ w2308 _]
          seq-local: [w2202 _ _ _ _] -> [_ w2224 _ _ _]
          seq-local: [_ _ w2286 _ _] -> [_ _ _ w2302 _]
          tunnel: [_ _ _ _ TRUE] -> w2200
          tunnel: [_ _ _ _ "Create Selectors"] -> w2199
          tunnel: w2197 -> [_ w2229 _ _ w2311]
          tunnel: w2198 -> [_ _ w2287 _ w2310]
          tunnel: [_ _ _ _ w2310] -> w2196
          tunnel: [_ _ _ _ w2311] -> w2195
          tunnel: w2194 -> [w2208 w2227 _ _ _]
          tunnel: w2188 -> [w2207 _ _ _ _]
          tunnel: w2193 -> [w2205 _ _ _ _]
          tunnel: w2192 -> [w2204 _ _ _ _]
          tunnel: w2191 -> [w2201 _ _ _ _]
          tunnel: w2190 -> [_ w2228 _ _ _]
          tunnel: w2189 -> [_ w2225 w2288 _ _]
          tunnel: [w2201 _ _ _ _] -> w2187
          frame #0 {
            n1027 = Not(x=w2204) -> (.not. x?=w2211:bool)
            n1028 = for {
              tunnel: w2207 -> [w2218] mode=indexing
              tunnel: w2211 -> [w2215]
              shift-right: [w2213] -> w2209
              shift-left: dbl[] [] -> [w2214]
              n1029 = Unbundle(w2218) -> (w2217:dbl[], w2216:dbl[])
              n1030 = Select(t=w2217, s=w2215, f=w2216) -> (s? t:f=w2212:dbl[])
              n1031 = Build Array (concatenate)(w2214, w2212) -> (w2213:dbl[])
            }
            n1032 = Index Array(array=w2208, index=w2205) -> (element=w2203:dbl)
            n1033 = call "Numeric_bins.vi"("Values"=w2209, "Tolerance"=w2203) -> ("Bin Centres"=w2206:dbl[], "Bin Index"=w2202:i32[])  [unwired: 1 out]
          }
          frame #1 {
            n1034 = Array Size(array=w2223) -> (size(s)=w2222:i32)
            n1035 = global read "Results_plotter_Global.vi" "Plot Index values"() -> (w2220:dbl[][])
            n1036 = Index Array(array=w2220, index (row)=2) -> (element=w2219:dbl[])  [unwired: 1 in]
            n1037 = for {
              N: w2222 -> [_]
              tunnel: w2229 -> [w2239]
              tunnel: w2228 -> [w2238]
              tunnel: w2227 -> [w2237]
              tunnel: [w2230] -> w2226 mode=indexing
              tunnel: w2225 -> [w2236]
              tunnel: w2224 -> [w2234]
              tunnel: w2219 -> [w2233]
              i -> [w2235]
              n1038 = stacked-sequence {
                seq-local: [w2243 _] -> [_ w2262]
                tunnel: w2239 -> [_ w2263]
                tunnel: w2238 -> [_ w2261]
                tunnel: w2237 -> [_ w2260]
                tunnel: w2236 -> [_ w2259]
                tunnel: w2235 -> [w2242 _]
                tunnel: w2234 -> [w2241 _]
                tunnel: w2233 -> [w2240 _]
                tunnel: [_ w2257] -> w2232
                tunnel: [_ w2256] -> w2231
                frame #0 {
                  n1039 = for {
                    shift-right: [w2249] -> w2243
                    shift-left: i32[] [] -> [w2250]
                    tunnel: w2242 -> [w2248]
                    tunnel: w2241 -> [w2247] mode=indexing
                    tunnel: w2240 -> [w2245] mode=indexing
                    n1040 = Equal?(x=w2247, y=w2248) -> (x = y?=w2246:bool)
                    n1041 = case shown="False" w2246 {
                      tunnel: w2250 -> [w2251 w2254]
                      tunnel: [w2251 w2255] -> w2249
                      tunnel: w2245 -> [_ w2252]
                      frame False {
                      }
                      frame True {
                        n1042 = To Long Integer(number=w2252) -> (32bit integer=w2253:i32)
                        n1043 = Build Array (concatenate)(w2254, w2253) -> (w2255:i32[])
                      }
                    }
                  }
                }
                frame #1 {
                  n1044 = for {
                    tunnel: w2263 -> [w2277]
                    tunnel: w2262 -> [w2276]
                    tunnel: w2261 -> [w2274] mode=indexing
                    tunnel: w2260 -> [w2273] mode=indexing
                    tunnel: [w2272] -> w2257 mode=indexing
                    tunnel: w2259 -> [w2269] mode=indexing
                    shift-right: [w2264] -> w2256
                    shift-left: string[] [] -> [w2265]
                    i -> [w2271]
                    n1045 = for {
                      tunnel: w2277 -> [w2285]
                      tunnel: w2276 -> [w2284] mode=indexing
                      tunnel: [w2283] -> w2275 mode=indexing
                      tunnel: w2271 -> [w2282]
                      n1046 = Index Array(array=w2285, index (row)=w2284, index (col)=w2282) -> (element=w2283:string)
                    }
                    n1047 = Equal?(x="TRUE", y=w2269) -> (x = y?=w2268:bool)
                    n1048 = Not(x=w2268) -> (.not. x?=w2267:bool)
                    n1049 = call "Value_Occurence_Analysis.vi"("Average Numeric Values?"=w2267, "Tolerance"=w2273, "Precision (3)"=w2274, "String Array"=w2275) -> ("St Dev"=w2266:string, "Output String"=w2272:string)  [unwired: 1 out]
                    n1050 = case shown="False" w2267 {
                      tunnel: w2266 -> [_ w2281]
                      tunnel: w2265 -> [w2278 w2280]
                      tunnel: [w2278 w2279] -> w2264
                      frame False {
                      }
                      frame True {
                        n1051 = Build Array (concatenate)(w2280, w2281) -> (w2279:string[])
                      }
                    }
                  }
                }
              }
              n1052 = Build Array (concatenate)(w2232, w2231) -> (w2230:string[])
            }
          }
          frame #2 {
            n1053 = for {
              tunnel: w2288 -> [w2293] mode=indexing
              shift-right: [w2289] -> w2286
              shift-left: w2287 -> [w2290]
              tunnel: w2287 -> [w2291] mode=indexing
              n1054 = Equal?(x="TRUE", y=w2293) -> (x = y?=w2292:bool)
              n1055 = case shown="False" w2292 {
                tunnel: w2291 -> [w2299 _]
                tunnel: w2290 -> [w2296 w2300]
                tunnel: [w2295 w2300] -> w2289
                frame False {
                  n1056 = Concatenate Strings(w2299, "St Dev") -> (w2297:string)
                  n1057 = Build Array (concatenate)(w2296, w2297) -> (w2295:string[])
                }
                frame True {
                }
              }
            }
          }
          frame #3 {
            w2305 = FALSE  # Save Plotted rows only?
            w2307 = TRUE  # Simple Save?
            n1058 = local read "Output Filename"() -> (w2303:path)
            n1059 = local read "Header"() -> (w2304:string)
            n1060 = local read "Template"() -> (w2306:path)
            n1061 = call "Write_output_file.vi"("Output filename"=w2303, "Header"=w2304, "Template Filename"=w2306, "Channel Names"=w2302, "Data"=w2308, "Simple Save?"=w2307, "Save Plotted rows only?"=w2305, "Summarise mode"=T9."No data summary") -> ("Output filename Out"=w2309:path)  [unwired: 4 in, 3 out]
            n1062 = local write "Output Filename"(w2309) -> ()
          }
          frame #4 {
            n1063 = local write "Save Averaged rows"(FALSE ("Save Plot data")) -> ()
          }
        }
      }
      frame "Save Surface Fit data" {
        n1064 = local read "Transpose"() -> (w2315:bool)
        n1065 = local read "Tolerances"() -> (w2322:dbl[])
        n1066 = local read "Absisca"() -> (w2321:u16)
        n1067 = global read "Results_plotter_Global.vi" "Precision"() -> (w2318:string[])
        n1068 = stacked-sequence {
          seq-local: [w2329 _ _ _ _ _] -> [_ w2348 _ _ _ _]
          seq-local: [_ w2345 _ _ _ _] -> [_ _ _ _ w2432 _]
          seq-local: [_ _ w2371 _ _ _] -> [_ _ _ _ w2451 _]
          seq-local: [w2330 _ _ _ _ _] -> [_ _ w2372 _ _ _]
          seq-local: [_ _ w2367 _ _ _] -> [_ _ _ _ w2435 _]
          seq-local: [_ _ w2366 _ _ _] -> [_ _ _ w2402 _ _]
          seq-local: [_ _ _ w2397 _ _] -> [_ _ _ _ w2433 _]
          tunnel: [_ _ _ _ _ TRUE] -> w2326
          tunnel: [_ _ _ _ _ "Create Selectors"] -> w2325
          tunnel: w2323 -> [_ _ _ _ _ w2457]
          tunnel: w2324 -> [_ w2333 _ _ _ w2458]
          tunnel: w2322 -> [_ w2359 _ _ _ _]
          tunnel: w2321 -> [_ w2360 _ _ _ _]
          tunnel: [_ _ w2377 _ _ _] -> w2320
          tunnel: w2319 -> [_ w2336 w2377 _ _ _]
          tunnel: w2318 -> [_ _ w2373 _ _ _]
          tunnel: [_ _ _ _ _ w2458] -> w2317
          tunnel: [_ _ _ _ _ w2457] -> w2316
          tunnel: w2315 -> [_ _ _ w2396 _ _]
          frame #0 {
            n1069 = global read "Results_plotter_Global.vi" "X Values"() -> (w2329:dbl[])
            n1070 = global read "Results_plotter_Global.vi" "Raw Interpolation"() -> (w2327:dbl[][])
            n1071 = global read "Results_plotter_Global.vi" "Y Values"() -> (w2328:dbl[])
            n1072 = Insert Into Array(array=w2327, index (col)=0 ("disabled index (col)"), new element=w2328) -> (w2330:dbl[][])  [unwired: 1 in]
          }
          frame #1 {
            n1073 = global read "Results_plotter_Global.vi" "Y Axis Name"() -> (w2335:string)
            n1074 = Search 1D Array(1D array=w2336, element=w2335) -> (index of element=w2334:i32)  [unwired: 1 out]
            n1075 = Index Array(array=w2333, index=w2334) -> (element=w2332:string)
            n1076 = Match Pattern(string=w2332, regular expression=":") -> (before substring=w2362:string, after substring=w2361:string)  [unwired: 3 out]
            n1077 = Index Array(array=w2359, index=w2360) -> (element=w2350:dbl)
            n1078 = Concatenate Strings(w2362, " ", w2361, " =:" ("regular expression")) -> (w2344:string)
            n1079 = Greater?(x=w2350, y=0.9) -> (0:w2357:bool)
            n1080 = Greater?(x=w2350, y=0.09) -> (0:w2352:bool)
            n1081 = call <vilib>:"Trim Whitespace.vi"("string"=w2344) -> ("trimmed string"=w2343:string)  [unwired: 1 in]
            n1082 = Select(t=i16 0 ("precision (6)"), s=w2357, f=i16 2 ("precision (6)")) -> (s? t:f=w2353:i16)
            n1083 = Select(t=w2353, s=w2352, f=i16 3) -> (s? t:f=w2349:i16)
            n1084 = Number To Fractional String(number=w2348, precision (6)=w2349) -> (F-format string=w2347:string[])  [unwired: 2 out]
            n1085 = for {
              tunnel: w2343 -> [w2365]
              tunnel: w2347 -> [w2363] mode=indexing
              tunnel: [w2364] -> w2338 mode=indexing
              n1086 = Concatenate Strings(w2365, w2363) -> (w2364:string)
            }
            n1087 = Build Array (concatenate)("Channel:Values:Plotted" ("Input Element"), "Axis:Name:" ("Input Element"), "Axis:Values:" ("Input Element"), w2338) -> (w2345:string[])
          }
          frame #2 {
            n1088 = global read "Results_plotter_Global.vi" "X Axis Name"() -> (w2370:string)
            n1089 = Concatenate Strings(w2370, " =" ("string")) -> (w2368:string)
            n1090 = local read "Multi Ordinate"() -> (w2376:i32[])
            n1091 = Index Array(array=w2376, index=0 ("Index")) -> (element=w2374:i32)
            n1092 = Index Array(array=w2373, index=w2374) -> (element=w2366:string)
            n1093 = Index Array(array=w2377, index=w2374) -> (element=w2367:string)
            n1094 = for {
              tunnel: w2367 -> [w2379]
              tunnel: [w2382] -> w2371 mode=indexing
              tunnel: w2366 -> [w2381]
              tunnel: w2372 -> [w2380] mode=indexing
              tunnel: w2368 -> [w2378]
              n1095 = for {
                tunnel: w2380 -> [w2385] mode=indexing
                tunnel: [w2384] -> w2383 mode=indexing
                tunnel: w2381 -> [w2387]
                n1096 = Not A Number/Path/Refnum?(number/path/refnum=w2385) -> (NaN/Path/Refnum?=w2386:bool)
                n1097 = case shown="False" w2386 {
                  tunnel: w2387 -> [w2390 _]
                  tunnel: w2385 -> [w2389 _]
                  tunnel: [w2388 ""] -> w2384
                  frame False {
                    n1098 = call "Number_2_string.vi"("precision"=w2390, "number"=w2389) -> ("String"=w2388:string)
                  }
                  frame True {
                  }
                }
              }
              n1099 = Build Array (concatenate)(w2379, w2378, w2383) -> (w2382:string[])
            }
          }
          frame #3 {
            w2401 = "\t"
            n1100 = global read "Results_plotter_Global.vi" "Intensity Plot data in rows"() -> (w2403:dbl[][])
            n1101 = global read "Results_plotter_Global.vi" "Value plotted Name"() -> (w2400:string)
            n1102 = global read "Results_plotter_Global.vi" "X Axis Name"() -> (w2394:string)
            n1103 = global read "Results_plotter_Global.vi" "Y Axis Name"() -> (w2393:string)
            n1104 = case shown="False" w2396 {
              tunnel: [w2404 w2407] -> w2395
              tunnel: w2394 -> [w2405 w2407]
              tunnel: w2393 -> [w2404 w2406]
              tunnel: [w2405 w2406] -> w2392
              frame False {
              }
              frame True {
              }
            }
            n1105 = Concatenate Strings(w2395, w2401, w2392, w2401, w2400, "\r\n") -> (w2398:string)
            n1106 = for {
              tunnel: w2403 -> [w2413] mode=indexing
              tunnel: w2402 -> [w2418]
              shift-right: [w2412] -> w2397
              shift-left: w2398 -> [w2417]
              n1107 = Index Array(array=w2413, index=0) -> (element=w2409:dbl)
              n1108 = Index Array(array=w2413, index=1) -> (element=w2408:dbl)
              n1109 = Index Array(array=w2413, index=2) -> (element=w2411:dbl)
              n1110 = Not A Number/Path/Refnum?(number/path/refnum=w2411) -> (NaN/Path/Refnum?=w2410:bool)
              n1111 = case shown="False" w2410 {
                tunnel: w2418 -> [w2429 _]
                tunnel: w2417 -> [w2428 w2430]
                tunnel: w2411 -> [w2427 _]
                tunnel: [w2426 w2430] -> w2412
                tunnel: w2409 -> [w2425 _]
                tunnel: w2408 -> [w2424 _]
                frame False {
                  w2420 = "\t"
                  n1112 = call "Number_2_string.vi"("number"=w2425) -> ("String"=w2423:string)  [unwired: 1 in]
                  n1113 = call "Number_2_string.vi"("number"=w2424) -> ("String"=w2422:string)  [unwired: 1 in]
                  n1114 = call "Number_2_string.vi"("precision"=w2429, "number"=w2427) -> ("String"=w2421:string)
                  n1115 = Concatenate Strings(w2428, w2423, w2420, w2422, w2420, w2421, "\r\n") -> (w2426:string)
                }
                frame True {
                }
              }
            }
          }
          frame #4 {
            w2447 = TRUE  # append to file? (new file:F)
            n1116 = global read "Results_plotter_Global.vi" "Surface Integral"() -> (w2446:dbl)
            n1117 = global read "Results_plotter_Global.vi" "Surface Area"() -> (w2445:dbl)
            n1118 = Initialize Array("", 10 ("Dimension Size")) -> (w2456:string[])
            n1119 = Divide(x=w2446, y=w2445) -> (x/y=w2444:dbl)
            n1120 = call "Asterisk_header.vi"("Channel names"=w2456) -> ("Header string"=w2434:string)
            n1121 = call "Value_to_string.vi"("Value"=w2446, "Label for value"="Surface Integral") -> ("Output string"=w2441:string)  [unwired: 1 in]
            n1122 = call "Value_to_string.vi"("Value"=w2445, "Label for value"="Surface Area") -> ("Output string"=w2442:string)  [unwired: 1 in]
            n1123 = call "Value_to_string.vi"("Value"=w2444, "Label for value"="Surface Average") -> ("Output string"=w2440:string)  [unwired: 1 in]
            n1124 = Concatenate Strings(w2442, w2441, w2440) -> (w2437:string)
            n1125 = call "Ch_names_to_rows.vi"("Channel Names"=w2432) -> ("3 Row names"=w2431:string[][])
            n1126 = local read "Output Filename"() -> (w2448:path)
            n1127 = Build Array (concatenate)(w2431, w2451) -> (w2449:string[][])
            n1128 = Array To Spreadsheet String(array=w2449, 3:"%s" ("format string")) -> (spreadsheet string=w2436:string)  [unwired: 1 out]
            n1129 = Format Into String(format string="\n%s\n\n%s\n%s\n\n\nInterpolated Surface of %s\n%s\n%s\n%s\n\n\n%s", w2434, w2433, w2434, w2435, w2434, w2436, w2434, w2437) -> (resulting string=w2439:string)  [unwired: 2 in, 1 out]
            n1130 = call "Write_Characters_To_File.vi"("file path (dialog if empty)"=w2448, "character string"=w2439, "append to file? (new file:F)"=w2447) -> ()  [unwired: 2 in, 4 out]
          }
          frame #5 {
            n1131 = local write "Save Surface Fit"(FALSE ("Save Plot data")) -> ()
          }
        }
      }
      frame "Save Data in Rows" {
        w2473 = TRUE  # Show panel ?
        n1132 = local read "Output Filename"() -> (w2470:path)
        n1133 = local write "Save Data in Rows"(FALSE ("Save All data")) -> ()
        n1134 = call "Output_file_Panel.vi"("Show panel ?"=w2473, "Channel Names"=w2468, "Header"="Header", "Output filename"=w2470) -> ("Save Full Res Data?"=w2465:bool, "Desired Columns"=w2474:i32[], "Header Out"=w2472:string, "Output filename Out"=w2476:path, "Channels to Tabulate in header Out"=w2462:i32[], "Save Plotted rows only?"=w2463:bool, "Summarise mode"=w2471:T9, "Grouping info"=w2464:T14[])
        "Plotted rows only?" <- w2463
        n1135 = case shown="False" w2465 {
          tunnel: w2476 -> [w2492 w2494]
          tunnel: w2474 -> [w2491 _]
          tunnel: w2472 -> [w2490 _]
          tunnel: w2463 -> [w2489 _]
          tunnel: w2471 -> [w2488 _]
          tunnel: w2469 -> [w2487 _]
          tunnel: w2468 -> [w2486 _]
          tunnel: [w2485 w2494] -> w2467
          tunnel: ["Create Selectors" "Is Filename Empty?"] -> w2466
          tunnel: w2464 -> [w2481 _]
          tunnel: w2462 -> [w2480 _]
          frame False {
            w2483 = FALSE  # Simple Save?
            n1136 = local read "Template"() -> (w2484:path)
            n1137 = call "Write_output_file.vi"("Output filename"=w2492, "Header"=w2490, "Template Filename"=w2484, "Channel Names"=w2486, "Data"=w2487, "Desired Columns"=w2491, "Simple Save?"=w2483, "Save Plotted rows only?"=w2489, "Summarise mode"=w2488, "Grouping info"=w2481, "Channels to Tabulate in header"=w2480) -> ("Output filename Out"=w2485:path)  [unwired: 1 in, 3 out]
          }
          frame True {
            "Mode" <- Plotter_Mode."Save file" ("Mode")
          }
        }
        n1138 = local write "Output Filename"(w2467) -> ()
      }
      frame "Is Filename Empty?" {
        # "This Express VI is the reason we can't strip object code from ResultsFilePlotter; may be able to convert to standard VI"
        n1139 = call "File Dialog"("start path"="Full_Res_Results_Folder", "prompt"="Please select a new or existing folder to save the results files in") -> ("selected path"=w2498:path, "cancelled"=w2496:bool)  [unwired: 5 in, 7 out]
        n1140 = local write "Full_Res_Results_Folder"(w2498) -> ()
        n1141 = case shown="False" w2496 {
          tunnel: ["Full Res file manipulator" ("f") "Create Selectors" ("t")] -> w2500
          frame False {
          }
          frame True {
          }
        }
      }
      frame "Check for overwrite or append" {
        n1142 = local read "Output Filename"() -> (w2514:path)
        n1143 = Format Into String(format string="Do you want to append to the result file\n\"%s\"" ("message"), w2514) -> (resulting string=w2509:string)  [unwired: 2 in, 1 out]
        n1144 = call <vilib>:"Three Button Dialog.vi"("Window Title (\"\")"="Output File Dialog" ("Window Title (\"\")"), "Right Button Text (\"Cancel\")"="Cancel" ("Button 3 Name"), "Center Button Text (\"No\")"="Overwrite" ("F button name (\"Cancel\")"), "Left Button Text (\"Yes\")"="Append" ("T button name (\"OK\")"), "message"=w2509) -> ("Which Button?"=w2508:T11)  [unwired: 6 out]
        n1145 = case shown="\"Center Button\"" w2508 {
          tunnel: w2514 -> [_ w2521 _]
          tunnel: ["Full Res file manipulator" "Full Res file manipulator" "Create Selectors" ("t")] -> w2507
          frame "Left Button" {
          }
          frame "Center Button" {
            n1146 = call "Delete_with_Check.vi"("FilePath"=w2521) -> ()  [unwired: 1 out]
          }
          frame "Right Button", Default {
          }
        }
      }
      frame "Create Plot summary" {
        w2536 = TRUE  # Summarise All
        n1147 = global read "Results_plotter_Global.vi" "Plot Index values"() -> (w2539:dbl[][])
        n1148 = local read "Intensity Plot?"() -> (w2535:bool)
        n1149 = global read "Results_plotter_Global.vi" "Row Reference"() -> (w2531:i32[][])
        n1150 = Index Array(array=w2531, index (col)=0 ("disabled index (col)")) -> (element=w2530:i32[])  [unwired: 1 in]
        n1151 = Index Array(array=w2539, index (row)=2) -> (element=w2541:dbl[])  [unwired: 1 in]
        n1152 = Select(t="Save Intensity plot as jpg", s=w2535, f="Create summary per series") -> (s? t:f=w2526:string)
        n1153 = To Long Integer(number=w2541) -> (32bit integer=w2538:i32[])
        n1154 = for {
          tunnel: w2546 -> [w2559]
          tunnel: [w2558] -> w2537 mode=indexing
          tunnel: w2538 -> [w2556] mode=indexing
          tunnel: w2530 -> [w2557]
          shift-right: [w2553] -> w2528
          shift-left: i32[] [] -> [w2554]
          n1155 = Index Array(array=w2557, index=w2556) -> (element=w2552:i32)
          n1156 = Search 1D Array(1D array=w2554, element=w2552) -> (index of element=w2555:i32)  [unwired: 1 out]
          n1157 = Index Array(array=w2559, index (row)=w2556) -> (element=w2558:string[])  [unwired: 1 in]
          n1158 = case shown="0, Default" w2555 {
            tunnel: w2552 -> [_ w2563]
            tunnel: w2554 -> [w2560 w2562]
            tunnel: [w2560 w2561] -> w2553
            frame 0, Default {
            }
            frame -1 {
              n1159 = Build Array (concatenate)(w2562, w2563) -> (w2561:i32[])
            }
          }
        }
        n1160 = local read "Result files to read"() -> (w2527:path[])
        n1161 = for {
          tunnel: w2528 -> [w2551] mode=indexing
          tunnel: w2527 -> [w2550]
          tunnel: [w2547] -> w2525 mode=indexing
          n1162 = Index Array(array=w2550, index=w2551) -> (element=w2549:path)
          n1163 = Strip Path(path=w2549) -> (name=w2548:string)  [unwired: 1 out]
          n1164 = call "Add_filename_suffix.vi"("Filename"=w2548) -> ("Base name"=w2547:string)  [unwired: 1 in, 3 out]
        }
        n1165 = call "Value_Occurence_Analysis.vi"("String Array"=w2525) -> ("Output String"=w2524:string)  [unwired: 3 in, 2 out]
        n1166 = global write "Results_plotter_Global.vi" "Current Data Filenames"(w2524) -> ()
        n1167 = call "Summarise.vi"("Channel Names"=w2542, "Data"=w2537, "Summarise All"=w2536) -> ("Summary"=w2544:string[][])  [unwired: 2 in]
        n1168 = global write "Results_plotter_Global.vi" "Plot Summary"(w2544) -> ()
      }
      frame "Create summary per series" {
        n1169 = global read "Results_plotter_Global.vi" "Plot Summary"() -> (w2565:string[][])
        n1170 = local read "Plotted Series"() -> (w2567:bool[][])
        n1171 = for {
          tunnel: w2567 -> [w2584] mode=indexing
          tunnel: i32[] [] -> [w2583]
          tunnel: w2572 -> [w2581]
          tunnel: w2569 -> [w2579]
          shift-right: [w2573] -> w2564
          shift-left: w2565 -> [w2575]
          w2578 = TRUE  # Summarise All
          n1172 = for {
            shift-right: [w2592] -> w2582
            shift-left: w2583 -> [w2593]
            tunnel: w2584 -> [w2591] mode=indexing
            i -> [w2594]
            n1173 = case shown="True" w2591 {
              tunnel: w2594 -> [_ w2598]
              tunnel: w2593 -> [w2595 w2597]
              tunnel: [w2595 w2596] -> w2592
              frame False {
              }
              frame True {
                n1174 = Build Array (concatenate)(w2597, w2598) -> (w2596:i32[])
              }
            }
          }
          n1175 = for {
            tunnel: w2582 -> [w2590] mode=indexing
            tunnel: w2581 -> [w2589]
            tunnel: [w2588] -> w2580 mode=indexing
            n1176 = Index Array(array=w2589, index (row)=w2590) -> (element=w2588:string[])  [unwired: 1 in]
          }
          n1177 = call "Summarise.vi"("Channel Names"=w2579, "Data"=w2580, "Summarise All"=w2578) -> ("Summary"=w2576:string[][])  [unwired: 2 in]
          n1178 = Index Array(array=w2576, index (col)=2 ("disabled index (col)")) -> (element=w2574:string[])  [unwired: 1 in]
          n1179 = for {
            tunnel: w2575 -> [w2587] mode=indexing
            tunnel: w2574 -> [w2586] mode=indexing
            tunnel: [w2585] -> w2573 mode=indexing
            n1180 = Build Array (concatenate)(w2587, w2586) -> (w2585:string[])
          }
        }
        n1181 = global write "Results_plotter_Global.vi" "Plot Summary"(w2564) -> ()
      }
      frame "Save Intensity plot as jpg" {
        n1182 = local read "Job Directory"() -> (w2605:path)
        n1183 = global read "Constants_global.vi" "EnFlo SW Folder"() -> (w2607:path)
        n1184 = Build Path(base path=w2607, name or relative path=path "Anemometry/Anemometry Sub Vis/Data_plotting_vis/Intensity Plot Vis") -> (appended path=w2601:path)
        n1185 = call "Remote_call_prep.vi"("Vi Name in"="Create picture Vi Name", "Job Directory In"=w2605, "VI Directory"=w2601) -> ("Vi Name out"=w2603:string, "Job Directory out"=w2600:path, "cancelled"=w2599:bool)
        n1186 = local write "Create picture Vi Name"(w2603) -> ()
        n1187 = local write "Job Directory"(w2600) -> ()
        n1188 = Build Path(base path=w2601, name or relative path=w2603) -> (appended path=w2602:path)
        n1189 = case shown="False" w2599 {
          tunnel: w2602 -> [w2616 _]
          tunnel: w2600 -> [w2615 _]
          frame False {
            n1190 = Open VI Reference(type specifier VI Refnum (for type only)="type specifier VI Refnum (for type only)", vi path=w2616) -> (vi reference=w2621:refnum<vi>, error out=w2620:errorcluster)  [unwired: 2 in, 2 out]
            n1191 = property class="VI Interface Type 0"(reference=w2621, error in=w2620, "Front Panel Window:Open"=TRUE) -> (reference out=w2617:refnum<vi>, error out=w2618:errorcluster)
            n1192 = local read "Intensity Graph"() -> (w2624:dbl[][])
            n1193 = local read "No of Contours"() -> (w2614:i32)
            n1194 = call-by-ref "?"(reference=w2617, error in=w2618, "No of Contours"=w2614, "Job Directory"=w2615, "Intensity Graph"=w2624) -> (reference out=w2623:refnum<vi>, error out=w2622:errorcluster)  [unwired: 3 in]
            n1195 = Close Reference(reference=w2623, error in (no error)=w2622) -> ()  [unwired: 1 out]
          }
          frame True {
          }
        }
        n1196 = local write "Save Plot as jpg"(FALSE ("Save All data")) -> ()
      }
      frame "Run Calculation Routine" {
        n1197 = stacked-sequence {
          seq-local: [w2633 _ _] -> [_ w2643 _]
          seq-local: [w2632 _ _] -> [_ w2644 _]
          tunnel: [_ w2642 _] -> w2627
          tunnel: w2626 -> [_ _ _]
          frame #0 {
            n1198 = global read "Constants_global.vi" "EnFlo SW Folder"() -> (w2639:path)
            n1199 = Build Path(base path=w2639, name or relative path=path "Anemometry/Anemometry Sub Vis/Data_plotting_vis/Calculation Vis") -> (appended path=w2636:path)
            n1200 = local read "Job Directory"() -> (w2635:path)
            n1201 = call "Remote_call_prep.vi"("Vi Name in"="...using routine", "Job Directory In"=w2635, "VI Directory"=w2636) -> ("Vi Name out"=w2637:string, "Job Directory out"=w2634:path, "cancelled"=w2633:bool)
            n1202 = local write "Job Directory"(w2634) -> ()
            n1203 = local write "...using routine"(w2637) -> ()
            n1204 = Build Path(base path=w2636, name or relative path=w2637) -> (appended path=w2632:path)
          }
          frame #1 {
            n1205 = case shown="False" w2643 {
              tunnel: w2644 -> [w2652 _]
              tunnel: [w2648 w2665] -> w2642
              tunnel: "What to do next?" -> [w2647 w2665]
              frame False {
                n1206 = Open VI Reference(type specifier VI Refnum (for type only)="VI Refnum Calculation", vi path=w2652) -> (vi reference=w2658:refnum<vi>, error out=w2657:errorcluster)  [unwired: 1 in, 3 out]
                n1207 = property class="VI Interface Type 1"(reference=w2658, error in=w2657, "Front Panel Window:Open"=TRUE) -> (reference out=w2654:refnum<vi>, error out=w2655:errorcluster)
                n1208 = call-by-ref "?"(reference=w2654, error in=w2655) -> (reference out=w2660:refnum<vi>, error out=w2659:errorcluster, "New Values In"=w2645:string[][], "New Chs In"=w2653:string[])  [unwired: 2 in]
                n1209 = for {
                  tunnel: w2653 -> [w2663] mode=indexing
                  tunnel: [w2662] -> w2646 mode=indexing
                  n1210 = call "Check_Ch_Name_colons.vi"("No of Colons"=2, "Ch Name in"=w2663) -> ("Ch Name out"=w2662:string)
                }
                n1211 = Empty String/Path?(string/path=w2646) -> (empty?=w2650:bool[])
                n1212 = Or Array Elements(Boolean array=w2650) -> (logical OR=w2649:bool)
                n1213 = Close Reference(reference=w2660, error in (no error)=w2659) -> ()  [unwired: 1 out]
                n1214 = Select(t=w2647, s=w2649, f="Input calculated values") -> (s? t:f=w2648:string)
                n1215 = global write "Results_plotter_Global.vi" "New Values In"(w2645) -> ()
                n1216 = global write "Results_plotter_Global.vi" "New Chs In"(w2646) -> ()
              }
              frame True {
              }
            }
          }
          frame #2 {
            w2668 = FALSE ("Raw DF in Orig Pos?")
            n1217 = local write "Edit Raw Data Header Info"(w2668) -> ()
            n1218 = local write "Calculate new metadata"(FALSE ("Save All data")) -> ()
            n1219 = local write "Plotted rows only?"(TRUE ("Plotted rows only?")) -> ()
            n1220 = local write "Raw DF in Orig Pos?"(w2668) -> ()
            n1221 = local write "Edit Raw DF?"(w2668) -> ()
            n1222 = local write "Mode"(Plotter_Mode."Edit values per row" ("Mode")) -> ()
          }
        }
      }
      frame "Input calculated values" {
        n1223 = local read "Result files to read"() -> (w2674:path[])
        n1224 = local read "Raw DF in Orig Pos?"() -> (w2671:bool)
        n1225 = stacked-sequence {
          seq-local: [w2678 _ _ _] -> [_ w2691 w2703 _]
          seq-local: [_ w2688 _ _] -> [_ _ w2704 _]
          tunnel: [_ _ _ w2756] -> w2676
          tunnel: w2674 -> [_ _ w2705 _]
          tunnel: w2673 -> [_ _ w2702 _]
          tunnel: w2672 -> [_ _ w2701 _]
          tunnel: w2671 -> [_ _ w2700 _]
          tunnel: w2670 -> [_ _ _ w2753]
          frame #0 {
            n1226 = global read "Results_plotter_Global.vi" "Plot Index values"() -> (w2681:dbl[][])
            n1227 = global read "Results_plotter_Global.vi" "Row Reference"() -> (w2682:i32[][])
            n1228 = Index Array(array=w2681, index (row)=2) -> (element=w2679:dbl[])  [unwired: 1 in]
            n1229 = for {
              tunnel: w2682 -> [w2686]
              tunnel: w2679 -> [w2685] mode=indexing
              tunnel: [w2684] -> w2678 mode=indexing
              n1230 = Index Array(array=w2686, index (row)=w2685) -> (element=w2684:i32[])  [unwired: 1 in]
            }
            n1231 = local write "Delete Plotted data from file"(FALSE ("Save All data")) -> ()
          }
          frame #1 {
            n1232 = Index Array(array=w2691, index (col)=0 ("disabled index (col)")) -> (element=w2687:i32[])  [unwired: 1 in]
            n1233 = for {
              shift-right: [w2693] -> w2688
              shift-left: i32[] [] -> [w2694]
              tunnel: w2687 -> [w2692] mode=indexing
              n1234 = Search 1D Array(1D array=w2694, element=w2692) -> (index of element=w2695:i32)  [unwired: 1 out]
              n1235 = case shown="-1" w2695 {
                tunnel: w2694 -> [w2696 w2699]
                tunnel: [w2696 w2698] -> w2693
                tunnel: w2692 -> [_ w2697]
                frame 0, Default {
                }
                frame -1 {
                  n1236 = Build Array (concatenate)(w2699, w2697) -> (w2698:i32[])
                }
              }
            }
          }
          frame #2 {
            n1237 = for {
              tunnel: w2705 -> [w2712]
              tunnel: w2704 -> [w2709] mode=indexing
              tunnel: w2703 -> [w2710]
              tunnel: w2702 -> [w2708]
              tunnel: w2701 -> [w2707]
              tunnel: w2700 -> [w2706]
              # "New Values"
              # "Row in file"
              n1238 = Index Array(array=w2712, index=w2709) -> (element=w2711:path)
              n1239 = stacked-sequence {
                seq-local: [w2717 _] -> [_ w2751]
                seq-local: [w2715 _] -> [_ w2746]
                tunnel: w2711 -> [_ w2752]
                tunnel: w2710 -> [w2719 _]
                tunnel: w2709 -> [w2718 _]
                tunnel: w2708 -> [_ _]
                tunnel: w2707 -> [_ _]
                tunnel: w2706 -> [_ w2750]
                frame #0 {
                  n1240 = global read "Results_plotter_Global.vi" "New Values In"() -> (w2713:string[][])
                  n1241 = for {
                    tunnel: w2718 -> [w2730]
                    tunnel: w2719 -> [w2726] mode=indexing
                    shift-right: [w2724] -> w2717
                    shift-left: i32[] [] -> [w2725]
                    shift-right: [w2723] -> w2715
                    shift-left: string[][] [] -> [w2722]
                    tunnel: w2713 -> [w2721]
                    i -> [w2720]
                    n1242 = Index Array(array=w2726, index=0) -> (element=w2728:i32)
                    n1243 = Equal?(x=w2728, y=w2730) -> (x = y?=w2727:bool)
                    n1244 = case shown="True" w2727 {
                      tunnel: w2726 -> [_ w2736]
                      tunnel: w2725 -> [w2732 w2741]
                      tunnel: [w2732 w2739] -> w2724
                      tunnel: w2722 -> [w2731 w2737]
                      tunnel: [w2731 w2738] -> w2723
                      tunnel: w2721 -> [_ w2734]
                      tunnel: w2720 -> [_ w2733]
                      frame False {
                      }
                      frame True {
                        n1245 = Index Array(array=w2734, index (row)=w2733) -> (element=w2735:string[])  [unwired: 1 in]
                        n1246 = Index Array(array=w2736, index=1) -> (element=w2740:i32)
                        n1247 = Build Array (concatenate)(w2741, w2740) -> (w2739:i32[])
                        n1248 = Build Array (concatenate)(w2737, w2735) -> (w2738:string[][])
                      }
                    }
                  }
                }
                frame #1 {
                  w2745 = FALSE  # Edit all Rows?
                  w2747 = FALSE  # Edit Raw DF?
                  w2748 = FALSE  # Edit Raw Data Header Info
                  w2749 = FALSE  # Value  Constant?
                  n1249 = global read "Results_plotter_Global.vi" "New Chs In"() -> (w2743:string[])
                  n1250 = local read "Job Directory"() -> (w2744:path)
                  n1251 = call "Add_Update_Values.vi"("Filename"=w2752, "Value  Constant?"=w2749, "Edit Raw data files?"=w2747, "New Chs In"=w2743, "Edit Raw Data Header Info"=w2748, "New Values In"=w2746, "Selected Rows"=w2751, "Edit all Rows?"=w2745, "Raw DF in Orig Pos?"=w2750, "Job Directory"=w2744) -> ()  [unwired: 1 in, 5 out]
                }
              }
            }
          }
          frame #3 {
            n1252 = local read "nRows"() -> (w2755:i32)
            n1253 = Less?(x=w2755, y=w2753) -> (x < y?=w2754:bool)
            n1254 = Current VI's Path() -> (path=w2757:path)
            n1255 = case shown="True" w2754 {
              tunnel: ["Create Selectors" "Initialise" ("t")] -> w2756
              frame False {
              }
              frame True {
              }
            }
            n1256 = call "Bring_to_front.vi"("path"=w2757) -> ()
          }
        }
      }
      frame "Save XY plot as jpg" {
        n1257 = local read "Create picture Vi Name"() -> (w2764:string)
        n1258 = local read "Job Directory"() -> (w2767:path)
        n1259 = global read "Constants_global.vi" "EnFlo SW Folder"() -> (w2769:path)
        n1260 = Build Path(base path=w2769, name or relative path=path "Anemometry/Anemometry Sub Vis/Data_plotting_vis/XY Plot Vis") -> (appended path=w2765:path)
        n1261 = call "Remote_call_prep.vi"("Vi Name in"=w2764, "Job Directory In"=w2767, "VI Directory"=w2765) -> ("Vi Name out"=w2766:string, "Job Directory out"=w2762:path, "cancelled"=w2761:bool)
        n1262 = local write "Create picture Vi Name"(w2766) -> ()
        n1263 = local write "Job Directory"(w2762) -> ()
        n1264 = Build Path(base path=w2765, name or relative path=w2766) -> (appended path=w2763:path)
        n1265 = case shown="False" w2761 {
          tunnel: [w2782 FALSE ("Saved Automatically?")] -> w2772
          tunnel: [w2781 path "" ("Plot data file")] -> w2771
          tunnel: [w2780 "" ("Tex Info String")] -> w2770
          tunnel: w2763 -> [w2779 _]
          tunnel: w2762 -> [w2778 _]
          frame False {
            n1266 = Open VI Reference(type specifier VI Refnum (for type only)="type specifier VI Refnum (for type only) 2", vi path=w2779) -> (vi reference=w2789:refnum<vi>, error out=w2788:errorcluster)  [unwired: 1 in, 3 out]
            n1267 = property class="VI Interface Type 2"(reference=w2789, error in=w2788, "Front Panel Window:Open"=TRUE) -> (reference out=w2785:refnum<vi>, error out=w2786:errorcluster)
            n1268 = global read "Results_plotter_Global.vi" "XY Graph Cluster"() -> (w2783:cluster{dbl[], dbl[]}[])
            n1269 = call-by-ref "?"(reference=w2785, error in=w2786, "Plot Array"=w2783, "Template"=w2778) -> (reference out=w2791:refnum<vi>, error out=w2790:errorcluster, "Saved Automatically?"=w2782:bool, "Tex Info String"=w2780:string, "Plot data file"=w2781:path)
            n1270 = Close Reference(reference=w2791, error in (no error)=w2790) -> ()  [unwired: 1 out]
          }
          frame True {
          }
        }
        n1271 = local write "Save Plot as jpg"(FALSE ("Save All data")) -> ()
        n1272 = case shown="True" w2772 {
          tunnel: w2771 -> [_ w2803]
          tunnel: [w2795 "Save Plot Data"] -> w2760
          tunnel: w2770 -> [_ w2801]
          frame False {
            n1273 = global read "Results_plotter_Global.vi" "New Chs In"() -> (w2800:string[])
            n1274 = Array Size(array=w2800) -> (size(s)=w2799:i32)
            n1275 = Greater Than 0?(x=w2799) -> (x > 0?=w2798:bool)
            n1276 = Select(t="Input calculated values", s=w2798, f="Create Selectors") -> (s? t:f=w2795:string)
          }
          frame True {
            n1277 = local write "Output Filename"(w2803) -> ()
            n1278 = local write "Header"(w2801) -> ()
          }
        }
      }
      frame "Full Res file manipulator" {
        n1279 = local read "Result files to read"() -> (w2813:path[])
        n1280 = local read "Output Filename"() -> (w2811:path)
        n1281 = local read "Mode"() -> (w2812:T4)
        n1282 = local read "Raw DF in Orig Pos?"() -> (w2807:bool)
        n1283 = local read "Plotted rows only?"() -> (w2810:bool)
        n1284 = global read "Results_plotter_Global.vi" "New Values In"() -> (w2804:string[][])
        n1285 = global read "Results_plotter_Global.vi" "New Chs In"() -> (w2805:string[])
        n1286 = stacked-sequence {
          seq-local: [w2818 _ _ _ _] -> [_ w2846 w2881 _ _]
          seq-local: [_ w2843 _ _ _] -> [_ _ w2882 _ _]
          seq-local: [_ w2838 _ _ _] -> [_ _ w2873 _ _]
          seq-local: [_ _ w2871 _ _] -> [_ _ _ w3084 _]
          seq-local: [_ _ w2870 _ _] -> [_ _ _ w3083 _]
          seq-local: [_ _ w2865 _ _] -> [_ _ _ w3080 _]
          tunnel: [_ _ _ w3087 _] -> w2815
          tunnel: w2813 -> [_ _ w2883 _ _]
          tunnel: w2812 -> [_ w2840 w2880 w3085 _]
          tunnel: w2811 -> [_ _ w2879 _ _]
          tunnel: w2810 -> [w2817 _ w2878 _ _]
          tunnel: w2805 -> [_ _ w2877 _ _]
          tunnel: w2809 -> [_ _ w2876 w3081 _]
          tunnel: w2808 -> [_ _ w2875 w3082 _]
          tunnel: w2807 -> [_ _ w2874 _ _]
          tunnel: w2806 -> [_ _ _ w3086 _]
          tunnel: w2804 -> [_ _ w2867 _ _]
          frame #0 {
            n1287 = global read "Results_plotter_Global.vi" "Row Reference"() -> (w2819:i32[][])
            n1288 = case shown="True" w2817 {
              tunnel: w2819 -> [w2821 w2822]
              tunnel: [w2821 w2823] -> w2818
              frame False {
              }
              frame True {
                n1289 = local read "Plotted Series"() -> (w2825:bool[][])
                n1290 = for {
                  tunnel: w2825 -> [w2832]
                  shift-right: [w2826] -> w2823
                  shift-left: i32[][] [] -> [w2828]
                  tunnel: w2822 -> [w2827] mode=indexing
                  i -> [w2831]
                  n1291 = Index Array(array=w2832, index (col)=w2831) -> (element=w2830:bool[])  [unwired: 1 in]
                  n1292 = Or Array Elements(Boolean array=w2830) -> (logical OR=w2829:bool)
                  n1293 = case shown="True" w2829 {
                    tunnel: w2828 -> [w2833 w2836]
                    tunnel: w2827 -> [_ w2835]
                    tunnel: [w2833 w2834] -> w2826
                    frame False {
                    }
                    frame True {
                      n1294 = Build Array (concatenate)(w2836, w2835) -> (w2834:i32[][])
                    }
                  }
                }
              }
            }
            n1295 = local write "Delete Plotted data from file"(FALSE ("Save All data")) -> ()
          }
          frame #1 {
            n1296 = local read "Job Directory"() -> (w2839:path)
            n1297 = case shown="\"Delete unwanted rows\", Default" w2840 {
              tunnel: [FALSE w2851] -> w2841
              tunnel: [w2847 w2849] -> w2838
              tunnel: w2839 -> [w2847 w2850]
              tunnel: [w2847 w2849] -> w2837
              frame "Post Process Plotted Rows" {
              }
              frame "Delete unwanted rows", Default {
                n1298 = call "Remote_call_prep.vi"("Job Directory In"=w2850) -> ("Job Directory out"=w2849:path)  [unwired: 2 in, 2 out]
                n1299 = local write "Job Directory"(w2849) -> ()
                n1300 = Not Equal?(x=w2850, y=w2849) -> (x != y?=w2851:bool)
              }
            }
            n1301 = Index Array(array=w2846, index (col)=0 ("disabled index (col)")) -> (element=w2842:i32[])  [unwired: 1 in]
            n1302 = for {
              shift-right: [w2858] -> w2843
              shift-left: i32[] [] -> [w2859]
              tunnel: w2842 -> [w2857] mode=indexing
              n1303 = Search 1D Array(1D array=w2859, element=w2857) -> (index of element=w2860:i32)  [unwired: 1 out]
              n1304 = case shown="-1" w2860 {
                tunnel: w2859 -> [w2861 w2864]
                tunnel: [w2861 w2863] -> w2858
                tunnel: w2857 -> [_ w2862]
                frame 0, Default {
                }
                frame -1 {
                  n1305 = Build Array (concatenate)(w2864, w2862) -> (w2863:i32[])
                }
              }
            }
            n1306 = case shown="True" w2841 {
              tunnel: w2837 -> [_ w2853]
              frame False {
              }
              frame True {
                n1307 = local read "Template"() -> (w2852:path)
                n1308 = Path To String(path=w2853) -> (string=w2856:string)
                n1309 = call "Read_Write_Template.vi"("Template File"=w2852, "Mode"=Global_mode."Write Global to File", "Single Value In"=w2856, "Data type"="Log Folder Name" ("Variable name")) -> ()  [unwired: 4 in, 8 out]
              }
            }
          }
          frame #2 {
            w2869 = path[] []
            n1310 = local read "Full_Res_Results_Folder"() -> (w2868:path)
            n1311 = for {
              tunnel: w2883 -> [w2905]
              tunnel: w2882 -> [w2902] mode=indexing
              tunnel: w2881 -> [w2903]
              tunnel: w2880 -> [w2901]
              tunnel: w2879 -> [w2900]
              tunnel: w2878 -> [w2899]
              tunnel: w2877 -> [w2898]
              tunnel: w2876 -> [w2897]
              tunnel: w2875 -> [w2896]
              tunnel: w2874 -> [w2895]
              tunnel: w2873 -> [w2894]
              shift-right: [w2893] -> _
              shift-left: FALSE -> [w2892]
              shift-right: [w2890] -> w2871
              shift-left: w2869 -> [w2891]
              shift-right: [w2888] -> w2870
              shift-left: w2869 -> [w2889]
              tunnel: w2868 -> [w2887]
              tunnel: w2867 -> [w2886]
              shift-right: [w2884] -> w2865
              shift-left: i32[] [] -> [w2885]
              # "Row No in file"
              # "Row No in plotter"
              n1312 = Index Array(array=w2905, index=w2902) -> (element=w2904:path)
              n1313 = stacked-sequence {
                seq-local: [w2908 _ _ _] -> [_ w2936 w2985 _]
                seq-local: [_ w2934 _ _] -> [_ _ w2984 _]
                seq-local: [w2906 _ _ _] -> [_ _ w2977 w3078]
                tunnel: w2904 -> [_ w2935 w2986 _]
                tunnel: w2903 -> [w2910 _ _ _]
                tunnel: w2902 -> [w2909 _ _ _]
                tunnel: w2901 -> [_ w2933 w2983 _]
                tunnel: w2900 -> [_ _ w2982 _]
                tunnel: w2899 -> [_ _ w2981 _]
                tunnel: w2898 -> [_ _ w2980 _]
                tunnel: w2897 -> [_ _ w2979 _]
                tunnel: w2896 -> [_ _ w2978 _]
                tunnel: w2895 -> [_ _ w2976 _]
                tunnel: w2894 -> [_ _ w2975 _]
                tunnel: [_ w2932 _ _] -> w2893
                tunnel: w2892 -> [_ w2931 _ _]
                tunnel: w2891 -> [_ _ w2974 _]
                tunnel: [_ _ w2973 _] -> w2890
                tunnel: w2889 -> [_ _ w2972 _]
                tunnel: [_ _ w2971 _] -> w2888
                tunnel: w2887 -> [_ _ w2970 _]
                tunnel: w2886 -> [_ _ w2969 _]
                tunnel: w2885 -> [_ _ _ w3079]
                tunnel: [_ _ _ w3077] -> w2884
                frame #0 {
                  w2907 = i32[] []
                  n1314 = for {
                    tunnel: w2909 -> [w2919]
                    tunnel: w2910 -> [w2915] mode=indexing
                    shift-right: [w2913] -> w2908
                    shift-left: w2907 -> [w2914]
                    shift-right: [w2912] -> w2906
                    shift-left: w2907 -> [w2911]
                    n1315 = Index Array(array=w2915, index=0) -> (element=w2917:i32)
                    n1316 = Equal?(x=w2917, y=w2919) -> (x = y?=w2916:bool)
                    n1317 = case shown="True" w2916 {
                      tunnel: w2915 -> [_ w2923]
                      tunnel: w2914 -> [w2921 w2929]
                      tunnel: [w2921 w2927] -> w2913
                      tunnel: w2911 -> [w2920 w2925]
                      tunnel: [w2920 w2926] -> w2912
                      frame False {
                      }
                      frame True {
                        n1318 = Index Array(array=w2923, index=2) -> (element=w2922:i32)
                        n1319 = Build Array (concatenate)(w2925, w2922) -> (w2926:i32[])
                        n1320 = Index Array(array=w2923, index=1) -> (element=w2928:i32)
                        n1321 = Build Array (concatenate)(w2929, w2928) -> (w2927:i32[])
                      }
                    }
                  }
                }
                frame #1 {
                  n1322 = case shown="\"Post Process Plotted Rows\"" w2933 {
                    tunnel: w2936 -> [_ _ _ _ _ w2952]
                    tunnel: w2935 -> [_ _ _ _ _ w2950]
                    tunnel: [TRUE ("T button?") TRUE ("T button?") TRUE ("T button?") TRUE ("T button?") TRUE ("T button?") w2949] -> w2934
                    tunnel: [w2937 w2939 w2941 w2943 w2945 w2948] -> w2932
                    tunnel: w2931 -> [w2937 w2939 w2941 w2943 w2945 w2947]
                    frame "Save file" {
                    }
                    frame "Edit values per row" {
                    }
                    frame "Edit Values with constants" {
                    }
                    frame "Edit Raw Data file header" {
                    }
                    frame "Post Process Plotted Rows" {
                    }
                    frame "Delete unwanted rows" {
                      n1323 = Array Size(array=w2952) -> (size(s)=w2951:i32)
                      n1324 = case shown="False" w2947 {
                        tunnel: w2951 -> [w2961 _]
                        tunnel: w2950 -> [w2960 _]
                        tunnel: [w2955 w2968] -> w2949
                        tunnel: [w2954 w2968] -> w2948
                        frame False {
                          n1325 = Format Into String(format string="Remove %d rows from \"%s\"", w2961, w2960) -> (resulting string=w2958:string)  [unwired: 2 in, 1 out]
                          n1326 = call <vilib>:"Three Button Dialog.vi"("Allow user to close window? (TRUE)"=TRUE, "Right Button Text (\"Cancel\")"="Yes To All Files" ("Right Button Text (\"Cancel\")"), "message"=w2958) -> ("Which Button?"=w2956:T11)  [unwired: 3 in, 5 out]
                          n1327 = case shown="\"Left Button\"" w2956 {
                            tunnel: [TRUE TRUE w2966 w2967] -> w2955
                            tunnel: [FALSE TRUE w2966 w2967] -> w2954
                            frame "Left Button" {
                            }
                            frame "Right Button" {
                            }
                            frame "Center Button" {
                              w2966 = FALSE
                            }
                            frame "Window Close" {
                              w2967 = FALSE
                            }
                          }
                        }
                        frame True {
                          w2968 = TRUE
                        }
                      }
                    }
                  }
                }
                frame #2 {
                  n1328 = case shown="True" w2984 {
                    tunnel: w2986 -> [_ w3005]
                    tunnel: w2985 -> [_ w3004]
                    tunnel: w2983 -> [_ w3003]
                    tunnel: w2982 -> [_ w3002]
                    tunnel: w2981 -> [_ w3001]
                    tunnel: w2980 -> [_ w3000]
                    tunnel: w2979 -> [_ w2999]
                    tunnel: w2978 -> [_ w2998]
                    tunnel: w2977 -> [_ w2997]
                    tunnel: w2976 -> [_ w2996]
                    tunnel: w2975 -> [_ w2995]
                    tunnel: w2974 -> [w2988 w2994]
                    tunnel: [w2988 w2993] -> w2973
                    tunnel: w2972 -> [w2987 w2992]
                    tunnel: [w2987 w2991] -> w2971
                    tunnel: w2970 -> [_ w2990]
                    tunnel: w2969 -> [_ w2989]
                    frame False {
                    }
                    frame True {
                      n1329 = case shown="\"Edit Raw Data file header\", Default" w3003 {
                        tunnel: w3005 -> [w3011 w3017 w3035 w3048 w3065]
                        tunnel: w3004 -> [w3014 w3024 w3034 w3047 w3064]
                        tunnel: w3002 -> [_ _ _ _ _]
                        tunnel: w3001 -> [_ _ _ w3045 w3062]
                        tunnel: w3000 -> [_ _ _ w3043 w3060]
                        tunnel: w2999 -> [_ _ _ _ w3059]
                        tunnel: w2998 -> [_ _ _ _ w3057]
                        tunnel: w2997 -> [_ _ _ _ w3056]
                        tunnel: w2996 -> [_ _ _ w3042 w3054]
                        tunnel: w2995 -> [_ _ _ w3040 w3052]
                        tunnel: w2994 -> [w3013 w3021 w3033 w3038 w3050]
                        tunnel: [w3013 w3022 w3033 w3038 w3050] -> w2993
                        tunnel: w2992 -> [w3012 w3020 w3032 w3037 w3049]
                        tunnel: [w3012 w3018 w3032 w3037 w3049] -> w2991
                        tunnel: w2990 -> [w3010 _ _ _ _]
                        tunnel: w2989 -> [_ _ _ w3036 _]
                        frame "Save file" {
                          n1330 = Strip Path(path=w3011) -> (name=w3008:string)  [unwired: 1 out]
                          n1331 = call "Add_filename_suffix.vi"("Filename"=w3008, "Suffix to add"=".xls") -> ("Filename out"=w3006:string)  [unwired: 3 out]
                          n1332 = Build Path(base path=w3010, name or relative path=w3006) -> (appended path=w3009:path)
                          n1333 = call "Save_full_Res_rows.vi"("Selected Rows"=w3014, "Filename to write"=w3009, "Filename Orig"=w3011) -> ()  [unwired: 2 out]
                        }
                        frame "Edit Raw Data file header", Default {
                          n1334 = call "GetRawDataFilePaths.vi"("Results file or Folder"=w3017) -> ("RawDataFilePaths"=w3015:string[], "RowNumbers"=w3016:i32[])  [unwired: 9 in]
                          n1335 = for {
                            tunnel: w3015 -> [w3031]
                            tunnel: w3024 -> [w3025] mode=indexing
                            tunnel: [w3029] -> w3023 mode=indexing
                            tunnel: [w3028] -> w3019 mode=indexing
                            tunnel: w3017 -> [w3028]
                            tunnel: w3016 -> [w3027]
                            n1336 = Search 1D Array(1D array=w3027, element=w3025) -> (index of element=w3026:i32)  [unwired: 1 in]
                            n1337 = Index Array(array=w3031, index=w3026) -> (element=w3030:string)
                            n1338 = call "String_to_Pathname.vi"("Input String"=w3030) -> ("path"=w3029:path)
                          }
                          n1339 = Build Array (concatenate)(w3020, w3019) -> (w3018:path[])
                          n1340 = Build Array (concatenate)(w3021, w3023) -> (w3022:path[])
                        }
                        frame "Delete unwanted rows" {
                          n1341 = call "Delete_unwanted_rows.vi"("Selected Rows"=w3034, "Filename"=w3035) -> ()  [unwired: 1 out]
                        }
                        frame "Edit Values with constants" {
                          w3046 = TRUE  # Value  Constant?
                          n1342 = local read "Edit Raw Data Header Info"() -> (w3039:bool)
                          n1343 = local read "Edit Raw DF?"() -> (w3041:bool)
                          n1344 = Not(x=w3045) -> (.not. x?=w3044:bool)
                          n1345 = call "Add_Update_Values.vi"("Filename"=w3048, "Value  Constant?"=w3046, "Edit Raw data files?"=w3041, "New Chs In"=w3043, "Edit Raw Data Header Info"=w3039, "New Values In"=w3036, "Selected Rows"=w3047, "Edit all Rows?"=w3044, "Raw DF in Orig Pos?"=w3042, "Job Directory"=w3040) -> ()  [unwired: 1 in, 5 out]
                        }
                        frame "Edit values per row" {
                          w3051 = FALSE  # Edit Raw Data Header Info
                          w3063 = FALSE  # Value  Constant?
                          n1346 = for {
                            tunnel: w3060 -> [w3076] mode=indexing
                            tunnel: w3059 -> [w3075]
                            tunnel: [w3074] -> w3058 mode=indexing
                            n1347 = Search 1D Array(1D array=w3075, element=w3076) -> (index of element=w3074:i32)  [unwired: 1 out]
                          }
                          n1348 = for {
                            tunnel: w3058 -> [w3070]
                            tunnel: w3057 -> [w3069]
                            tunnel: w3056 -> [w3067] mode=indexing
                            tunnel: [w3066] -> w3055 mode=indexing
                            n1349 = Index Array(array=w3069, index (row)=w3067) -> (element=w3068:string[])  [unwired: 1 in]
                            n1350 = for {
                              tunnel: w3070 -> [w3073] mode=indexing
                              tunnel: w3068 -> [w3072]
                              tunnel: [w3071] -> w3066 mode=indexing
                              n1351 = Index Array(array=w3072, index=w3073) -> (element=w3071:string)
                            }
                          }
                          n1352 = Not(x=w3062) -> (.not. x?=w3061:bool)
                          n1353 = local read "Edit Raw DF?"() -> (w3053:bool)
                          n1354 = call "Add_Update_Values.vi"("Filename"=w3065, "Value  Constant?"=w3063, "Edit Raw data files?"=w3053, "New Chs In"=w3060, "Edit Raw Data Header Info"=w3051, "New Values In"=w3055, "Selected Rows"=w3064, "Edit all Rows?"=w3061, "Raw DF in Orig Pos?"=w3054, "Job Directory"=w3052) -> ()  [unwired: 1 in, 5 out]
                        }
                      }
                    }
                  }
                }
                frame #3 {
                  n1355 = Build Array (concatenate)(w3079, w3078) -> (w3077:i32[])
                }
              }
            }
          }
          frame #3 {
            n1356 = case shown="\"Post Process Plotted Rows\"" w3085 {
              tunnel: ["Create Selectors" w3095 "Initialise" ("t") w3154] -> w3087
              tunnel: w3086 -> [_ _ _ w3151]
              tunnel: w3084 -> [w3088 w3094 _ _]
              tunnel: w3083 -> [_ w3093 _ _]
              tunnel: w3082 -> [_ w3092 _ _]
              tunnel: w3081 -> [_ w3091 _ _]
              tunnel: w3080 -> [_ w3090 _ _]
              frame "Edit Raw Data file header" {
                n1357 = call "Edit_Raw_DF_Header.vi"("Selected files"=w3088) -> ()  [unwired: 15 out]
              }
              frame "Post Process Plotted Rows" {
                n1358 = stacked-sequence {
                  seq-local: [w3097 _ _] -> [_ w3121 _]
                  seq-local: [w3096 _ _] -> [_ _ w3146]
                  seq-local: [_ w3118 _] -> [_ _ w3145]
                  tunnel: [_ _ "Create Selectors"] -> w3095
                  tunnel: w3094 -> [_ _ w3148]
                  tunnel: w3093 -> [_ _ w3147]
                  tunnel: w3092 -> [_ w3120 _]
                  tunnel: w3091 -> [w3098 _ _]
                  tunnel: w3090 -> [_ w3117 _]
                  frame #0 {
                    n1359 = global read "Results_plotter_Global.vi" "Dispose"() -> (w3100:string[])
                    n1360 = for {
                      tunnel: w3100 -> [w3109] mode=indexing
                      shift-right: [w3105] -> w3097
                      shift-left: i32[] [] -> [w3107]
                      i -> [w3106]
                      n1361 = String Subset(string=w3109, length (rest)=1 ("length (rest)")) -> (substring=w3111:string)  [unwired: 1 out]
                      n1362 = Equal?(x="T", y=w3111) -> (x = y?=w3108:bool)
                      n1363 = case shown="False" w3108 {
                        tunnel: w3107 -> [w3115 w3116]
                        tunnel: [w3114 w3116] -> w3105
                        tunnel: w3106 -> [w3113 _]
                        frame False {
                          n1364 = Build Array (concatenate)(w3115, w3113) -> (w3114:i32[])
                        }
                        frame True {
                        }
                      }
                    }
                    n1365 = for {
                      tunnel: w3098 -> [w3104]
                      tunnel: w3097 -> [w3103] mode=indexing
                      tunnel: [w3102] -> w3096 mode=indexing
                      n1366 = Index Array(array=w3104, index=w3103) -> (element=w3102:string)
                    }
                    n1367 = local write "Post Process Plotted Data"(FALSE ("Post Process Plotted Data")) -> ()
                  }
                  frame #1 {
                    n1368 = global read "Results_plotter_Global.vi" "Precision"() -> (w3119:string[])
                    n1369 = for {
                      tunnel: w3121 -> [w3127]
                      tunnel: w3120 -> [w3123]
                      tunnel: w3119 -> [w3126]
                      tunnel: [w3125] -> w3118 mode=indexing
                      tunnel: w3117 -> [w3124] mode=indexing
                      n1370 = Index Array(array=w3123, index (row)=w3124) -> (element=w3122:string[])  [unwired: 1 in]
                      n1371 = for {
                        tunnel: w3127 -> [w3137] mode=indexing
                        tunnel: w3122 -> [w3139]
                        tunnel: w3126 -> [w3138]
                        tunnel: [w3131] -> w3125 mode=indexing
                        n1372 = Index Array(array=w3139, index=w3137) -> (element=w3130:string)
                        n1373 = Index Array(array=w3138, index=w3137) -> (element=w3129:string)
                        n1374 = Fract/Exp String To Number(string=w3130) -> (offset past number=w3135:i32, number=w3132:dbl)  [unwired: 3 out]
                        n1375 = String Length(string=w3130) -> (length=w3136:i32)
                        n1376 = Equal?(x=w3136, y=w3135) -> (x = y?=w3133:bool)
                        n1377 = Empty String/Path?(string/path=w3130) -> (empty?=w3134:bool)
                        n1378 = Compound Arithmetic op=AND(invert w3134, w3133) -> (w3128:bool)
                        n1379 = case shown="True" w3128 {
                          tunnel: w3129 -> [_ w3142]
                          tunnel: w3132 -> [_ w3143]
                          tunnel: [w3140 w3141] -> w3131
                          tunnel: w3130 -> [w3140 _]
                          frame False {
                          }
                          frame True {
                            n1380 = call "Number_2_string.vi"("precision"=w3142, "number"=w3143) -> ("String"=w3141:string)
                          }
                        }
                      }
                    }
                  }
                  frame #2 {
                    n1381 = Build Array (concatenate)(w3146, w3145) -> (w3144:string[][])
                    n1382 = call "Post_Process_Profile_Remote.vi"("Results Plotter Rows"=w3144, "Raw Data files to PP"=w3148, "Current Results filenames"=w3147) -> ()  [unwired: 1 out]
                  }
                }
              }
              frame "Delete unwanted rows" {
              }
              frame "Edit Values with constants", Default {
                n1383 = local read "nRows"() -> (w3153:i32)
                n1384 = Less?(x=w3153, y=w3151) -> (x < y?=w3152:bool)
                n1385 = case shown="True" w3152 {
                  tunnel: ["Create Selectors" "Initialise" ("t")] -> w3154
                  frame False {
                  }
                  frame True {
                  }
                }
              }
            }
          }
          frame #4 {
            n1386 = Current VI's Path() -> (path=w3157:path)
            n1387 = call "Bring_to_front.vi"("path"=w3157) -> ()
          }
        }
      }
      frame "End" {
        n1388 = local read "Template"() -> (w3159:path)
        n1389 = local read "Empty"() -> (w3160:bool)
        n1390 = call "Valid_Path.vi"("Filename"=w3159) -> ("Valid Path?"=w3158:bool)
        n1391 = case shown="True" w3160 {
          frame False {
          }
          frame True {
            n1392 = property on="Result files to read" class="Arr (strict)"("Index Values"=u32[] [0] ("Write Attribute")) -> ()  [unwired: 2 in, 2 out]
            n1393 = local write "Result files to read"(path[] [] ("Result files to read")) -> ()
            n1394 = local write "Empty"(FALSE ("Empty")) -> ()
          }
        }
        n1395 = case shown="False" w3158 {
          tunnel: w3161 -> [w3170 _]
          frame False {
            n1396 = local write "Template"(w3170) -> ()
          }
          frame True {
          }
        }
      }
      frame "Empty Results file array" {
        n1397 = local read "Template"() -> (w3172:path)
        n1398 = call "Valid_Path.vi"("Filename"=w3172) -> ("Valid Path?"=w3171:bool)
        n1399 = case shown="True" w3171 {
          tunnel: w3173 -> [w3182 _]
          frame False {
            n1400 = local write "Template"(w3182) -> ()
          }
          frame True {
          }
        }
        n1401 = property on="Result files to read" class="Arr (strict)"("Index Values"=u32[] [0] ("Write Attribute")) -> ()  [unwired: 2 in, 2 out]
        n1402 = local write "Result files to read"(path[] [] ("Result files to read")) -> ()
        n1403 = local write "Empty"(FALSE ("Empty")) -> ()
      }
      frame "Save Setup" {
        w3187 = "Current_Setup.xls" ("Setup filename")
        n1404 = local read "Create picture Vi Name"() -> (w3202:string)
        n1405 = local read "Additional X Values"() -> (w3208:dbl[])
        n1406 = local read "Additional Y Values"() -> (w3207:dbl[])
        n1407 = local read "Result files to read"() -> (w3210:path[])
        n1408 = local read "Output Filename"() -> (w3203:path)
        n1409 = local read "Multi Ordinate?"() -> (w3200:bool)
        n1410 = local read "Intensity Plot?"() -> (w3201:bool)
        n1411 = local read "Multi Ordinate"() -> (w3196:i32[])
        n1412 = local read "Filter Array"() -> (w3204:u16[])
        n1413 = local read "Transpose"() -> (w3209:bool)
        n1414 = local read "Template"() -> (w3188:path)
        n1415 = local read "Ordinate"() -> (w3206:u16)
        n1416 = local read "Filter Bins 2"() -> (w3197:i32[])
        n1417 = local read "Filter Bins 1"() -> (w3198:i32[])
        n1418 = local read "Absisca"() -> (w3205:u16)
        n1419 = call "Read_Write_Plot_Setup.vi"("Mode"=enum16{"Load", "Save"}."Load", "Setup filename"=w3187) -> ("Cluster 2"=w3211:T10)  [unwired: 1 in, 1 out]
        n1420 = Bundle By Name(cluster=w3211, "Result files to read"=w3210, "Template"=w3188, "Transpose"=w3209, "Additional X Values"=w3208, "Additional Y Values"=w3207, "Ordinate"=w3206, "Absisca"=w3205, "Filter Array"=w3204, "color and symbol"=TRUE, "Output Filename"=w3203, "Jpg Vi Name"=w3202, "Intensity Plot?"=w3201, "Multi Ordinate?"=w3200, "Filter Bins 1"=w3198, "Filter Bins 2"=w3197, "Multi Ordinate"=w3196) -> (w3199:T10)
        n1421 = local read "Save Setup"() -> (w3186:bool)
        n1422 = local read "stop"() -> (w3194:bool)
        n1423 = Not(x=w3194) -> (.not. x?=w3193:bool)
        n1424 = Path To String(path="Job Directory") -> (string=w3192:string)
        n1425 = call "Read_Write_Plot_Setup.vi"("Mode"=enum16{"Load", "Save"}."Save", "Setup filename"=w3187, "Cluster"=w3199) -> ()  [unwired: 2 out]
        n1426 = call "Read_Write_Template.vi"("Template File"=w3188, "Mode"=Global_mode."Write Global to File", "Single Value In"=w3192, "Data type"="Log Folder Name" ("Variable name")) -> ()  [unwired: 4 in, 8 out]
        n1427 = Select(t="Save to named setup file", s=w3186, f="Check modification dates?") -> (s? t:f=w3184:string)
      }
      frame "Save to named setup file" {
        w3218 = TRUE  # Save New File?
        n1428 = call "Save_current_setup.vi"("Save New File?"=w3218, "Setup File Type"=Setup_Filetype."Results File Plotter Setups") -> ()  [unwired: 4 out]
        n1429 = local write "Save Setup"(FALSE ("Save Setup")) -> ()
      }
    }
    "Current" <- w11
  }
